vi "United-main.vi"() -> ()   [LabVIEW 2022 SP3]
doc: "Main VI for HFEPR measurements in Field domain.\nProgram uses a tab control that divides user interface in 5 pages. First (status) page is to monitor status of instruments. Second (adjustment) page is to setup individual parameters of each instrument. Third (EPR measurement) page serves for execution of measurement. Fourth (script) page serves for generation of script that can be later loaded in measurement tab. Fifth (measurement review) page is to display previous measurements. The last (about) page contains quick start info for user."
uses:
  Datatypes/Connected modules.ctl
  Datatypes/Magnet controls.ctl
  Datatypes/Application tabs.ctl
  Datatypes/Servo controls.ctl
  Datatypes/THz parameters.ctl
  Datatypes/Measurement info.ctl
  Datatypes/experiment state.ctl
  Datatypes/SampleHolders.ctl
  Datatypes/Module selection.ctl
  Datatypes/Acquisition controls.ctl
  Subsystem modules/Lock-in module/ctl/MFLI parameters.ctl
  Subsystem modules/Temperature control module/ctl/Set temperature.ctl
  Datatypes/script polymorh line.ctl
  Datatypes/Instr Info.ctl
  Subsystem modules/Magnet module/ctl/RampingOutput.ctl
  Datatypes/Single servo status.ctl
  Subsystem modules/Servo drive module/ctl/Axis names.ctl
  Datatypes/Measurement type.ctl
  Datatypes/Rotator controls.ctl
  Subsystem modules/Sample rotator/ctl/Motion Properties.ctl
  Subsystem modules/Source meter/ctls/SMU settings.ctl
  Datatypes/TopStates.ctl
  Datatypes/XY measurement graph data.ctl
  Datatypes/Measurement mode.ctl
  <vilib>/Utility/sysdir.llb/System Directory Type.ctl
  Subsystem modules/Magnet module/ctl/MSG to magnet.ctl
  Subsystem modules/Magnet module/ctl/Magnet Orders.ctl
  Subsystem modules/Magnet module/ctl/SetField data.ctl
  Subsystem modules/Magnet module/ctl/Magnet mode public.ctl
  Subsystem modules/Servo drive module/ctl/Servo MSG.ctl
  Subsystem modules/Servo drive module/ctl/Servo commands.ctl
  Subsystem modules/Sample rotator/ctl/MSG to Rotator.ctl
  Subsystem modules/Sample rotator/ctl/Rotator commands.ctl
  Subsystem modules/Sample rotator/ctl/Positoin to set.ctl
  Subsystem modules/THz module/ctl/THz Message for module.ctl
  Subsystem modules/THz module/ctl/THz commands enum.ctl
  Subsystem modules/THz module/ctl/THz sweep parameters.ctl
  Subsystem modules/Lock-in module/ctl/MFLI_message for module.ctl
  Subsystem modules/Lock-in module/ctl/MFLI_command enum.ctl
  Subsystem modules/Lock-in module/ctl/MFLI_parameter and value.ctl
  Subsystem modules/Lock-in module/ctl/MFLI_node.ctl
  Subsystem modules/Temperature control module/ctl/MSG for VTI.ctl
  Subsystem modules/Temperature control module/ctl/TC commands.ctl
  Subsystem modules/Temperature control module/ctl/Set point.ctl
  Subsystem modules/Source meter/ctls/MSG to SMU.ctl
  Subsystem modules/Source meter/ctls/SMU Commands.ctl
  Subsystem modules/THz module/ctl/THz MW generator constants.ctl
  Subsystem modules/Magnet module/ctl/TM Revision.ctl
  Subsystem modules/Magnet module/ctl/Overall status.ctl
  Subsystem modules/Magnet module/ctl/Actual magnet state.ctl
  Subsystem modules/Magnet module/ctl/Magnet mode.ctl
  Subsystem modules/Magnet module/ctl/Cryostat temperature sensors.ctl
  Subsystem modules/Power monitor/PwrM status.ctl
  Subsystem modules/Source meter/ctls/SMU status.ctl
  Subsystem modules/Lock-in module/ctl/ACQ info.ctl
  <instrlib>/Zurich Instruments LabOne/Public/Data/ziTypeDemodSampleSingle.ctl
  <instrlib>/Zurich Instruments LabOne/Public/ziTypeHandle.ctl
  Subsystem modules/Temperature control module/ctl/TC sensors.ctl
  Subsystem modules/Servo drive module/ctl/Servo state.ctl
  Subsystem modules/Servo drive module/ctl/Servo variables.ctl
  Subsystem modules/Servo drive module/ctl/Servo constants.ctl
  Subsystem modules/Servo drive module/ctl/Status variable change.ctl
  Subsystem modules/Sample rotator/ctl/Rotator all.ctl
  Subsystem modules/Sample rotator/ctl/Axis status.ctl
  <vilib>/Utility/error.llb/Trim Whitespace One-Sided.vi
  Subsystem modules/Messenger service/MessengerLib.lvlib
  Subsystem modules/Magnet module/Magnet module.lvlib
  Subsystem modules/Servo drive module/Servo drive module.lvlib
  Subsystem modules/THz module/THz source modeule.lvlib
  Subsystem modules/Lock-in module/Lock-in module.lvlib
  Subsystem modules/Sample rotator/SampleRotator.lvlib
  <instrlib>/Zurich Instruments LabOne/Zurich Instruments LabOne.lvlib
  Subsystem modules/Temperature control module/Temperature controller.lvlib
  <userlib>/_OpenG.lib/variantconfig/variantconfig.llb/openg_variant_configuration_file.lvlib
  <vilib>/Utility/config.llb/NI_LVConfig.lvlib
  Subsystem modules/Source meter/Source meter.lvlib
  Subsystem modules/Power monitor/Power monitor.lvlib
panel:
  out "Instr status":T1 caption="Connected\ninstuments"
  out "Controls referencies":T2
  out "Tmp [K]":T3
  out "Busy":bool
  in  "Stop":bool
  out "Results":T5(array[cluster])
  out "Magnetic\nfield state":bool
  out "data time":timestamp
  out "New data":bool
  out "Data":dbl[](array[numeric])
  out "Instr control refs":refnum<vi>[](array[refnum])
  out "meas results":refnum<file>
  out "Tmp reched time":dbl format="%<%H:%M:%S>T"
  out "VTI tmp reached":bool
  out "Running experiment":bool
  out "Temperature log ref":refnum<file>
  out "round execution\ntime [ms]":u32
  out "loggersRef":refnum<file>
  in  "Tab Control":T6
  out "Drift[K/s]":dbl[](array[numeric])
  in  "Log folder":path=path "C:/HFEPR logs"
  in  "Disconnect":bool
  in  "Select module":T7
  out "Logger":string[](array[string])
  in  "Re-connect instruments":bool
  in  "System config file path":path=path "C:/Programs/Debug/HFEPR spectrometer SW 2024/Multi-HFEPR app/SystemData/config.ini"
  out "Instr info":T8 {"PwrMonitor"."Last update" format="%<%H:%M:%S>T"; "VTI"."Last update" format="%<%H:%M:%S>T"; "PMD"."Last update" format="%<%H:%M:%S>T"; "SMU"."Last update" format="%<%H:%M:%S>T"; "Servo"."Last update" format="%<%H:%M:%S>T"; "Rotator"."Axes"."Actuator" items=["Linear", "Roatator", "Goniometer"]; "Rotator"."Name" items=["ANC350res", "ANC350num", "ANC350fps", "Unknown"]; "Rotator"."Last update" format="%<%H:%M:%S>T"; "THz"."Last update" format="%<%H:%M:%S>T"; "MFLI"."Last update" format="%<%H:%M:%S>T"; "Magnet"."Last update" format="%<%H:%M:%S>T"}
  in  "Use previous settings":bool=TRUE
  out "Temperature monitor":T12(graph)
  in  "Operation mode":bool=TRUE
  in  "SMU controls":T14={"Apply"=FALSE, "Measurement settings"={"Source Mode "=1, "Source Level"=0.1, "Source Limit"=0.21, "Measure Function"=0, "Remote sense"=TRUE, "Clear buffer?"=FALSE, "Beep"=TRUE, "High Capacity"=TRUE, "Terminals"=1, "PLCs"=4.0, "Fast measurement"=TRUE}, "Value"=0.1006, "Stop"=FALSE, "Record"=FALSE, "B[T]"=0.0, "Refresh"=FALSE} {"Value" format="%#_3e"; "Measurement settings"."Measure Function" items=["Volts", "Current", "Auto Resistance", "Manual Resistance", "Digitize Voltage", "Digitize Current"]; "Measurement settings"."Source Level" max=0.3; "Measurement settings"."Source Mode" items=["Voltage", "Current"]; "Measurement settings"."Terminals" items=["Front", "Rear"]}
  in  "Piezo controls":T15 {"Axes properties"."Amplitude [V]" min=0.0 max=60.0 step=1.0; "Axes properties"."DC voltage [V]" min=0.0 max=60.0 step=1.0; "Axes properties"."MaxErr [µm|m°]" min=1.0 max=1000.0 step=1.0; "Axes properties"."Frequency [Hz]" min=0.1 max=5000.0 step=10.0}
  in  "Password":string
  in  "VTI control":T17={"VTI space [K]"=1.0, "Sample [K]"=0.0, "Heater3 [K]"=1.8, "Heater4 [K]"=1.8, "Out 1 [%]"=0.0, "Out 2 [%]"=0.0, "Range out 1"=0} {"Range out 1" items=["Off", "Range 1 (On)", "Range 2", "Range 3", "Range 4", "Range 5"]; "Heater4 [K]" min=1.8 max=300.0; "Heater3 [K]" min=1.8 max=300.0; "Sample [K]" min=1.8 max=300.0; "VTI space [K]" min=1.8 max=300.0}
  in  "Acquisition controls":T18={"ACQ parameters"={"Filter order"=7.0, "Filter tau [ms]"=10.0, "F_Mod [kHz]"=1.0, "Amp_Mod [mV]"=10.0, "Enable output"=0, "Phase [°]"=0.0}, "ACQ shot btn"=FALSE, "Modulation [A]"=0.0, "In50"=FALSE, "Out50"=FALSE, "DemEn"=FALSE, "Actual [G]"=0.0, "Sample holder"=enum."Simple", "Desired [G]"=0.0, "Adj mod"=FALSE, "Auto-modulation"=TRUE, "Autorange"=FALSE, "AuxIn0 [V]"=0.0, "AuxIn1 [V]"=0.0} {"AuxIn1 [V]" format="%#_3g"; "AuxIn0 [V]" format="%#_3g"; "Desired [G]" format="%.1g"; "ACQ parameters"."Enable output" items=["Disable", "Enable"]; "ACQ parameters"."Amp_Mod [mV]" min=0.0 max=10000.0; "ACQ parameters"."F_Mod [kHz]" min=0.1 max=500.0; "ACQ parameters"."Filter order" min=1.0 max=9.0 step=1.0; "ACQ parameters"."Filter tau [ms]" min=0.0 max=1000.0}
  in  "THz control":T21={"AMC"=9, "Multip"=1, "Base frequency [GHz]"=82.0, "End frequency [GHz]"=0.0, "Im frequency [MHz]"=1885.0, "Sweep up [ms]"=0.0, "Reset trigger?"=FALSE} {"Multip" items=["1"=1, "2"=2, "3"=3, "4"=4, "6"=6, "8"=8, "9"=9]; "AMC" items=["9"=9, "12"=12]; "Base frequency [GHz]" format="%_5g"}
  in  "Servo controls":T22={"Y left"=FALSE, "Y right"=FALSE, "X backward"=FALSE, "X forward"=FALSE, "Zdown"=FALSE, "Zup"=FALSE, "Step\n[mm]"=5.0, "QO table"={"ZLdown"=FALSE, "ZLup"=FALSE, "ZRup"=FALSE, "ZRdown"=FALSE, "ZMdown"=FALSE, "ZMup"=FALSE}, "X"=0.0, "Y"=0.0, "ZL"=0.0, "ZR"=0.0, "ZM"=0.0, "Measure Position btn"=FALSE, "Eject position btn"=FALSE, "Stop servo btn"=FALSE, "Save position btn"=FALSE} {"Step\n[mm]" min=0.0 max=10.0 step=0.25}
  in  "Magnet controls":T23 {"Output\n[T]" scale=0.0..16.0; "Field\n[T]" scale=0.0..16.0; "Desired ramp\nrate [mT/s]" max=7.545; "Set Field [T]" min=0.0 max=16.0}
  out "lookup":cluster{"X (Vrms)":dbl, "Y (Vrms)":dbl}(graph) caption="Waveform Chart - Dark"
  in  "Create folder with date":bool
  in  "Operator":string
  in  "Save also backup":bool
  in  "Main data folder":path
  in  "Global comment":string
  in  "Sample name":string="Unknown"
  in  "Run script btn":bool
  in  "Direct stop meas. btn":bool
  out "Infobar":T24 {"Started" format="%<%H:%M:%S>T"; "Remains" format="%<%H:%M:%S>t"}
  out "Spectrum":cluster{dbl[], dbl[]}[](graph) caption="Live spectrum"
  in  "Paste from Editor":bool
  out "Actual measurement":T26={"Start"=nan, "Start Caption"="Start [T]", "End"=0.0, "End Caption"="End [T]", "Sweep"=0.0, "Sweep caption"="Rate [mT/s]", "Constant"=0.0, "Constant caption"="Freq [GHz]", "Mod_F [kHz]"=0.0, "Mod_A [G]"=0.0, "Tau [ms]"=0.0, "Positioners [mm|°]"=[], "Tmp [K]"=50.0, "Wait [min]"=0.0, "Carousel"=-1, "Comment"="", "Auto-mod"=TRUE, "Execute"=FALSE} {"Carousel" items=["0", "1", "2", "3", "4", "5", "6"]; "Positioners [mm|°]" min=-1.0 max=330.0; "Tau [ms]" min=0.002 max=10000.0; "Wait [min]" min=0.0 max=3000.0; "Tmp [K]" min=0.0 max=350.0; "Mod_A [G]" min=0.0 max=100.0; "Mod_F [kHz]" min=0.1 max=150.0}
  in  "Script Array":T26[](array[typedef]) {"Carousel" items=["0", "1", "2", "3", "4", "5", "6"]; "Positioners [mm|°]" min=-1.0 max=330.0; "Tau [ms]" min=0.002 max=10000.0; "Wait [min]" min=0.0 max=3000.0; "Tmp [K]" min=0.0 max=350.0; "Mod_A [G]" min=0.0 max=100.0; "Mod_F [kHz]" min=0.1 max=150.0}
  in  "Generator options":T27={"Tmp step [K]"=0.0, "Position [mm|°]"=[], "Freq step [GHz]"=0.0, "Append"=TRUE, "Iterate"=0}
  in  "Clear script btn":bool caption="Clear all script"
  in  "Set as adj tab btn":bool caption="Apply settings from\nadjustment tab"
  in  "Prototype line":T26={"Start"=0.0, "Start Caption"="Start [T]", "End"=0.0, "End Caption"="End [T]", "Sweep"=3.0, "Sweep caption"="Rate [mT/s]", "Constant"=100.0, "Constant caption"="Freq [GHz]", "Mod_F [kHz]"=3.01, "Mod_A [G]"=3.0, "Tau [ms]"=100.0, "Positioners [mm|°]"=[], "Tmp [K]"=5.0, "Wait [min]"=0.1, "Carousel"=0, "Comment"="", "Auto-mod"=TRUE, "Execute"=TRUE} {"Carousel" items=["0", "1", "2", "3", "4", "5", "6"]; "Positioners [mm|°]" min=-1.0 max=330.0; "Tau [ms]" min=0.002 max=10000.0; "Wait [min]" min=0.0 max=3000.0; "Tmp [K]" min=0.0 max=350.0; "Mod_A [G]" min=0.0 max=100.0; "Mod_F [kHz]" min=0.1 max=150.0}
  in  "Paste from meeasurrement":bool
  in  "Save script file btn":bool
  in  "Generate Script btn":bool caption="Generate Script"
  in  "Edited script":T26[](array[typedef]) caption="Script file name:" {"Carousel" items=["0", "1", "2", "3", "4", "5", "6"]; "Positioners [mm|°]" min=-1.0 max=330.0; "Tau [ms]" min=0.002 max=10000.0; "Wait [min]" min=0.0 max=3000.0; "Tmp [K]" min=0.0 max=350.0; "Mod_A [G]" min=0.0 max=100.0; "Mod_F [kHz]" min=0.1 max=150.0}
  in  "Remove from script btn":bool
  in  "Load script btn":bool
  in  "Select line":i32 min=0 max=10000
  in  "Save data btn":bool
  in  "Shift data btn":bool
  in  "Edit Channel":bool
  in  "Amlitude shift [-]":dbl
  in  "From point [T]":dbl
  out "Header":string[](array[string])
  out "Review Graph":cluster{"Array":dbl[], "Array":dbl[]}[](graph) caption="Header"
  in  "Open measurement":bool
  in  "Data file to show":u16(ring) items=["Empty", "Empty", "Empty", "Empty", "Empty", "Empty", "Empty", "Empty", "Empty", "Empty"]
  in  "Quick guide":T28(tab)
  # "Status part"
  # "Option 1:\nchoice primary and secondary sweep\n\nOption 2:\nChoice measurement mode, and appropriate cluster will apear. Other clusters wil be hidden.\n\n\nOption 3:\nChoice measurement mode.\nInternal parts of single cluster will (dis)apear if needed.\n\nNote:\nPosibility to do an orientation/temperature deppendency."
  # "Tmp [K]"
  # "Position [mm]"
  # "Z"
  # "X/Y"
  # "1.\tSelect module for subsystem, which is ready to operate. For CW measurements it is necessary to use subsystems: Magnet, VTI,\n THz sources and data acquisition (MFLI).\n2.\tClick on (Re)Connect button. Repeat for all subsystems that are ready and needed.\n3.\tWhen VTI and Magnet subsystems are connected, readings from temperature monitor and controller are displayed in graph.\n4.\tSuccessful connection to subsystem is indicated here.\n5.\tEvents on instruments are reported in this indicator.\n6.\tIf everything is OK, user may continue to another tab."
  # "1.\tFor CW experiments, magnet has to be in  ramping mode. (Magnet can be then pre-set to a start field.)\n2.\tCorrect multiplication factor need to be set manually by user.\n3.\tIntermediate frequency need to be set in in a middle of the range of band pass filters. \n4.\tTemperature of VTI can be also pre-set, while other settings are done (2 - 325 K).\n5.\tPosition of table in X axis should be about 900 mm. If table is not in measurement position, and there is no object in way, user can click on button Measure.\n6.\tIn control cluster for MFLI it is needed to enable output and set reasonable frequency and amplitude of modulation. After that click on Auto range button.\n7.\tIn case when sample rotator is used, user can check if rotator works correctly by setting desired position and press Go button.\n8.\tIn case when field sensor is used, it is required to setup current source, 100 mA, measure voltage, remote sense, rear terminals and press Apply button.\n9.\tIf series of measurement is going to be done, it is recommended to first setup measurement script in a script editor."
  # "1.\tLoad script from the Script editor tab. (overwrites current script in this tab)\n2.\tModify script if needed.\n3.\tSelect main folder, where data will be stored.\n4.\tFill name of a sample and operator that will be included in a file name.\n5.\tIf checked, save data in subfolder.\n6.\tTextbox for user to add any comment in header of data file.\n7.\tStart sequence of measurements in the script.\n8.\tContain brief information about measurement process.\n9.\tDisplays a raw spectrum.\n10.\tStop whole sequence.\n11.\tA standard graph tools."
  # "1.\tLoad actual settings of instruments and apply them to a prototype line.\n2.\tModify prototype line if needed.\n3.\tSet step for one (or more) parameter, and number of iterations.\n4.\tIf checked, append to a current scrip; else, overwrites.\n5.\tSave current script into text file (structured as configuration file) to load it later.\n6.\tModify generated script or manually fill a next line."
  # "1.\tLoad data from a file.\n2.\tRing for switching to previously loaded data.\n3.\tStandard graph tools (zoom, cursor).\n4.\tFeature to apply a simple data correction."
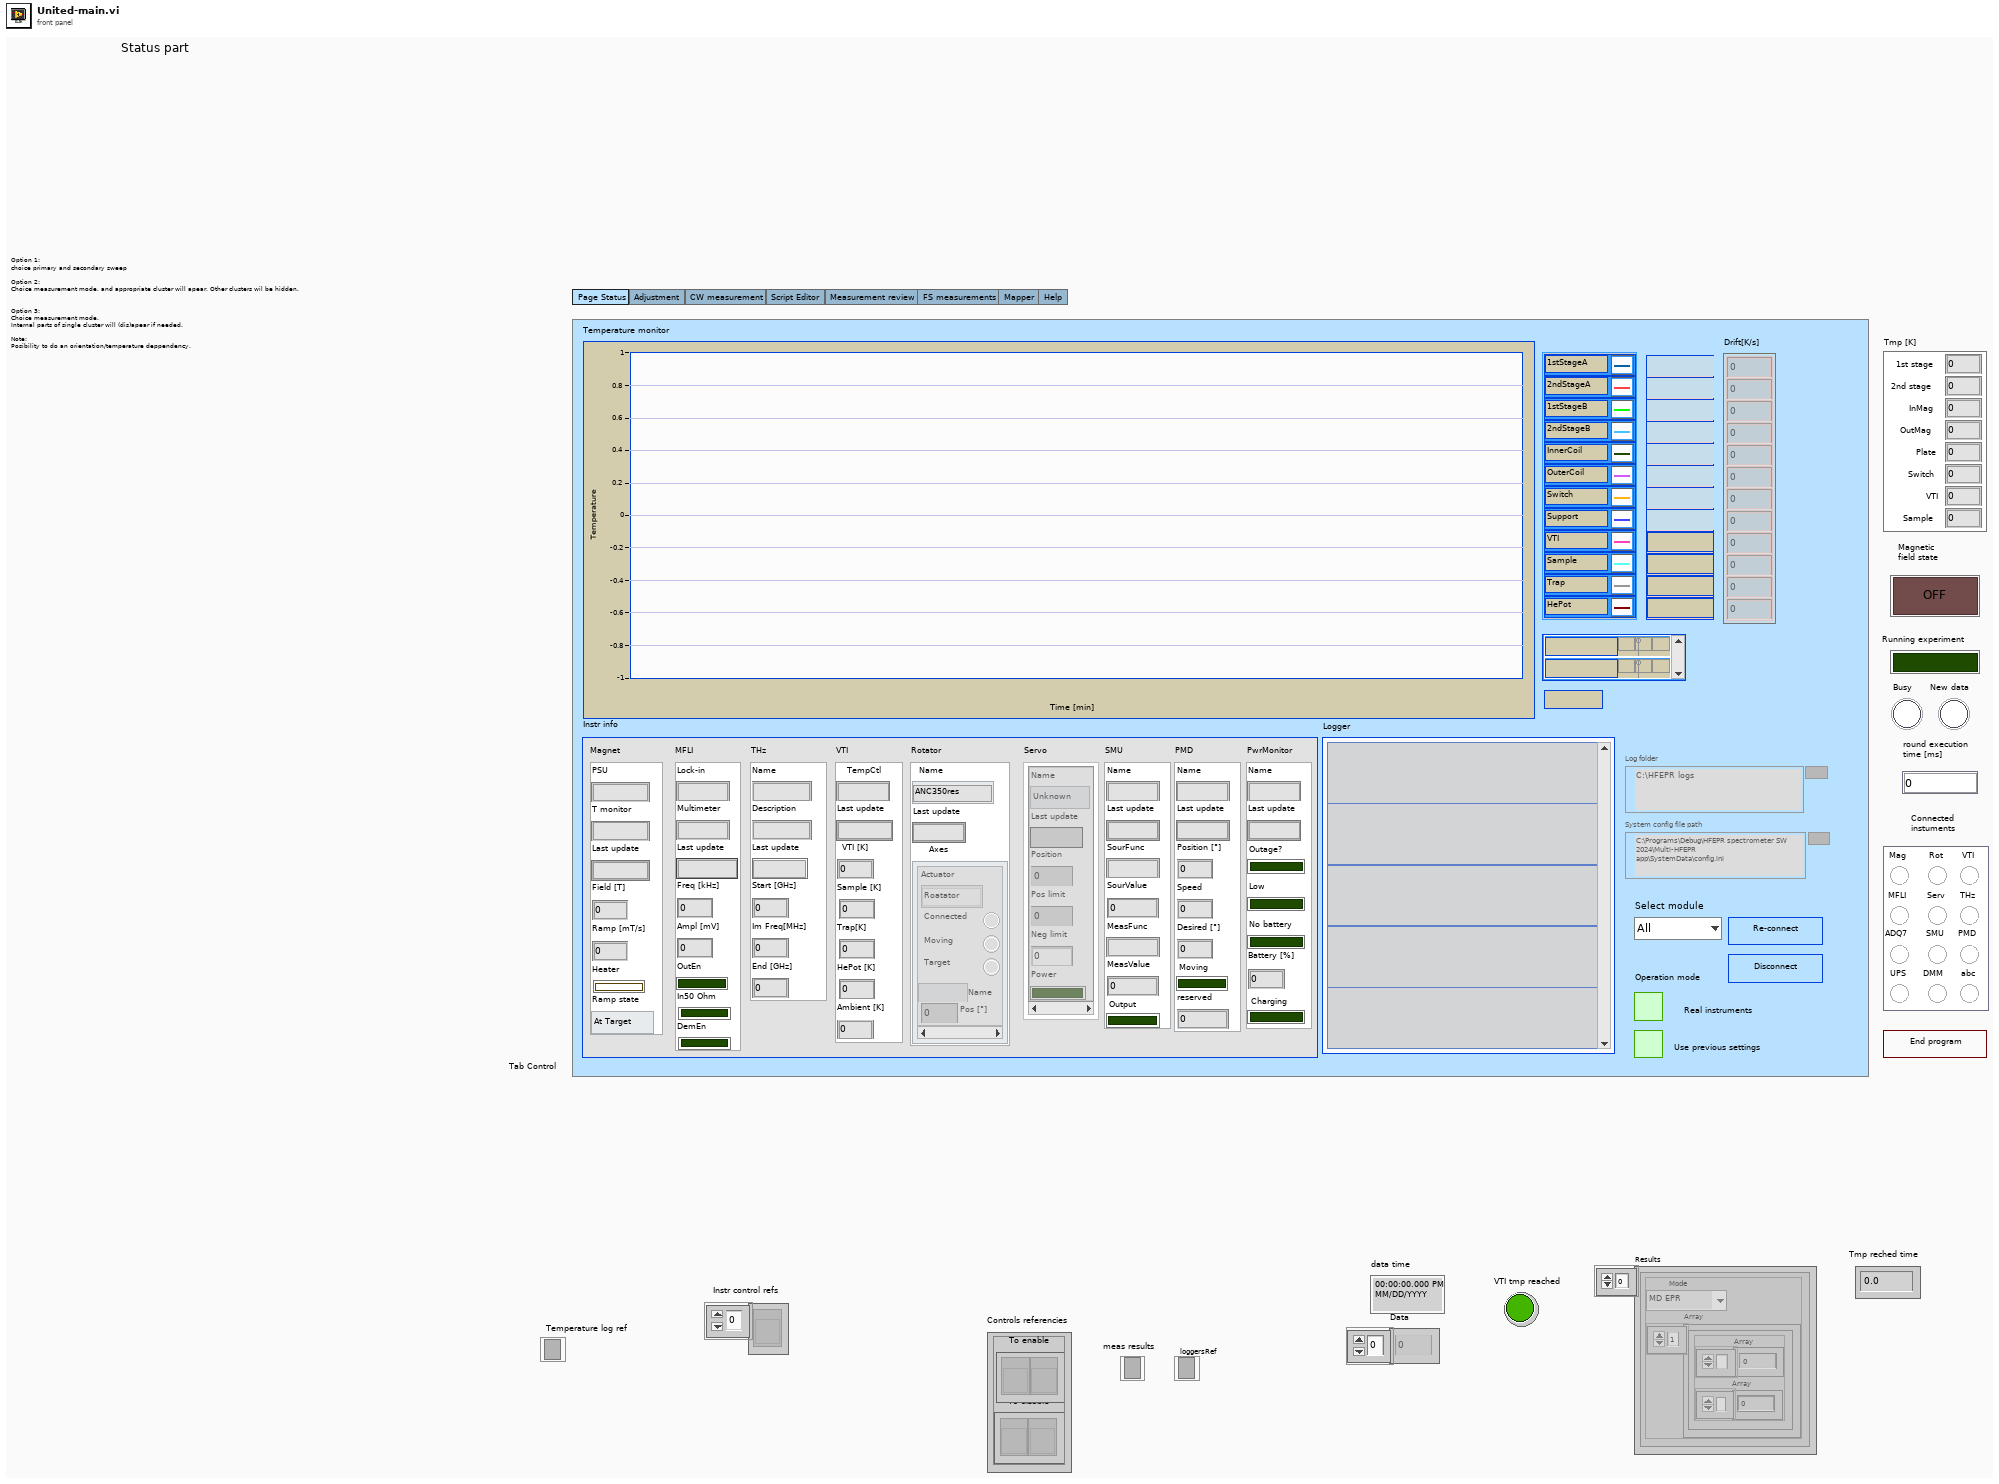
[diagram p1: front panel]
types:
  T1 = typedef "Connected modules.ctl" = cluster{"Mag":bool, "Rot":bool, "VTI":bool, "MFLI":bool, "Serv":bool, "THz":bool, "ADQ7":bool, "SMU":bool, "PMD":bool, "UPS":bool, "DMM":bool, "abc":bool}
  T2 = cluster{"To disable":refnum<vi>[], "To enable":refnum<vi>[]}
  T3 = cluster{"1st stage":dbl, "2nd stage":dbl, "InMag":dbl, "OutMag":dbl, "Plate":dbl, "Switch":dbl, "VTI":dbl, "Sample":dbl}
  T4 = typedef "Measurement type.ctl" = enum16{"MD EPR", "FD EPR"}
  T5 = cluster{"Mode":T4, "Array":cluster{"Array":dbl[], "Array":dbl[]}[]}[]
  T6 = typedef "Application tabs.ctl" = enum32{"Page Status", "Adjustment", "CW measurement", "Script Editor", "Measurement review", "FS measurements", "Mapper", "Help"}
  T7 = typedef "Module selection.ctl" = enum16{"All", "None", "ACQ", "THz", "MAG", "SERV", "ROT", "VTI", "SMU", "ADQ7", "PMD"}
  T8 = typedef "Instr Info.ctl" = cluster{"Magnet":cluster{"PSU":string, "T monitor":string, "Last update":timestamp, "Field [T]":dbl, "Ramp [mT/s]":dbl, "Heater":bool, "Ramp state":T9}, "MFLI":cluster{"Lock-in":string, "Multimeter":string, "Last update":timestamp, "Freq [kHz]":dbl, "Ampl [mV]":dbl, "OutEn":bool, "In50 Ohm":bool, "DemEn":bool}, "THz":cluster{"Name":string, "Description":string, "Last update":timestamp, "Start [GHz]":dbl, "Im Freq[MHz]":dbl, "End [GHz]":dbl}, "VTI":cluster{"TempCtl":string, "Last update":timestamp, "VTI [K]":dbl, "Sample [K]":dbl, "Trap[K]":dbl, "HePot [K]":dbl, "Ambient [K]":dbl}, "Rotator":cluster{"Name":i32, "Last update":timestamp, "Axes":cluster{"Pos [°]":dbl, "Moving":bool, "Name":string, "Actuator":u16, "Target":bool, "Connected":bool}[]}, "Servo":T10[], "SMU":cluster{"Name":string, "Last update":timestamp, "SourFunc":string, "SourValue":dbl, "MeasFunc":string, "MeasValue":dbl, "Output":bool}, "PMD":cluster{"Name":string, "Last update":timestamp, "Position [°]":dbl, "Speed":dbl, "Desired [°]":dbl, "Moving":bool, "reserved":dbl}, "PwrMonitor":cluster{"Name":string, "Last update":timestamp, "Outage?":bool, "Low":bool, "No battery":bool, "Battery [%]":u8, "Charging":bool}}
  T9 = typedef "Magnet module.lvlib/RampingOutput.ctl" = enum16{"At Target", "Go up", "Go down"}
  T10 = typedef "Single servo status.ctl" = cluster{"Name":T11, "Last update":timestamp, "Position":dbl, "Pos limit":dbl, "Neg limit":dbl, "Power":bool}
  T11 = typedef "Servo drive module.lvlib/Axis names.ctl" = enum16{"Unknown", "AxisX", "AxisY", "AxisZ_left", "AxisZ_middle", "AxisZ_right"}
  T12 = cluster{"[0]":dbl, "[1]":dbl, "[2]":dbl, "[3]":dbl, "[4]":dbl, "[5]":dbl, "[6]":dbl, "[7]":dbl, "[8]":dbl, "[9]":dbl, "[10]":dbl, "[11]":dbl}
  T13 = typedef "SMU settings.ctl" = cluster{"Source Mode ":u16, "Source Level":dbl, "Source Limit":dbl, "Measure Function":u16, "Remote sense":bool, "Clear buffer?":bool, "Beep":bool, "High Capacity":bool, "Terminals":u16, "PLCs":dbl, "Fast measurement":bool}
  T14 = cluster{"Apply":bool, "Measurement settings":T13, "Value":dbl, "Stop":bool, "Record":bool, "B[T]":dbl, "Refresh":bool}
  T15 = typedef "Rotator controls.ctl" = cluster{"Axes properties":T16[], "Rot set properties btn":bool, "Rot set position btn":bool, "Stop btn":bool, "Safe to \nmove?":bool}
  T16 = typedef "Motion Properties.ctl" = cluster{"Frequency [Hz]":dbl, "MaxErr [µm|m°]":dbl, "DC voltage [V]":dbl, "Amplitude [V]":dbl, "Position [mm|°]":dbl, "EoF":bool, "EoB":bool, "Error":bool, "Target [mm|°]":dbl}
  T17 = typedef "Temperature controller.lvlib/Set temperature.ctl" = cluster{"VTI space [K]":dbl, "Sample [K]":dbl, "Heater3 [K]":dbl, "Heater4 [K]":dbl, "Out 1 [%]":dbl, "Out 2 [%]":dbl, "Range out 1":u16}
  T18 = typedef "Acquisition controls.ctl" = cluster{"ACQ parameters":T19, "ACQ shot btn":bool, "Modulation [A]":dbl, "In50":bool, "Out50":bool, "DemEn":bool, "Actual [G]":dbl, "Sample holder":T20, "Desired [G]":dbl, "Adj mod":bool, "Auto-modulation":bool, "Autorange":bool, "AuxIn0 [V]":dbl, "AuxIn1 [V]":dbl}
  T19 = typedef "Lock-in module.lvlib/MFLI parameters.ctl" = cluster{"Filter order":dbl, "Filter tau [ms]":dbl, "F_Mod [kHz]":dbl, "Amp_Mod [mV]":dbl, "Enable output":u16, "Phase [°]":dbl}
  T20 = typedef "SampleHolders.ctl" = enum16{"Simple", "Carousel", "Chip", "Rotator", "Liquid"}
  T21 = typedef "THz parameters.ctl" = cluster{"AMC":u16, "Multip":u16, "Base frequency [GHz]":dbl, "End frequency [GHz]":dbl, "Im frequency [MHz]":dbl, "Sweep up [ms]":dbl, "Reset trigger?":bool}
  T22 = typedef "Servo controls.ctl" = cluster{"Y left":bool, "Y right":bool, "X backward":bool, "X forward":bool, "Zdown":bool, "Zup":bool, "Step\n[mm]":dbl, "QO table":cluster{"ZLdown":bool, "ZLup":bool, "ZRup":bool, "ZRdown":bool, "ZMdown":bool, "ZMup":bool}, "X":dbl, "Y":dbl, "ZL":dbl, "ZR":dbl, "ZM":dbl, "Measure Position btn":bool, "Eject position btn":bool, "Stop servo btn":bool, "Save position btn":bool}
  T23 = typedef "Magnet controls.ctl" = cluster{"Set Field [T]":dbl, "Desired ramp\nrate [mT/s]":dbl, "Custom\nramp":bool, "Mode switch":bool, "Pause ramp":bool, "Field\n[T]":dbl, "Output\n[T]":dbl, "Equalize":bool, "Discharge":bool, "Switch \ntmp [K]":dbl, "Direction":bool}
  T24 = typedef "Measurement info.ctl" = cluster{"Remains":dbl, "T_sample [K]":dbl, "Last log":string, "Experiment state":T25, "Field [T]":dbl, "Sample holder":T20, "Started":timestamp}
  T25 = typedef "experiment state.ctl" = enum16{"Setup", "Preparation", "Stabilization", "Begin", "Acquisition", "Save"}
  T26 = typedef "script polymorh line.ctl" = cluster{"Start":dbl, "Start Caption":string, "End":dbl, "End Caption":string, "Sweep":dbl, "Sweep caption":string, "Constant":dbl, "Constant caption":string, "Mod_F [kHz]":dbl, "Mod_A [G]":dbl, "Tau [ms]":dbl, "Positioners [mm|°]":dbl[], "Tmp [K]":dbl, "Wait [min]":dbl, "Carousel":i8, "Comment":string, "Auto-mod":bool, "Execute":bool}
  T27 = cluster{"Tmp step [K]":dbl, "Position [mm|°]":dbl[], "Freq step [GHz]":dbl, "Append":bool, "Iterate":u16}
  T28 = enum32{"Status", "Adjustment", "Measurement", "Script", "Viewer"}
  T29 = typedef "TopStates.ctl" = enum16{"Initialize GUI", "Wait for Event", "Check message", "Check measurement", "Stop", "Restart"}
  T30 = typedef "MessengerLib.lvlib/Messenger referencies.ctl" = cluster{"TOP":refnum<queue>, "Instr_M":refnum<queue>, "Field_C":refnum<queue>, "Tmp_M":refnum<queue>, "Tmp_C":refnum<queue>, "Table_C":refnum<queue>, "MW_C":refnum<queue>, "Data_Aq":refnum<queue>, "Mod_M":refnum<queue>, "Field_M":refnum<queue>, "Pwr_M":refnum<queue>, "Angle_C":refnum<queue>, "Sample_C":refnum<queue>, "Reserved":refnum<queue>}
  T31 = typedef "XY measurement graph data.ctl" = cluster{"Mode":T32, "Array":cluster{"Array":dbl[], "Array":dbl[]}[]}
  T32 = typedef "Measurement mode.ctl" = enum16{"MD EPR", "FD EPR", "EDMR", "EPR MAP"}
  T33 = enum8{"Enabled", "Disabled", "Disabled and Grayed Out"}
  T34 = typedef "Magnet module.lvlib/Magnet mode public.ctl" = enum16{"Persistant", "Ramping"}
  T35 = typedef "Magnet module.lvlib/SetField data.ctl" = cluster{"Field [T]":dbl, "Ramp [T/s]":dbl, "Custom Ramp?":bool, "Mode":T34}
  T36 = typedef "Magnet module.lvlib/Magnet Orders.ctl" = enum16{"Ignore", "Connect", "Update", "Switch mode", "Set field", "Stop ramping", "Equalize output", "Zero output", "Flip polarity", "Blackout", "Set timer", "Eval temperatures", "Disconnect"}
  T37 = typedef "Magnet module.lvlib/MSG to magnet.ctl" = cluster{"Command":T36, "Data":variant}
  T38 = typedef "Servo drive module.lvlib/Servo commands.ctl" = enum16{"Initialize", "Update", "Move by", "Move to", "Stop", "Ignore", "Disconnect", "End"}
  T39 = typedef "Servo drive module.lvlib/Servo MSG.ctl" = cluster{"Command":T38, "Data":variant}
  T40 = typedef "SampleRotator.lvlib/MSG to Rotator.ctl" = cluster{"Command":T41, "Data":variant}
  T41 = typedef "SampleRotator.lvlib/Rotator commands.ctl" = enum16{"Ignore", "Initialize", "Initialize axes", "Update", "Set parameters", "Stop movement", "Set position", "Disconnect", "End"}
  T42 = typedef "Positoin to set.ctl" = cluster{"Relative?":bool, "Position [°]":dbl, "Safe to move?":bool}
  T43 = typedef "THz source modeule.lvlib/THz commands enum.ctl" = enum16{"Ignore", "Connect", "Update", "Set parameters", "Disconnect", "End"}
  T44 = typedef "THz source modeule.lvlib/THz sweep parameters.ctl" = cluster{"Start [GHz]":dbl, "End [GHz] ":dbl, "Sweep up\ntime [ms]":dbl, "Sweep down\ntime [ms]":dbl, "Intermidiate [MHz]":dbl, "Reset trigger":bool}
  T45 = typedef "THz source modeule.lvlib/THz Message for module.ctl" = cluster{"Command":T43, "Data":variant}
  T46 = typedef "Lock-in module.lvlib/MFLI_parameter and value.ctl" = cluster{"parameter":T47, "value":dbl}
  T47 = typedef "Lock-in module.lvlib/MFLI_node.ctl" = enum16{"None", "filter_order [-]", "filter_constant [ms]", "in_diff", "in_autorange", "in_imp50", "in_AC", "osc_freq [kHz]", "out_ampl [V]", "out_autorange", "out_imp50", "enable output", "enamble ampl", "scope_enable", "scope_rate", "scope_len", "scope_trigEn", "AuxOut_amplify", "Phase_deg", "AuxOut_select"}
  T48 = typedef "Lock-in module.lvlib/MFLI_command enum.ctl" = enum16{"Initialize", "Update", "Set parameters", "Set module", "Set individual parameters", "Get point", "Get array", "Disconnect", "End", "Ignore"}
  T49 = typedef "Lock-in module.lvlib/MFLI_message for module.ctl" = cluster{"Command":T48, "Data":variant}
  T50 = typedef "Temperature controller.lvlib/Set point.ctl" = cluster{"Heater":string, "Tmp [K]":dbl}
  T51 = typedef "Temperature controller.lvlib/TC commands.ctl" = enum16{"Initialize", "Update", "Stop tmp change", "Set temperature", "Set point", "Disconnect", "End", "Ignore"}
  T52 = typedef "Temperature controller.lvlib/MSG for VTI.ctl" = cluster{"Command":T51, "Data":variant}
  T53 = typedef "Source meter.lvlib/MSG to SMU.ctl" = cluster{"Command":T54, "Data":variant}
  T54 = typedef "Source meter.lvlib/SMU Commands.ctl" = enum16{"Ignore", "Connect", "Update", "Set measurement", "Start measurement", "Get actual results", "Stop measurement", "Disconnect", "End"}
  T55 = cluster{"min synth f":dbl, "max synth f":dbl, "Ramp limits [mT/s]":dbl[], "Field ranges [T]":dbl[]}
  T56 = cluster{"Mode":T4, "Array":cluster{"Array":dbl[], "Array":dbl[]}[]}
  T57 = typedef "THz source modeule.lvlib/THz MW generator constants.ctl" = cluster{"Lower limit [GHz]":dbl, "Upper limit [GHz]":dbl, "Device name":string, "Connection":string, "Description":string, "Connected":bool, "Last settings":string, "Operation mode":enum16{"Disabled", "CW", "Arbitrary", "Sweep"}, "Enable ch 1":bool, "Enable ch 2":bool}
  T58 = typedef "Magnet module.lvlib/TM Revision.ctl" = cluster{"Instr Serial Number":string, "Instr Driver Revision":string, "Instr Firmware Revision":string, "Instr Model Number":string}
  T59 = typedef "Magnet module.lvlib/Overall status.ctl" = cluster{"Desired":T35, "Actual":T60}
  T60 = typedef "Magnet module.lvlib/Actual magnet state.ctl" = cluster{"Mode":T61, "Ramping output":T9, "Ready for change":bool, "Switch heater":bool, "Cooler Overheat":bool, "Coil overheat":bool, "Energized":bool, "Output [T]":dbl, "Field [T]":dbl, "Ramp[T/s]":dbl, "Switch\ntemperature [K]":dbl, "Voltage [V]":dbl, "Current direction":bool}
  T61 = typedef "Magnet module.lvlib/Magnet mode.ctl" = enum16{"Persistant", "Switching", "Ramping", "Quenched"}
  T62 = typedef "Magnet module.lvlib/Cryostat temperature sensors.ctl" = cluster{"First stage A [K]":dbl, "Second stage A [K]":dbl, "Firs stage B [K]":dbl, "Second stage B [K]":dbl, "Inner magnet [K]":dbl, "Outer Magnet [K]":dbl, "Switch [K]":dbl, "Support plate [K]":dbl, "Time stamp":dbl}
  T63 = typedef "Power monitor.lvlib/PwrM status.ctl" = cluster{"Name":string, "Last update":timestamp, "Outage?":bool, "Low":bool, "No battery":bool, "Battery [%]":u8, "Charging":bool}
  T64 = typedef "Source meter.lvlib/SMU status.ctl" = cluster{"VISA name":refnum<visa-resource-name>, "Connected":bool, "Name":string, "Message":string, "Error message":string, "Min voltage":dbl, "Max voltage":dbl, "Min Current":dbl, "Max Current":dbl, "Measurement value":dbl, "Source Voltage":dbl, "Measurement":bool, "Source Current":dbl, "Source Mode":u16, "Measure Function":u16}
  T65 = typedef "Lock-in module.lvlib/ACQ info.ctl" = cluster{"In50":bool, "InAC":bool, "InDiff":bool, "Out50":bool, "OutEN":bool, "OutF[Hz]":dbl, "OutA[V]":dbl, "DemEN":bool, "Const[ms]":dbl, "Order[-]":i32, "Phase [°]":dbl}
  T66 = enum32{"Page Status", "Adjustment", "EPR measurement", "About"}
  T67 = typedef "Zurich Instruments LabOne.lvlib/ziTypeDemodSampleSingle.ctl" = cluster{"Timestamps (ticks)":u64, "X (Vrms)":dbl, "Y (Vrms)":dbl, "Osc Phase (deg)":dbl, "Freq (Hz)":dbl, "DIO":u32, "AuxIn0 (V)":dbl, "AuxIn1 (V)":dbl, "Trigger":u32}
  T68 = typedef "Zurich Instruments LabOne.lvlib/ziTypeHandle.ctl" = cluster{"handleValid":bool, "Conn":u64, "Path Prefix":string, "Handle":u64, "Connected":bool, "Clockbase(s)":dbl}
  T69 = typedef "Temperature controller.lvlib/TC sensors.ctl" = cluster{"VTI space":dbl, "Sample":dbl, "He pot":dbl, "Trap":dbl, "Ambient":dbl, "SetP_VTI":dbl, "SetP_Smp":dbl, "SetP_Pot":dbl, "SetP_Trap":dbl, "Range out 1":u16, "Out 1 [%]":dbl, "Out 2 [%]":dbl}
  T70 = typedef "Servo drive module.lvlib/Servo state.ctl" = cluster{"Servo variables":T71, "Servo constants":T72, "Connection":variant}
  T71 = typedef "Servo drive module.lvlib/Servo variables.ctl" = cluster{"Terget reached":bool, "Connected":bool, "Power ON":bool, "Operation mode":bool, "Actual position":dbl, "Target position":dbl}
  T72 = typedef "Servo drive module.lvlib/Servo constants.ctl" = cluster{"Name":T11, "Pos position limit [mm]":dbl, "Neg position limit [mm]":dbl, "Pos velocity limit":dbl, "Neg velocity limit":dbl, "Acceleration limit":dbl}
  T73 = typedef "Servo drive module.lvlib/Status variable change.ctl" = cluster{"Property":string, "Value":variant, "Name":T11}
  T74 = typedef "SampleRotator.lvlib/Rotator all.ctl" = cluster{"Controller info":cluster{"deviceNumber":i32, "DeviceType":i32, "ID":u32, "Serial":string, "Address":string, "connected":bool}, "Handle":u64, "FW-Version":i32, "Features":u32, "Axes":T75[], "Path to DLL":path}
  T75 = typedef "SampleRotator.lvlib/Axis status.ctl" = cluster{"Axis status":cluster{"Connected":bool, "Enabled":bool, "Moving":bool, "Target":bool, "EndForward":bool, "EndBackarwd":bool, "Error":bool}, "Position [°]":dbl, "Frequency [Hz]":dbl, "Voltage [V]":dbl, "Capacitance[uF]":dbl, "Name":string, "ActuatorType":u16, "DC offset [V]":dbl, "Tolerance [m°]":dbl, "Index":u8}
  T76 = typedef "NI_LVConfig.lvlib/Config Data RefNum.ctl" = refnum<k1>
  T77 = typedef "System Directory Type.ctl" = i32
  T78 = typedef "lveventtype.ctl" = enum32{"Null", "Timeout", "Annotation Menu Selection", "Annotation Menu Selection?", "App Instance Close", "App Instance Close?", "Autoscale Range Change", "Bookmark Info Change", "Cell Edit", "Cell Edit?", "Cursor Grab", "Cursor Grab?", "Cursor Menu Selection", "Cursor Menu Selection?", "Cursor Move", "Cursor Release", "Data Change", "Direction Change", "Display State Change", "Drag Ended", "Drag Enter", "Drag Leave", "Drag Over", "Drag Source Update", "Drag Starting", "Drag Starting?", "Drop", "Exec State Change", "Key Down", "Key Down?", "Key Repeat", "Key Repeat?", "Key Up", "Listbox Double Click", "Menu Activation?", "Menu Selection (App)", "Menu Selection? (App)", "Menu Selection (User)", "Mouse Down", "Mouse Down?", "Mouse Enter", "Mouse Leave", "Mouse Move", "Mouse Up", "Mouse Wheel", "NI Security User Change (App)", "Pane Size", "Panel Close", "Panel Close?", "Panel Resize", "Plot Attribute Change", "Scale Range Change", "Shortcut Menu Activation?", "Shortcut Menu Selection (App)", "Shortcut Menu Selection? (App)", "Shortcut Menu Selection (User)", "Tree Double Click", "Tree Drag", "Tree Drag?", "Tree Drop", "Tree Drop?", "Tree Item Close", "Tree Item Close?", "Tree Item Open", "Tree Item Open?", "User Event", "Value Change"}
  T79 = typedef "Mudules status.ctl" = cluster{"Mag":bool, "Rot":bool, "VTI":bool, "MFLI":bool, "Serv":bool, "THz":bool, "ADQ7":bool, "SMU":bool, "PMD":bool, "UPS":bool, "DMM":bool, "abc":bool}
  T80 = typedef "Magnet module.lvlib/Magnet config constants.ctl" = cluster{"Switch resistant [K]":dbl, "Switch superconducting [K]":dbl, "First stage critical temperature [K]":dbl, "Second stage critical temperature [K]":dbl, "Inner magnet critical temperature [K]":dbl, "Outer magnet critical temperature [K]":dbl, "Field Constant [T/A]":dbl, "Maximum Current [A]":dbl, "Maximum field [T]":dbl, "Maximum source ramp [A/s]":dbl, "Source precision [T]":dbl, "Ramp limits [A/s]":dbl[], "Field limits [T]":dbl[], "SMS":refnum<visa-resource-name>, "LSC218":refnum<visa-resource-name>}
  T81 = typedef "MessengerLib.lvlib/MSG to TOP.ctl" = cluster{"Module":T82, "Response":string, "Data":variant, "Time":timestamp}
  T82 = typedef "Module name.ctl" = enum16{"Emty", "Magnet", "VTI", "Excitation", "Servo", "Acquisition", "Rotator", "Digitizer", "SMU2450", "Carousel", "Multimeter", "Tmp monitor", "Power monitor"}
  T83 = cluster{"PSU":string, "T monitor":string, "Last update":timestamp, "Field [T]":dbl, "Ramp [mT/s]":dbl, "Heater":bool, "Ramp state":T9}
  T84 = cluster{"TempCtl":string, "Last update":timestamp, "VTI [K]":dbl, "Sample [K]":dbl, "Trap[K]":dbl, "HePot [K]":dbl, "Ambient [K]":dbl}
  T85 = cluster{"Name":string, "Description":string, "Last update":timestamp, "Start [GHz]":dbl, "Im Freq[MHz]":dbl, "End [GHz]":dbl}
  T86 = cluster{"Name":string, "Last update":timestamp, "Outage?":bool, "Low":bool, "No battery":bool, "Battery [%]":u8, "Charging":bool}
  T87 = cluster{"Name":string, "Last update":timestamp, "SourFunc":string, "SourValue":dbl, "MeasFunc":string, "MeasValue":dbl, "Output":bool}
  T88 = cluster{"Lock-in":string, "Multimeter":string, "Last update":timestamp, "Freq [kHz]":dbl, "Ampl [mV]":dbl, "OutEn":bool, "In50 Ohm":bool, "DemEn":bool}
  T89 = cluster{"Name":i32, "Last update":timestamp, "Axes":cluster{"Pos [°]":dbl, "Moving":bool, "Name":string, "Actuator":u16, "Target":bool, "Connected":bool}[]}
  T90 = cluster{"Pos [°]":dbl, "Moving":bool, "Name":string, "Actuator":u16, "Target":bool, "Connected":bool}[]
  T91 = cluster{"Pos [°]":dbl, "Moving":bool, "Name":string, "Actuator":u16, "Target":bool, "Connected":bool}
  T92 = cluster{"deviceNumber":i32, "DeviceType":i32, "ID":u32, "Serial":string, "Address":string, "connected":bool}
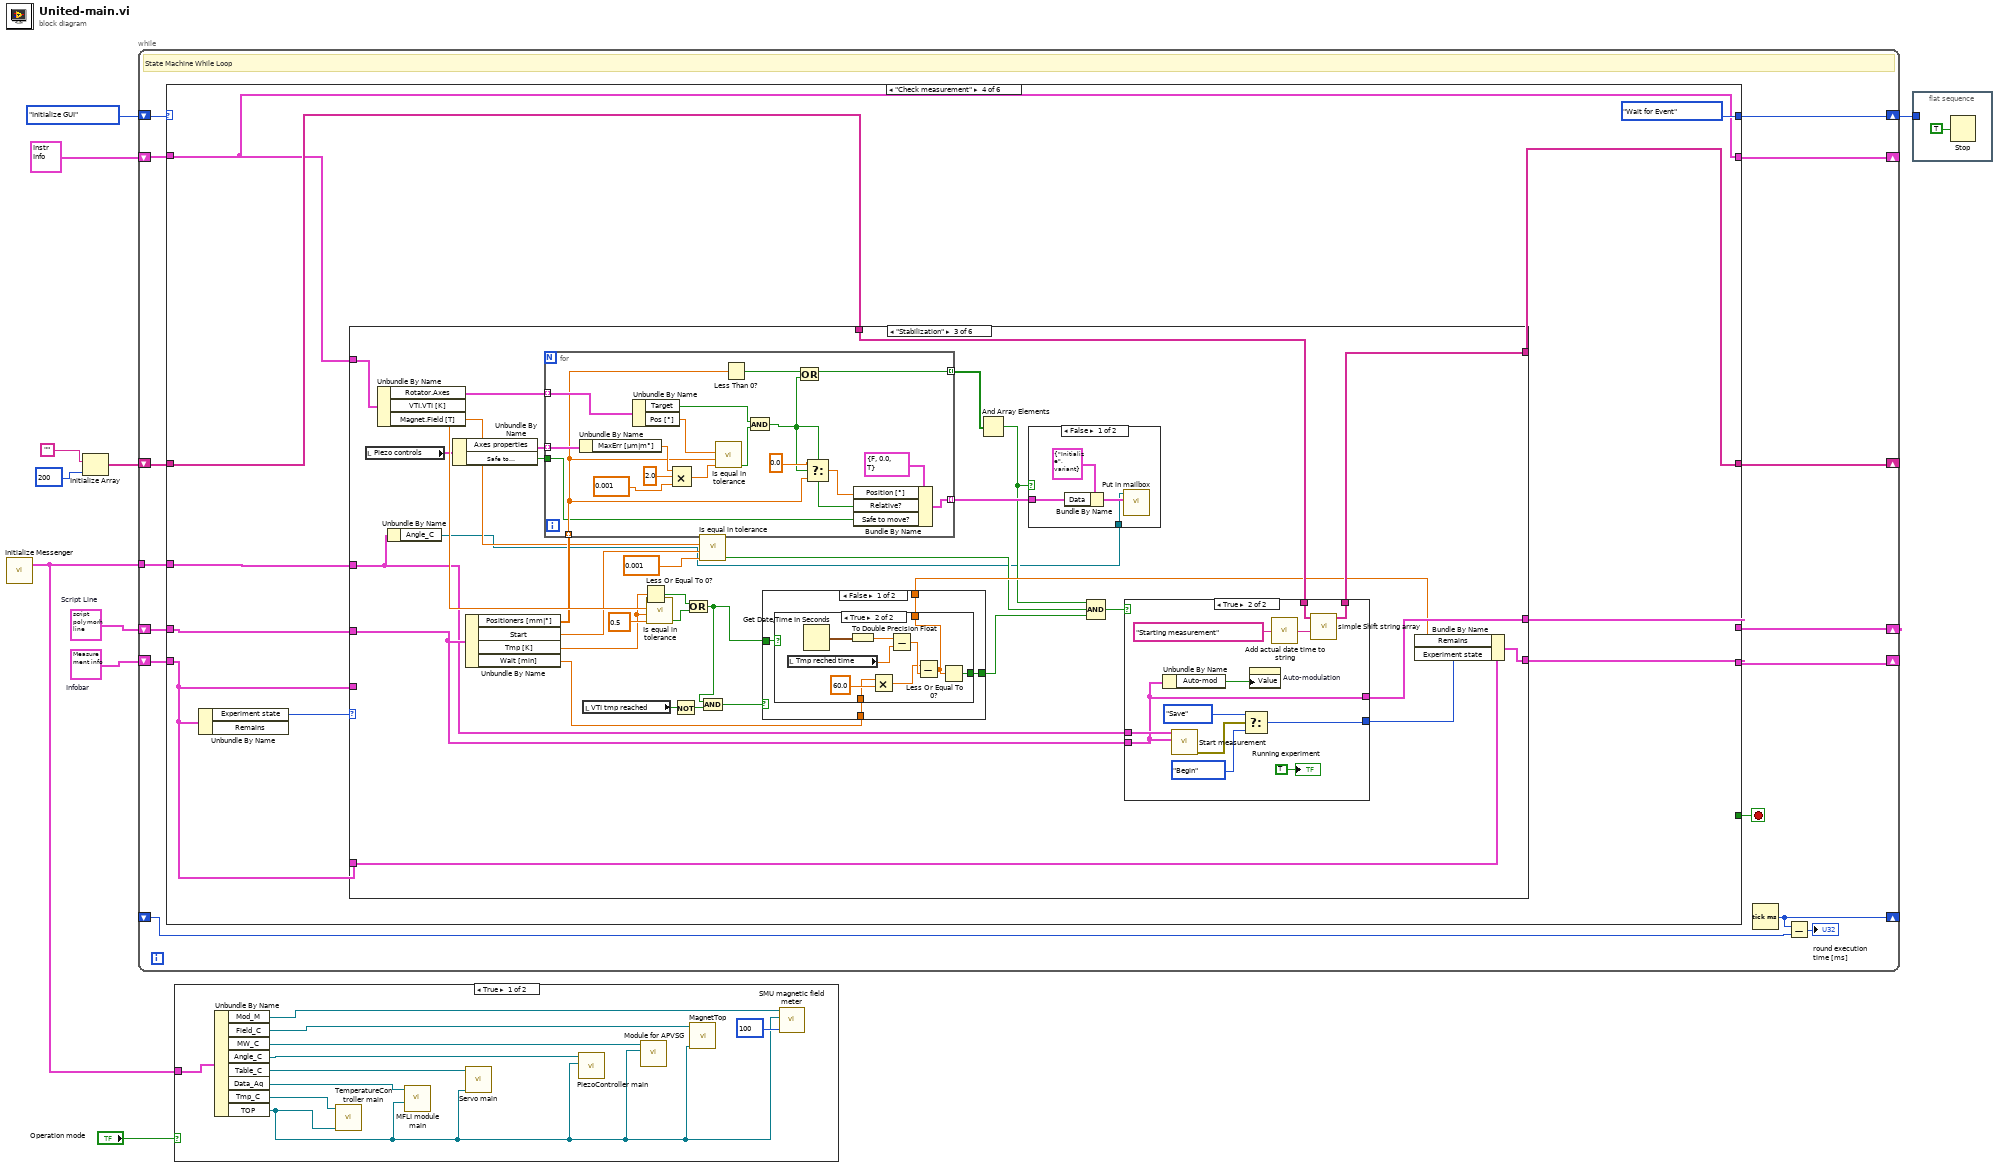
[diagram p0: block diagram]
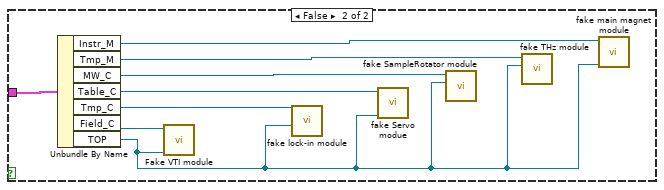
[diagram p2: hidden frame]
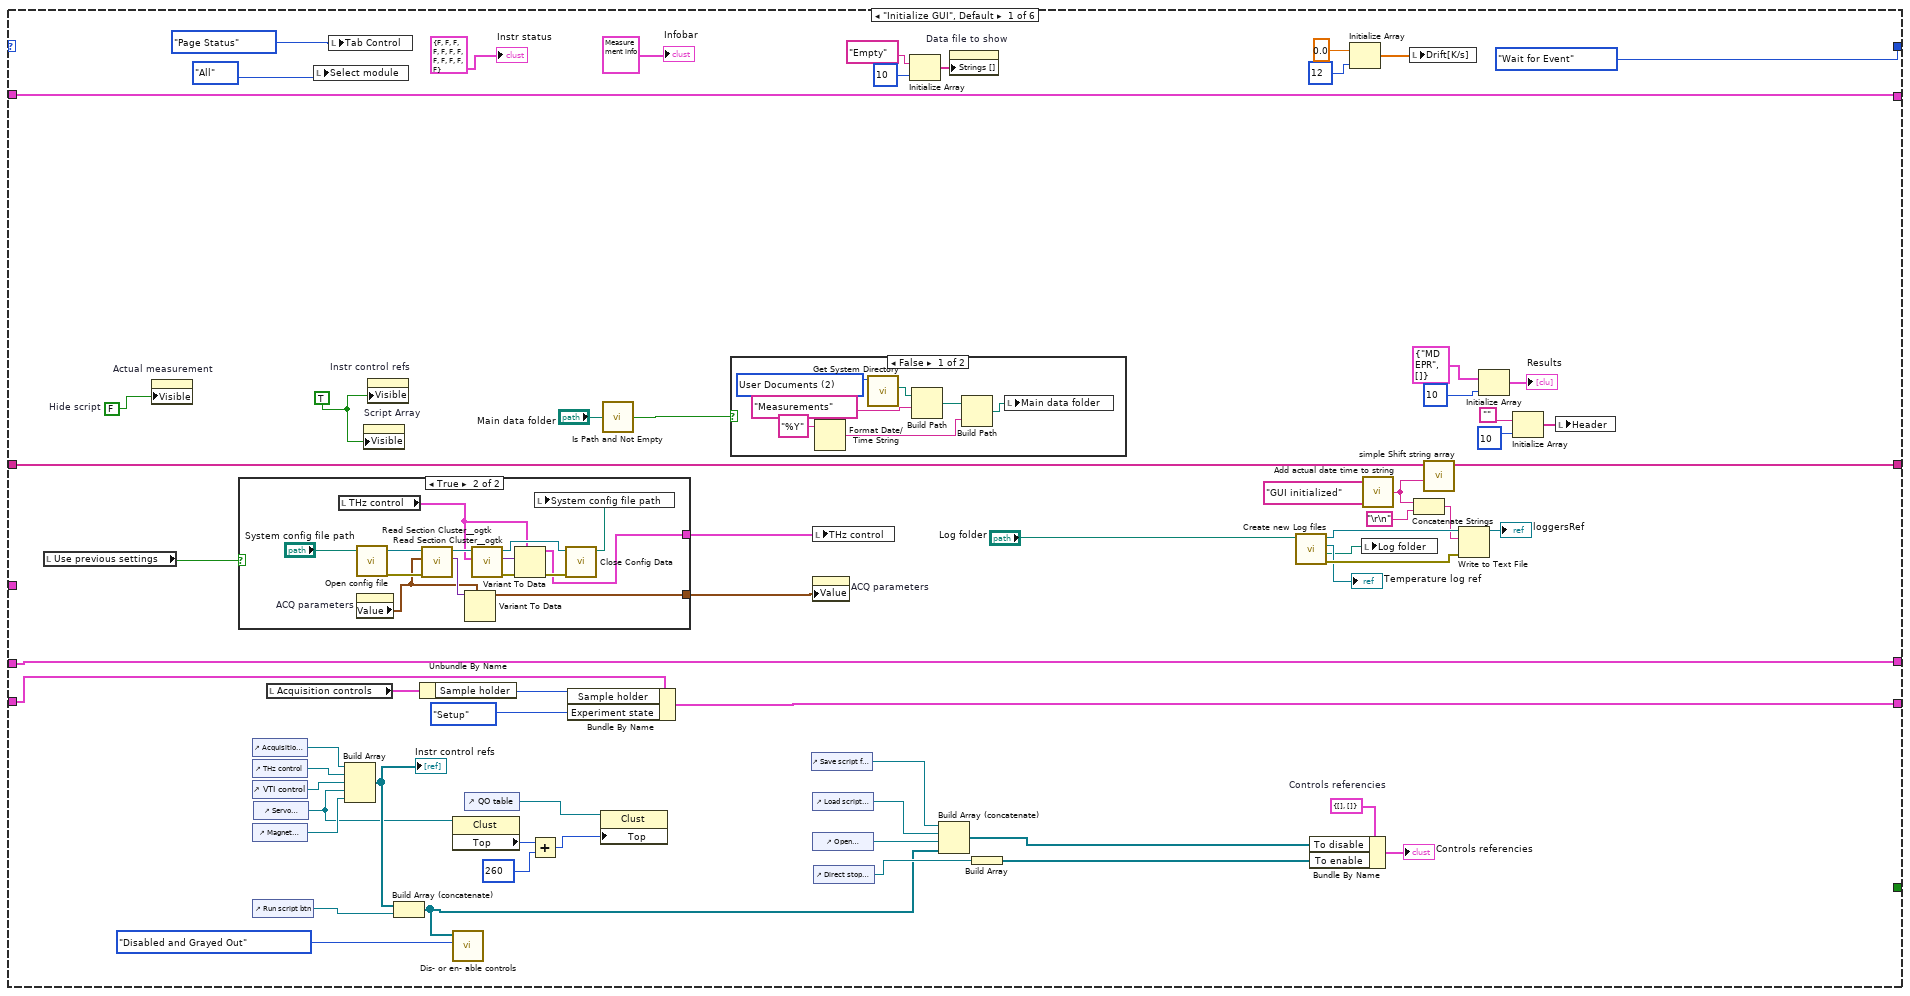
[diagram p3: hidden frame]
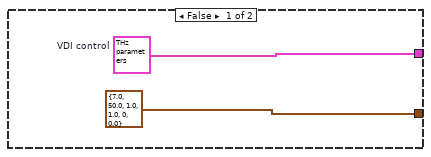
[diagram p5: hidden frame]
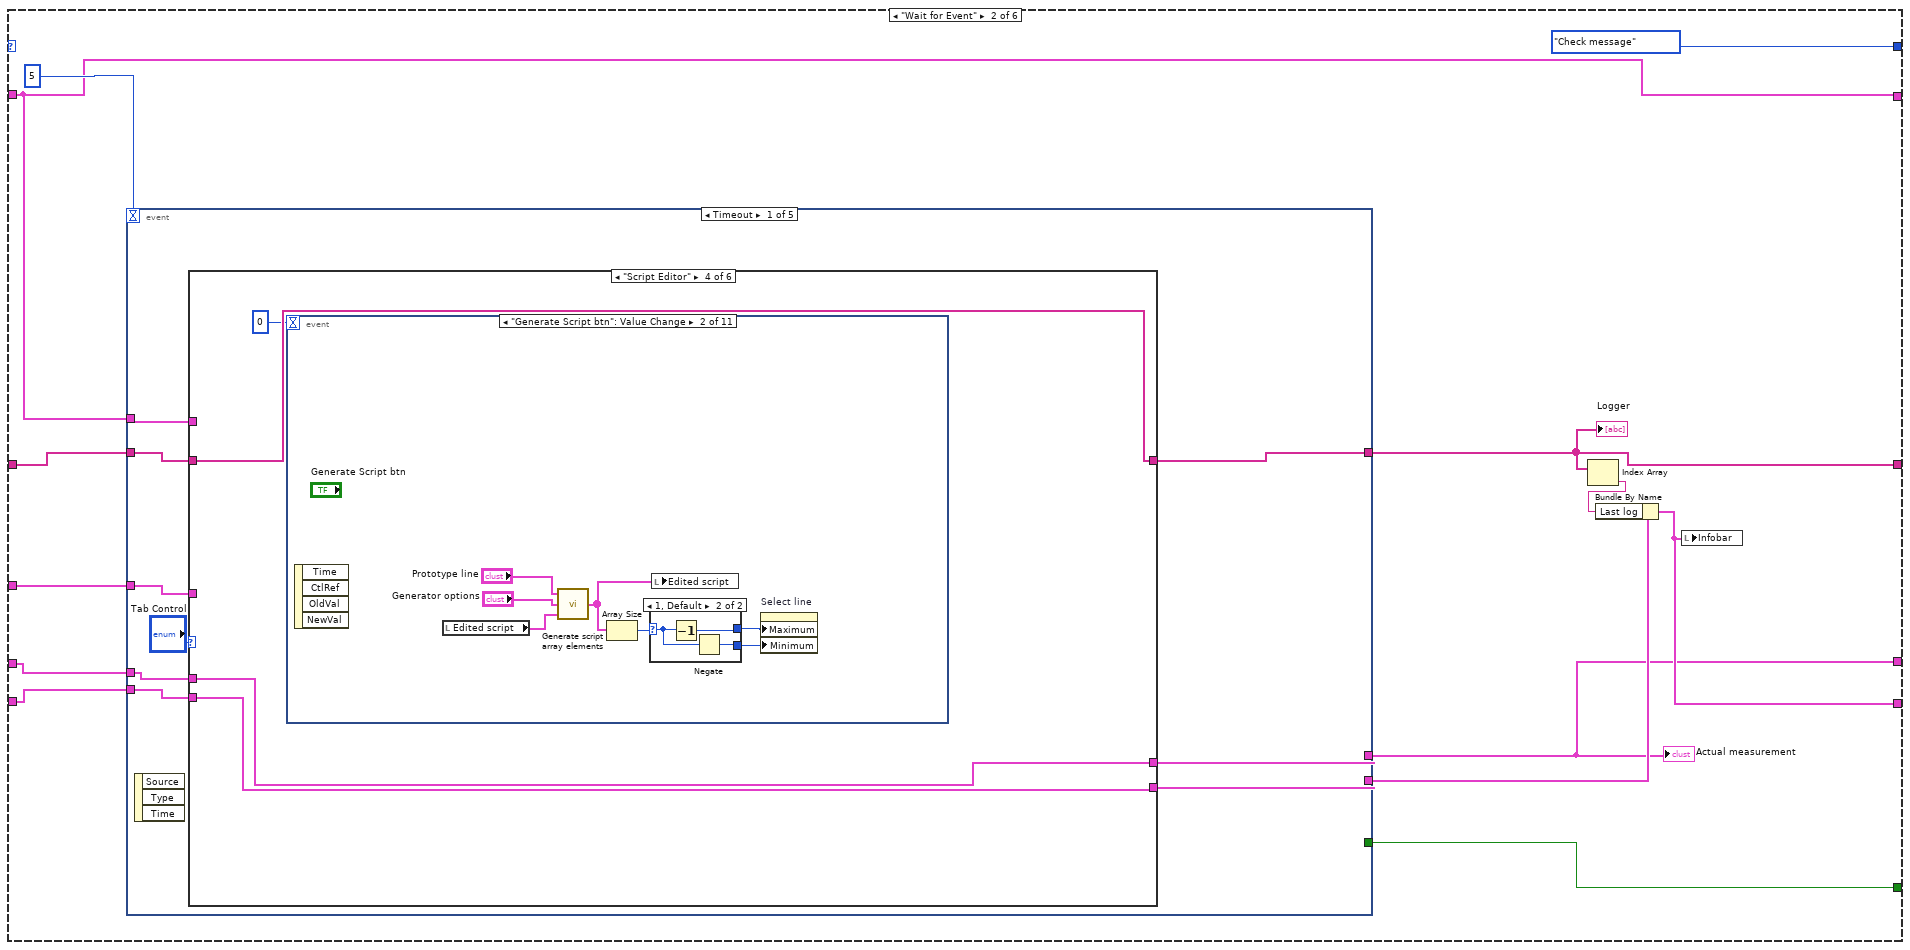
[diagram p6: hidden frame]
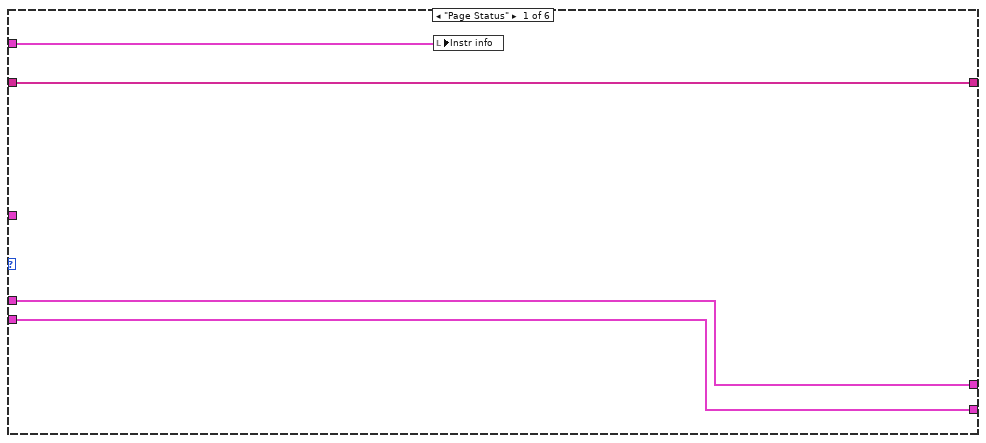
[diagram p7: hidden frame]
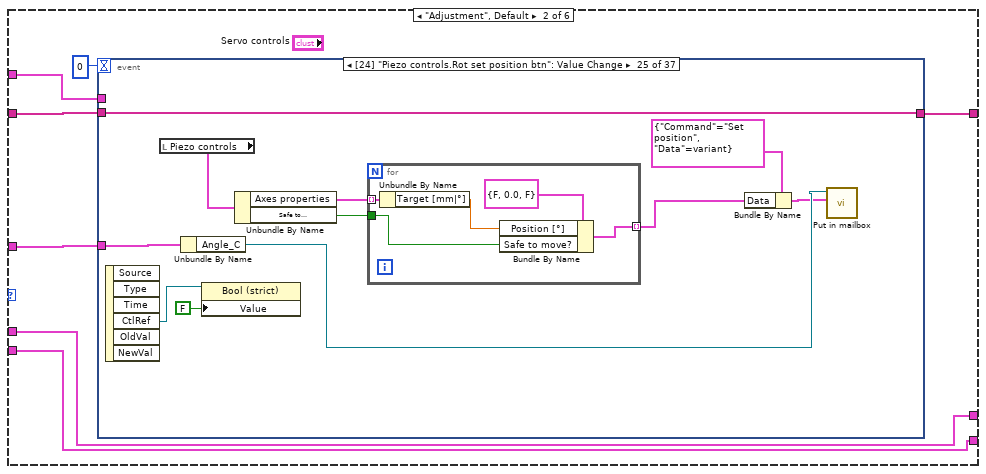
[diagram p8: hidden frame]
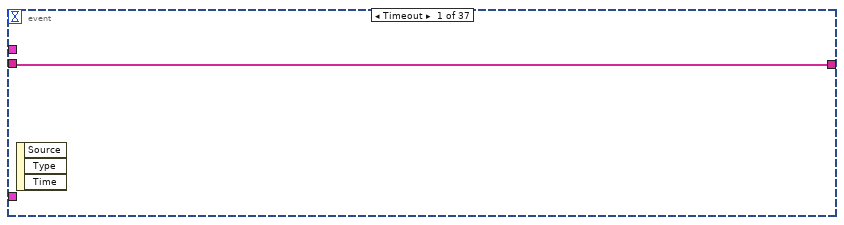
[diagram p9: hidden frame]
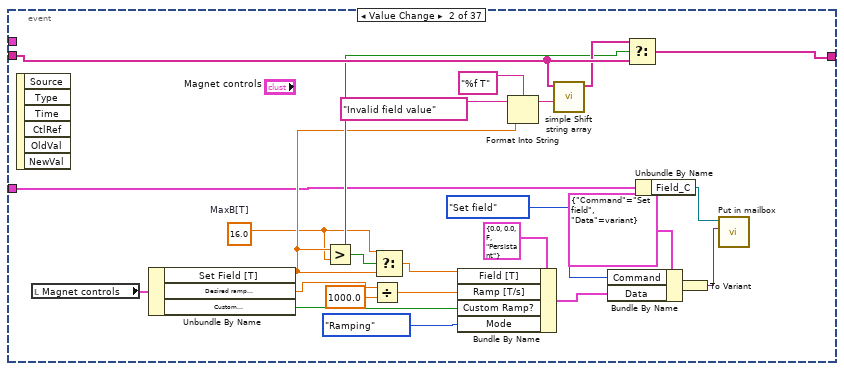
[diagram p10: hidden frame]
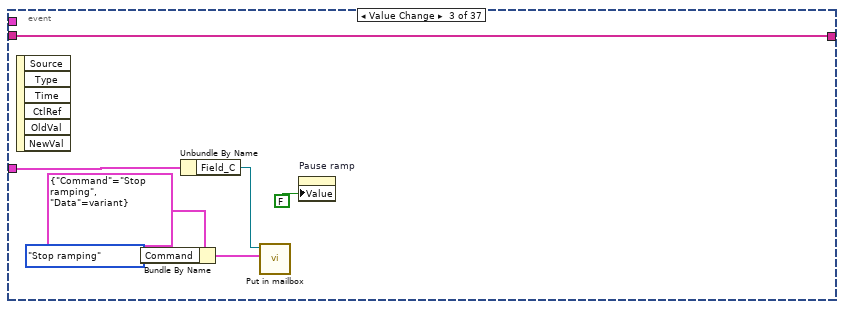
[diagram p11: hidden frame]
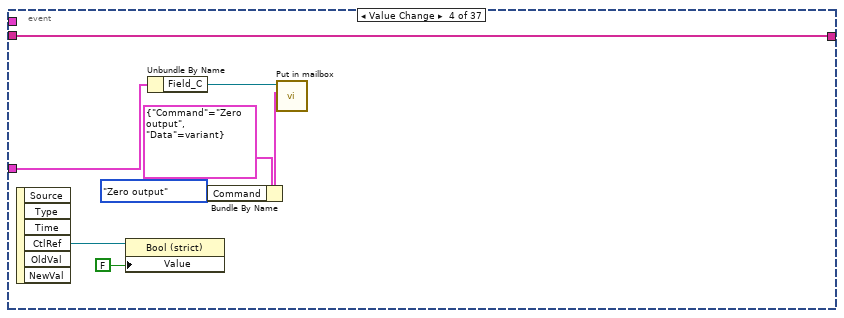
[diagram p12: hidden frame]
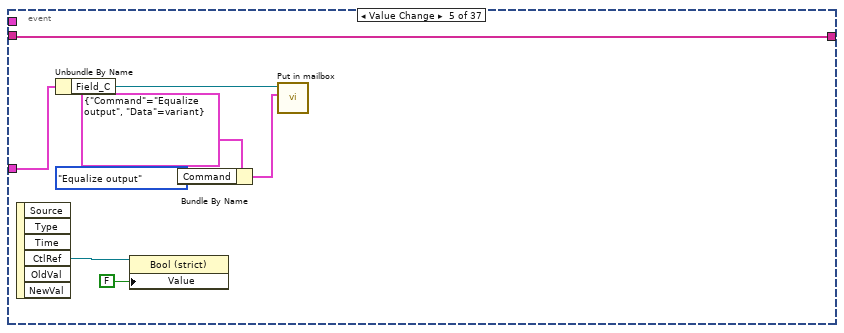
[diagram p13: hidden frame]
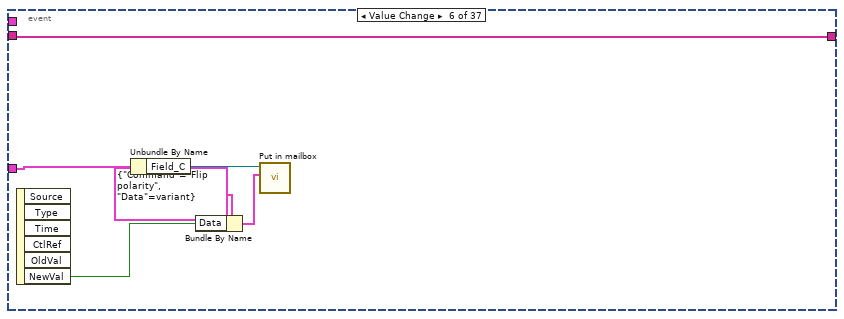
[diagram p14: hidden frame]
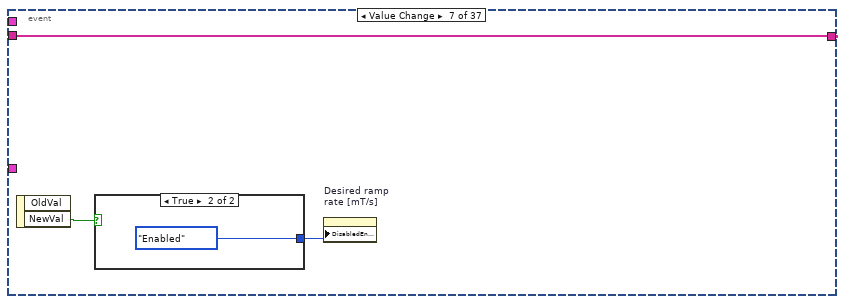
[diagram p15: hidden frame]
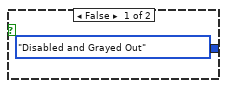
[diagram p16: hidden frame]
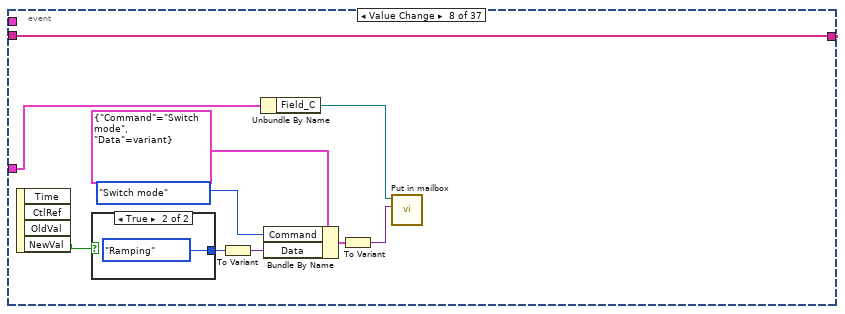
[diagram p17: hidden frame]
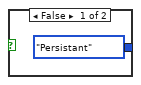
[diagram p18: hidden frame]
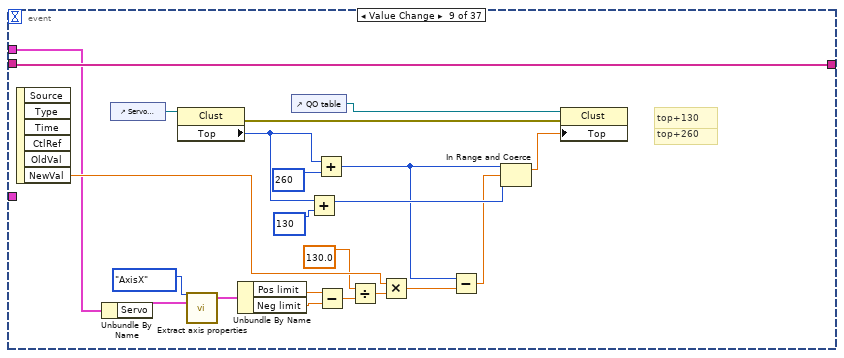
[diagram p19: hidden frame]
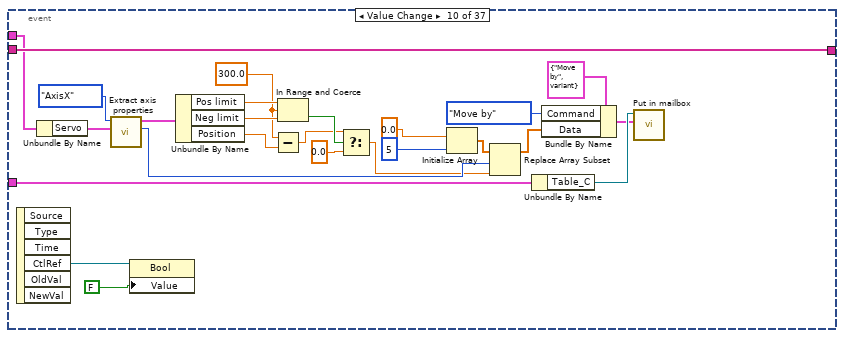
[diagram p20: hidden frame]
diagram:
  w1 = T26 {"Start"=nan, "Start Caption"="Start [T]", "End"=0.0, "End Caption"="End [T]", "Sweep"=0.0, "Sweep caption"="Rate [mT/s]", "Constant"=0.0, "Constant caption"="Freq [GHz]", "Mod_F [kHz]"=0.0, "Mod_A [G]"=0.0, "Tau [ms]"=0.0, "Positioners [mm|°]"=[], "Tmp [K]"=50.0, "Wait [min]"=0.0, "Carousel"=-1, "Comment"="", "Auto-mod"=TRUE, "Execute"=FALSE}  # Script Line
  w4 = T24 {"Remains"=0.0, "T_sample [K]"=1.6, "Last log"="", "Experiment state"=enum."Setup", "Field [T]"=0.0, "Sample holder"=enum."Simple", "Started"=timestamp(0 s since 1904-01-01)}  # Infobar
  n1 = call "Initialize Messenger.vi"() -> ("Referencies out"=w10:T30)  [unwired: 2 in, 1 out]
  n2 = Initialize Array("", 200 ("dimension size")) -> (w7:string[])
  n3 = while {
    tunnel: w10 -> [w25]
    shift-right: [w14] -> _
    shift-left: w7 -> [w24]
    shift-right: [w22] -> w5
    shift-left: TopStates."Initialize GUI" ("State") -> [w23]
    shift-right: [w20] -> _
    shift-left: _ -> [w19]
    shift-right: [w11] -> _
    shift-left: w1 -> [w17]
    shift-right: [w15] -> _
    shift-left: w4 -> [w16]
    shift-right: [w12] -> _
    shift-left: T8 {"Magnet"={"PSU"="None", "T monitor"="None", "Last update"=timestamp(0 s since 1904-01-01), "Field [T]"=0.0, "Ramp [mT/s]"=0.0, "Heater"=FALSE, "Ramp state"=enum."At Target"}, "MFLI"={"Lock-in"="None", "Multimeter"="None", "Last update"=timestamp(0 s since 1904-01-01), "Freq [kHz]"=0.0, "Ampl [mV]"=0.0, "OutEn"=FALSE, "In50 Ohm"=FALSE, "DemEn"=FALSE}, "THz"={"Name"="None", "Description"="None", "Last update"=timestamp(0 s since 1904-01-01), "Start [GHz]"=0.0, "Im Freq[MHz]"=0.0, "End [GHz]"=0.0}, "VTI"={"TempCtl"="", "Last update"=timestamp(0 s since 1904-01-01), "VTI [K]"=0.0, "Sample [K]"=0.0, "Trap[K]"=0.0, "HePot [K]"=0.0, "Ambient [K]"=0.0}, "Rotator"={"Name"=0, "Last update"=timestamp(0 s since 1904-01-01), "Axes"=[]}, "Servo"=[{"Name"=enum."Unknown", "Last update"=timestamp(0 s since 1904-01-01), "Position"=0.0, "Pos limit"=0.0, "Neg limit"=0.0, "Power"=FALSE}], "SMU"={"Name"="", "Last update"=timestamp(0 s since 1904-01-01), "SourFunc"="None", "SourValue"=0.0, "MeasFunc"="", "MeasValue"=0.0, "Output"=FALSE}, "PMD"={"Name"="", "Last update"=timestamp(0 s since 1904-01-01), "Position [°]"=0.0, "Speed"=0.0, "Desired [°]"=0.0, "Moving"=FALSE, "reserved"=0.0}, "PwrMonitor"={"Name"="", "Last update"=timestamp(0 s since 1904-01-01), "Outage?"=FALSE, "Low"=FALSE, "No battery"=FALSE, "Battery [%]"=0, "Charging"=FALSE}} ("Instr info") -> [w13]
    stop <- w21 stop-if-true
    # "State Machine While Loop"
    n4 = case shown="\"Check measurement\"" w23 {
      tunnel: w25 -> [_ w125 w1415 w2930 _ _]
      tunnel: w24 -> [w88 w124 w1429 w2929 w3218 _]
      tunnel: [w87 w113 w1428 w2928 w3217 w3223] -> w14
      tunnel: [TopStates."Wait for Event" ("State") TopStates."Check message" ("State") w1418 TopStates."Wait for Event" ("State") TopStates."Stop" ("State") TopStates."Initialize GUI" ("State")] -> w22
      tunnel: [_ w122 _ _ _ _] -> w21
      tunnel: [w74 w114 w1416 w2925 w3215 w3222] -> w11
      tunnel: w17 -> [w74 w120 w1416 w2926 w3215 w3222]
      tunnel: [w72 w115 w1417 w2927 w3214 w3221] -> w15
      tunnel: w16 -> [w73 w119 w1412 w2922 w3214 w3221]
      tunnel: w13 -> [w64 w116 w1414 w2923 w3213 w3220]
      tunnel: [w64 w116 w1413 w2923 w3213 w3220] -> w12
      frame "Initialize GUI", Default {
        w34 = FALSE  # Hide script
        w42 = T2 {"To disable"=[], "To enable"=[]}  # Controls referencies
        w63 = TRUE ("Visible")
        n5 = local read "Use previous settings"() -> (w57:bool)
        n6 = property on="Actual measurement" class="Clust (strict)"("Visible"=w34) -> ()  [unwired: 2 in, 2 out]
        n7 = case shown="True" w57 {
          tunnel: [w98 w100] -> w60
          tunnel: [T19 {"Filter order"=7.0, "Filter tau [ms]"=50.0, "F_Mod [kHz]"=1.0, "Amp_Mod [mV]"=1.0, "Enable output"=0, "Phase [°]"=0.0} ("ACQ parameters") w103] -> w54
          frame False {
            w98 = T21 {"AMC"=9, "Multip"=1, "Base frequency [GHz]"=90.0, "End frequency [GHz]"=90.0, "Im frequency [MHz]"=10.0, "Sweep up [ms]"=0.0, "Reset trigger?"=FALSE}  # VDI control
          }
          frame True {
            n8 = local read "THz control"() -> (w102:T21)
            n9 = call "Open config file.vi"("MAG config file path"="System config file path") -> ("error out"=w111:errorcluster, "Refnum out"=w112:T76)  [unwired: 7 in, 2 out]
            n10 = property on="ACQ parameters" class="Clust (strict)"() -> ("Value"=w101:T19)  [unwired: 2 in, 2 out]
            n11 = call <userlib>:"Read Section Cluster__ogtk.vi"("error in (no error)"=w111, "Section Formatted Cluster Type"=w101, "refnum"=w112) -> ("Section Formatted Cluster"=w110:variant, "dup refnum"=w107:T76)  [unwired: 4 in, 3 out]
            n12 = Variant To Data(type=w101, Variant=w110) -> (data=w103:T19)  [unwired: 1 in, 1 out]
            n13 = call <userlib>:"Read Section Cluster__ogtk.vi"("Section Formatted Cluster Type"=w102, "refnum"=w107) -> ("error out"=w109:errorcluster, "Section Formatted Cluster"=w108:variant, "dup refnum"=w106:T76)  [unwired: 5 in, 2 out]
            n14 = Variant To Data(error in=w109, type=w102, Variant=w108) -> (data=w100:T21, error out=w104:errorcluster)
            n15 = call <vilib>:"Close Config Data.vi"("error in (no error)"=w104, "refnum"=w106) -> ("file path"=w99:path)  [unwired: 8 in, 1 out]
            n16 = local write "System config file path"(w99) -> ()
          }
        }
        n17 = control-ref of="Acquisition controls"() -> (w76:refnum<vi>)
        n18 = control-ref of="THz control"() -> (w58:refnum<vi>)
        n19 = control-ref of="VTI control"() -> (w59:refnum<vi>)
        n20 = control-ref of="Magnet controls"() -> (w75:refnum<vi>)
        n21 = control-ref of="Run script btn"() -> (w52:refnum<vi>)
        n22 = control-ref of="Servo controls"() -> (w65:refnum<vi>)
        n23 = local read "Acquisition controls"() -> (w56:T18)
        n24 = local write "Select module"(Module_selection."All" ("Module")) -> ()
        n25 = local write "Tab Control"(Application_tabs."Page Status" ("Tab Control")) -> ()
        n26 = Build Array(w76, w58, w59, w65, w75) -> (w66:refnum<vi>[])
        "Instr control refs" <- w66
        n27 = property on="Script Array" class="Arr (strict)"("Visible"=w63) -> ()  [unwired: 2 in, 2 out]
        n28 = property on="Instr control refs" class="Arr (strict)"("Visible"=w63) -> ()  [unwired: 2 in, 2 out]
        n29 = Build Array (concatenate)(w66, w52) -> (w33:refnum<vi>[])
        n30 = Unbundle By Name(w56) -> ("Sample holder"=w30:T20)
        n31 = property class="Clust"(reference=w65) -> ("Top"=w69:i32)  [unwired: 1 in, 2 out]
        n32 = call "Dis- or en- able controls.vi"("Disabled"=T33."Disabled and Grayed Out", "Control referencies"=w33) -> ()  [unwired: 9 in, 1 out]
        n33 = control-ref of="QO table"() -> (w68:refnum<vi>)
        n34 = Add(x=w69, y=260 ("Position:Top")) -> (x+y=w70:i32)
        n35 = Bundle By Name(cluster=w73, "Sample holder"=w30, "Experiment state"=experiment_state."Setup" ("Value")) -> (w72:T24)
        n36 = property class="Clust"(reference=w68, "Top"=w70) -> ()  [unwired: 1 in, 2 out]
        n37 = call <vilib>:"Is Path and Not Empty.vi"("path"="Main data folder") -> ("Is Path and Not Empty?"=w32:bool)  [unwired: 4 in]
        n38 = case shown="False" w32 {
          frame False {
            w94 = T77 2 items=["User Home"=0, "User Desktop"=1, "User Documents"=2, "User Application Data"=3, "User Preferences"=4, "User Temporary"=5, "Public Documents"=6, "Public Application Data"=7, "Public Preferences"=8, "Public Cache"=13, "System Core Libraries"=9, "System Installed Libraries"=10, "Application Files"=11, "Boot Volume Root"=12] ("system directory type")
            n39 = Format Date/Time String(time format string (%c)="%Y") -> (date/time string=w90:string)  [unwired: 2 in]
            n40 = call <vilib>:"Get System Directory.vi"("system directory type"=w94) -> ("system directory"=w96:path)  [unwired: 10 in]
            n41 = Build Path(base path=w96, name or relative path="Measurements") -> (appended path=w95:path)
            n42 = Build Path(base path=w95, name or relative path=w90) -> (appended path=w92:path)
            n43 = local write "Main data folder"(w92) -> ()
          }
          frame True {
          }
        }
        n44 = control-ref of="Save script file btn"() -> (w35:refnum<vi>)
        n45 = local write "THz control"(w60) -> ()
        n46 = property on="ACQ parameters" class="Clust (strict)"("Value"=w54) -> ()  [unwired: 2 in, 2 out]
        n47 = control-ref of="Load script btn"() -> (w36:refnum<vi>)
        n48 = control-ref of="Open measurement"() -> (w37:refnum<vi>)
        n49 = control-ref of="Direct stop meas. btn"() -> (w40:refnum<vi>)
        n50 = Initialize Array("Empty", 10 ("dimension size")) -> (w44:string[])
        n51 = Build Array (concatenate)(w35, w36, w37, w33) -> (w38:refnum<vi>[])
        n52 = property on="Data file to show" class="Ring (strict)"("Strings []"=w44) -> ()  [unwired: 2 in, 2 out]
        n53 = Build Array(w40) -> (w39:refnum<vi>[])
        n54 = call "Create new Log files.vi"("Log folder"="Log folder") -> ("error out"=w82:errorcluster, "dup path"=w53:path, "tmp logfile out"=→"Temperature log ref":refnum<file>, "event logfile out"=w83:refnum<file>)  [unwired: 7 in]
        n55 = Bundle By Name(cluster=w42, "To disable"=w38, "To enable"=w39) -> (→"Controls referencies":T2)
        n56 = Initialize Array(0.0 ("element"), 12 ("dimension size")) -> (w29:dbl[])
        n57 = local write "Log folder"(w53) -> ()
        n58 = call "Add actual date time to string.vi"("String in"="GUI initialized") -> ("String out"=w81:string)  [unwired: 4 in]
        n59 = local write "Drift[K/s]"(w29) -> ()
        n60 = Concatenate Strings(w81, "\r\n") -> (w80:string)
        n61 = call "simple Shift string array.vi"("Element in"=w81, "Array in"=w88) -> ("Array out"=w87:string[])  [unwired: 8 in, 1 out]
        n62 = Write to Text File(file (use dialog)=w83, text=w80, error in=w82) -> (refnum out=→"loggersRef":refnum<file>)  [unwired: 1 in, 2 out]
        n63 = Initialize Array(T31 {"Mode"=enum."MD EPR", "Array"=[]} ("Results"), 10 ("dimension size")) -> (→"Results":T31[])
        n64 = Initialize Array("", 10 ("dimension size")) -> (w50:string[])
        n65 = local write "Header"(w50) -> ()
        "Instr status" <- T1 {"Mag"=FALSE, "Rot"=FALSE, "VTI"=FALSE, "MFLI"=FALSE, "Serv"=FALSE, "THz"=FALSE, "ADQ7"=FALSE, "SMU"=FALSE, "PMD"=FALSE, "UPS"=FALSE, "DMM"=FALSE, "abc"=FALSE} ("Instruments status 2")
        "Infobar" <- T24 {"Remains"=0.0, "T_sample [K]"=0.0, "Last log"="", "Experiment state"=enum."Setup", "Field [T]"=0.0, "Sample holder"=enum."Simple", "Started"=timestamp(0 s since 1904-01-01)} ("Infobar")
      }
      frame "Wait for Event" {
        n66 = event shown="[0] Timeout" {
          selector: _ -> [_ _ _ _ _]
          dyn-events: _ -> [_ _ _ _ _]
          timeout: 5 -> [_ _ _ _ _]
          tunnel: w124 -> [w132 w1143 w1153 w1225 w1309]
          tunnel: [w134 w1143 w1153 w1225 w1308] -> w113
          tunnel: w125 -> [w127 _ w1147 w1227 w1310]
          tunnel: [_ _ _ w1226 _] -> w122
          tunnel: [w131 w1146 w1152 w1224 w1307] -> w114
          tunnel: w120 -> [w130 w1146 w1152 w1224 w1307]
          tunnel: [w129 w1145 w1151 w1223 w1306] -> w117
          tunnel: w119 -> [w128 w1145 w1151 w1223 w1306]
          tunnel: w116 -> [w126 _ _ _ _]
          event Timeout {
            n67 = event-data() -> ()  [unwired: 1 in, 3 out]
            n68 = case shown="\"Script Editor\"" "Tab Control" {
              tunnel: [w138 w145 w845 w979 w1083 w1142] -> w134
              tunnel: w132 -> [w138 w143 w846 w979 w1083 w1142]
              tunnel: w127 -> [_ w142 w843 _ _ _]
              tunnel: [w137 w141 w842 w978 w1082 w1141] -> w131
              tunnel: w130 -> [w137 w141 w841 w978 w1082 w1141]
              tunnel: [w136 w140 w839 w977 w1081 w1140] -> w129
              tunnel: w128 -> [w136 w140 w840 w977 w1081 w1140]
              tunnel: w126 -> [w135 w139 _ _ _ _]
              frame "Page Status" {
                n69 = local write "Instr info"(w135) -> ()
              }
              frame "Adjustment", Default {
                n70 = event shown="[24] \"Piezo controls.Rot set position btn\": Value Change" {
                  selector: _ -> [_ _ _ _ _ _ _ _ _ _ _ _ _ _ _ _ _ _ _ _ _ _ _ _ _ _ _ _ _ _ _ _ _ _ _ _ _]
                  dyn-events: _ -> [_ _ _ _ _ _ _ _ _ _ _ _ _ _ _ _ _ _ _ _ _ _ _ _ _ _ _ _ _ _ _ _ _ _ _ _ _]
                  timeout: 0 -> [_ _ _ _ _ _ _ _ _ _ _ _ _ _ _ _ _ _ _ _ _ _ _ _ _ _ _ _ _ _ _ _ _ _ _ _ _]
                  tunnel: w143 -> [w146 w162 w177 w185 w193 w199 w200 w209 w219 w263 w273 w302 w316 w341 w367 w397 w432 w477 w506 w531 w557 w582 w608 w633 w656 w671 w690 w712 w721 w736 w787 w796 w807 w816 w823 w830 w836]
                  tunnel: [w146 w166 w177 w185 w193 w199 w200 w209 w219 w263 w273 w302 w316 w341 w367 w397 w432 w477 w506 w531 w557 w582 w608 w633 w656 w671 w690 w712 w721 w736 w787 w796 w807 w816 w823 w830 w836] -> w145
                  tunnel: w142 -> [_ w152 w171 w180 w188 w195 _ w205 _ w253 w270 w299 w307 w332 w358 w383 w408 w452 w497 w522 w548 w573 w599 w624 w654 w667 w688 w703 _ w735 w786 w793 w806 w811 w817 w826 _]
                  tunnel: w139 -> [_ _ _ _ _ _ _ _ w218 w240 w265 _ w304 w328 w354 w379 w405 w448 w494 w518 w544 w569 w595 w620 _ _ _ _ _ _ _ _ _ _ _ _ _]
                  event Timeout {
                    (unwired) TopStates."Check message" ("State")
                    n71 = event-data() -> ()  [unwired: 1 in, 3 out]
                  }
                  event Value Change {
                    w147 = 16.0  # MaxB[T]
                    n72 = event-data() -> ()  [unwired: 1 in, 6 out]
                    n73 = local read "Magnet controls"() -> (w168:T23)
                    n74 = Unbundle By Name(w168) -> ("Set Field [T]"=w159:dbl, "Desired ramp\nrate [mT/s]"=w149:dbl, "Custom\nramp"=w155:bool)
                    n75 = Greater?(x=w159, y=w147) -> (0:w160:bool)
                    n76 = Divide(x=w149, y=1000.0) -> (x/y=w150:dbl)
                    n77 = Select(t=w147, s=w160, f=w159) -> (s? t:f=w157:dbl)
                    n78 = Bundle By Name(cluster=T35 {"Field [T]"=0.0, "Ramp [T/s]"=0.0, "Custom Ramp?"=FALSE, "Mode"=enum."Persistant"} ("Set Field"), "Field [T]"=w157, "Ramp [T/s]"=w150, "Custom Ramp?"=w155, "Mode"=Magnet_mode_public."Ramping") -> (w156:T35)
                    n79 = Format Into String(format string="%f T", initial string="Invalid field value" ("Element in"), w159) -> (resulting string=w163:string)  [unwired: 1 in, 1 out]
                    n80 = call "simple Shift string array.vi"("Element in"=w163, "Array in"=w162) -> ("Array out"=w161:string[])  [unwired: 8 in, 1 out]
                    n81 = Bundle By Name(cluster=T37 {"Command"=enum."Set field", "Data"=variant(enum16{"Ramping", "Perzistant"} enum."Ramping")} ("MSG to magnet"), "Command"=Magnet_Orders."Set field" ("Order"), "Data"=w156) -> (w170:T37)
                    n82 = Select(t=w161, s=w160, f=w162) -> (s? t:f=w166:string[])
                    n83 = Unbundle By Name(w152) -> ("Field_C"=w154:refnum<queue>)
                    n84 = To Variant(anything=w170) -> (Variant=w153:variant)
                    n85 = call "Put in mailbox.vi"("Message"=w153, "Queue in"=w154) -> ()  [unwired: 7 in, 3 out]
                  }
                  event Value Change {
                    n86 = event-data() -> ()  [unwired: 1 in, 6 out]
                    n87 = Bundle By Name(cluster=T37 {"Command"=enum."Stop ramping", "Data"=variant(enum16{"Ramping", "Perzistant"} enum."Ramping")} ("MSG to magnet"), "Command"=Magnet_Orders."Stop ramping" ("Order")) -> (w174:T37)
                    n88 = Unbundle By Name(w171) -> ("Field_C"=w175:refnum<queue>)
                    n89 = call "Put in mailbox.vi"("Message"=w174, "Queue in"=w175) -> ()  [unwired: 7 in, 3 out]
                    n90 = property on="Pause ramp" class="Bool (strict)"("Value"=FALSE) -> ()  [unwired: 2 in, 2 out]
                  }
                  event Value Change {
                    n91 = event-data() -> ("CtlRef"=w179:refnum<vi>)  [unwired: 1 in, 5 out]
                    n92 = property class="Bool (strict)"(reference=w179, "Value"=FALSE) -> ()  [unwired: 1 in, 2 out]
                    n93 = Unbundle By Name(w180) -> ("Field_C"=w182:refnum<queue>)
                    n94 = Bundle By Name(cluster=T37 {"Command"=enum."Zero output", "Data"=variant(enum16{"Ramping", "Perzistant"} enum."Ramping")} ("MSG to magnet"), "Command"=Magnet_Orders."Zero output" ("Order")) -> (w181:T37)
                    n95 = call "Put in mailbox.vi"("Message"=w181, "Queue in"=w182) -> ()  [unwired: 7 in, 3 out]
                  }
                  event Value Change {
                    n96 = event-data() -> ("CtlRef"=w186:refnum<vi>)  [unwired: 1 in, 5 out]
                    n97 = Unbundle By Name(w188) -> ("Field_C"=w190:refnum<queue>)
                    n98 = property class="Bool (strict)"(reference=w186, "Value"=FALSE) -> ()  [unwired: 1 in, 2 out]
                    n99 = Bundle By Name(cluster=T37 {"Command"=enum."Equalize output", "Data"=variant(enum16{"Ramping", "Perzistant"} enum."Ramping")} ("MSG to magnet"), "Command"=Magnet_Orders."Equalize output" ("Order")) -> (w189:T37)
                    n100 = call "Put in mailbox.vi"("Message"=w189, "Queue in"=w190) -> ()  [unwired: 7 in, 3 out]
                  }
                  event Value Change {
                    n101 = event-data() -> ("NewVal"=w194:bool)  [unwired: 1 in, 5 out]
                    n102 = Unbundle By Name(w195) -> ("Field_C"=w197:refnum<queue>)
                    n103 = Bundle By Name(cluster=T37 {"Command"=enum."Flip polarity", "Data"=variant(enum16{"Ramping", "Perzistant"} enum."Ramping")} ("MSG to magnet"), "Data"=w194) -> (w196:T37)
                    n104 = call "Put in mailbox.vi"("Message"=w196, "Queue in"=w197) -> ()  [unwired: 7 in, 3 out]
                  }
                  event Value Change {
                    n105 = event-data() -> ("NewVal"=w202:bool)  [unwired: 1 in, 1 out]
                    n106 = case shown="True" w202 {
                      tunnel: [T33."Disabled and Grayed Out" ("Disabled") T33."Enabled" ("Disabled")] -> w201
                      frame False {
                      }
                      frame True {
                      }
                    }
                    n107 = property on="Desired ramp\nrate [mT/s]" class="DigNum (strict)"("DisabledEnum"=w201) -> ()  [unwired: 2 in, 2 out]
                  }
                  event Value Change {
                    n108 = event-data() -> ("NewVal"=w210:bool)  [unwired: 1 in, 3 out]
                    n109 = case shown="True" w210 {
                      tunnel: [Magnet_mode_public."Persistant" ("Operation mode") Magnet_mode_public."Ramping" ("Operation mode")] -> w211
                      frame False {
                      }
                      frame True {
                      }
                    }
                    n110 = To Variant(anything=w211) -> (Variant=w208:variant)
                    n111 = Unbundle By Name(w205) -> ("Field_C"=w207:refnum<queue>)
                    n112 = Bundle By Name(cluster=T37 {"Command"=enum."Switch mode", "Data"=variant(enum16{"Ramping", "Perzistant"} enum."Ramping")} ("MSG to magnet"), "Command"=Magnet_Orders."Switch mode" ("Order"), "Data"=w208) -> (w214:T37)
                    n113 = To Variant(anything=w214) -> (Variant=w206:variant)
                    n114 = call "Put in mailbox.vi"("Message"=w206, "Queue in"=w207) -> ()  [unwired: 7 in, 3 out]
                  }
                  event Value Change {
                    # "top+260"
                    # "top+130"
                    n115 = event-data() -> ("NewVal"=w230:dbl)  [unwired: 1 in, 5 out]
                    n116 = Unbundle By Name(w218) -> ("Servo"=w217:T10[])
                    n117 = control-ref of="Servo controls"() -> (w238:refnum<vi>)
                    n118 = property class="Clust"(reference=w238) -> (error out=w229:errorcluster, "Top"=w224:i32)  [unwired: 1 in, 1 out]
                    n119 = call "Extract axis properties.vi"("Name"=Axis_names."AxisX", "All servo status"=w217) -> ("Servo"=w235:T10)  [unwired: 6 in, 2 out]
                    n120 = Unbundle By Name(w235) -> ("Pos limit"=w233:dbl, "Neg limit"=w232:dbl)
                    n121 = control-ref of="QO table"() -> (w234:refnum<vi>)
                    n122 = Add(x=w224, y=130) -> (x+y=w226:i32)
                    n123 = Add(x=w224, y=260) -> (x+y=w223:i32)
                    n124 = Subtract(x=w233, y=w232) -> (x-y=w220:dbl)
                    n125 = Divide(x=130.0 ("y"), y=w220) -> (x/y=w231:dbl)
                    n126 = Multiply(x=w230, y=w231) -> (x*y=w227:dbl)
                    n127 = Subtract(x=w223, y=w227) -> (x-y=w222:dbl)
                    n128 = In Range and Coerce(upper limit=w223, x=w222, lower limit=w226) -> (coerced(x)=w237:dbl)  [unwired: 1 out]
                    n129 = property class="Clust"(reference=w234, error in=w229, "Top"=w237) -> ()  [unwired: 2 out]
                  }
                  event Value Change {
                    w245 = 300.0 ("x")
                    n130 = event-data() -> ("CtlRef"=w262:refnum<vi>)  [unwired: 1 in, 5 out]
                    n131 = Unbundle By Name(w240) -> ("Servo"=w239:T10[])
                    n132 = call "Extract axis properties.vi"("Name"=Axis_names."AxisX", "All servo status"=w239) -> ("Servo"=w260:T10, "Index"=w251:i32)  [unwired: 6 in, 1 out]
                    n133 = property class="Bool"(reference=w262, "Value"=FALSE) -> ()  [unwired: 1 in, 2 out]
                    n134 = Unbundle By Name(w260) -> ("Pos limit"=w247:dbl, "Neg limit"=w246:dbl, "Position"=w248:dbl)
                    n135 = Subtract(x=w245, y=w248) -> (x-y=w242:dbl)
                    n136 = In Range and Coerce(upper limit=w247, x=w245, lower limit=w246) -> (In Range?=w244:bool)  [unwired: 1 out]
                    n137 = Select(t=w242, s=w244, f=0.0) -> (s? t:f=w241:dbl)
                    n138 = Initialize Array(0.0 ("element"), 5 ("dimension size")) -> (w249:dbl[])
                    n139 = Replace Array Subset(array=w249, new element=w241, index=w251) -> (w250:dbl[])
                    n140 = Unbundle By Name(w253) -> ("Table_C"=w254:refnum<queue>)
                    n141 = Bundle By Name(cluster=T39 {"Command"=enum."Move by", "Data"=variant(dbl[] [])} ("MSG to Servo"), "Command"=Servo_commands."Move by", "Data"=w250) -> (w252:T39)
                    n142 = call "Put in mailbox.vi"("Message"=w252, "Queue in"=w254) -> ()  [unwired: 7 in, 3 out]
                  }
                  event Value Change {
                    n143 = event-data() -> ("CtlRef"=w272:refnum<vi>, "NewVal"=w269:bool)  [unwired: 1 in, 2 out]
                    n144 = Unbundle By Name(w265) -> ("Servo"=w264:T10[])
                    n145 = property class="Bool"(reference=w272, "Value"=FALSE) -> ()  [unwired: 1 in, 2 out]
                    n146 = call "Timeout dialoge Abbort.vi"("Enable"=w269, "Message to Display"="Really go to measurement position?", "timeout[ms]"=u32 3000) -> ("Yes"=w266:bool)  [unwired: 15 in, 1 out]
                    n147 = case shown="True" w266 {
                      tunnel: w270 -> [_ w287]
                      tunnel: w264 -> [_ w275]
                      frame False {
                      }
                      frame True {
                        w274 = 916.0 ("x")
                        # "previous\n890\n895\n899"
                        n148 = call "Extract axis properties.vi"("Name"=Axis_names."AxisX", "All servo status"=w275) -> ("Servo"=w294:T10, "Index"=w285:i32)  [unwired: 6 in, 1 out]
                        n149 = Unbundle By Name(w294) -> ("Pos limit"=w281:dbl, "Neg limit"=w280:dbl, "Position"=w282:dbl)
                        n150 = Subtract(x=w274, y=w282) -> (x-y=w277:dbl)
                        n151 = In Range and Coerce(upper limit=w281, x=w274, lower limit=w280) -> (In Range?=w279:bool)  [unwired: 1 out]
                        n152 = Unbundle By Name(w287) -> ("Table_C"=w288:refnum<queue>)
                        n153 = Select(t=w277, s=w279, f=0.0) -> (s? t:f=w276:dbl)
                        n154 = Initialize Array(0.0 ("element"), 5 ("dimension size")) -> (w283:dbl[])
                        n155 = Replace Array Subset(array=w283, new element=w276, index=w285) -> (w284:dbl[])
                        n156 = Bundle By Name(cluster=T39 {"Command"=enum."Move by", "Data"=variant(dbl[] [])} ("MSG to Servo"), "Command"=Servo_commands."Move by", "Data"=w284) -> (w286:T39)
                        n157 = call "Put in mailbox.vi"("Message"=w286, "Queue in"=w288) -> ()  [unwired: 7 in, 3 out]
                      }
                    }
                  }
                  event Value Change {
                    n158 = event-data() -> ("CtlRef"=w301:refnum<vi>)  [unwired: 1 in, 4 out]
                    n159 = Unbundle By Name(w299) -> ("Table_C"=w296:refnum<queue>)
                    n160 = Bundle By Name(cluster=T39 {"Command"=enum."Stop", "Data"=variant(dbl[] [])} ("MSG to Servo"), "Command"=Servo_commands."Stop") -> (w295:T39)
                    n161 = property class="Bool"(reference=w301, "Value"=FALSE) -> ()  [unwired: 1 in, 2 out]
                    n162 = call "Put in mailbox.vi"("Message"=w295, "Queue in"=w296) -> ()  [unwired: 7 in, 3 out]
                  }
                  event Value Change {
                    # "X position limit"
                    n163 = event-data() -> ("CtlRef"=w305:refnum<vi>)  [unwired: 1 in, 5 out]
                    n164 = Unbundle By Name(w304) -> ("Servo"=w303:T10[])
                    n165 = call "Extract axis properties.vi"("Name"=Axis_names."AxisX", "All servo status"=w303) -> ("Servo"=w313:T10, "Index"=w310:i32)  [unwired: 6 in, 1 out]
                    n166 = property class="Bool"(reference=w305, "Value"=FALSE) -> ()  [unwired: 1 in, 2 out]
                    n167 = Unbundle By Name(w313) -> ("Position"=w308:dbl, "Pos limit"=w311:dbl)
                    n168 = property on="Step\n[mm]" class="DigNum (strict)"() -> ("Value"=w309:dbl)  [unwired: 2 in, 2 out]
                    n169 = Subtract(x=w311, y=w309) -> (x-y=w315:dbl)
                    n170 = Less?(x=w308, y=w315) -> (x < y?=w314:bool)
                    n171 = case shown="True" w314 {
                      tunnel: w309 -> [_ w325]
                      tunnel: w310 -> [_ w321]
                      tunnel: w307 -> [_ w318]
                      frame False {
                      }
                      frame True {
                        n172 = Initialize Array(0.0 ("element"), 5 ("dimension size")) -> (w326:dbl[])
                        n173 = Replace Array Subset(array=w326, new element=w325, index=w321) -> (w322:dbl[])
                        n174 = Bundle By Name(cluster=T39 {"Command"=enum."Move by", "Data"=variant(dbl[] [])} ("MSG to Servo"), "Command"=Servo_commands."Move by", "Data"=w322) -> (w319:T39)
                        n175 = Unbundle By Name(w318) -> ("Table_C"=w320:refnum<queue>)
                        n176 = call "Put in mailbox.vi"("Message"=w319, "Queue in"=w320) -> ()  [unwired: 7 in, 3 out]
                      }
                    }
                  }
                  event Value Change {
                    n177 = event-data() -> ("CtlRef"=w330:refnum<vi>)  [unwired: 1 in, 5 out]
                    n178 = Unbundle By Name(w328) -> ("Servo"=w329:T10[])
                    n179 = property on="Step\n[mm]" class="DigNum (strict)"() -> ("Value"=w334:dbl)  [unwired: 2 in, 2 out]
                    n180 = call "Extract axis properties.vi"("Name"=Axis_names."AxisX", "All servo status"=w329) -> ("Servo"=w338:T10, "Index"=w335:i32)  [unwired: 6 in, 1 out]
                    n181 = property class="Bool"(reference=w330, "Value"=FALSE) -> ()  [unwired: 1 in, 2 out]
                    n182 = Unbundle By Name(w338) -> ("Position"=w333:dbl, "Neg limit"=w336:dbl)
                    n183 = Add(x=w336, y=w334) -> (x+y=w339:dbl)
                    n184 = Greater?(x=w333, y=w339) -> (0:w340:bool)
                    n185 = case shown="True" w340 {
                      tunnel: w334 -> [_ w350]
                      tunnel: w335 -> [_ w346]
                      tunnel: w332 -> [_ w343]
                      frame False {
                      }
                      frame True {
                        n186 = Negate(x=w350) -> (-x=w352:dbl)
                        n187 = Initialize Array(0.0 ("element"), 5 ("dimension size")) -> (w351:dbl[])
                        n188 = Replace Array Subset(array=w351, new element=w352, index=w346) -> (w347:dbl[])
                        n189 = Unbundle By Name(w343) -> ("Table_C"=w344:refnum<queue>)
                        n190 = Bundle By Name(cluster=T39 {"Command"=enum."Move by", "Data"=variant(dbl[] [])} ("MSG to Servo"), "Command"=Servo_commands."Move by", "Data"=w347) -> (w342:T39)
                        n191 = call "Put in mailbox.vi"("Message"=w342, "Queue in"=w344) -> ()  [unwired: 7 in, 3 out]
                      }
                    }
                  }
                  event Value Change {
                    w364 = 0.5 ("y")
                    n192 = event-data() -> ("CtlRef"=w356:refnum<vi>)  [unwired: 1 in, 3 out]
                    n193 = Unbundle By Name(w354) -> ("Servo"=w355:T10[])
                    n194 = call "Extract axis properties.vi"("Name"=Axis_names."AxisY", "All servo status"=w355) -> ("Servo"=w363:T10, "Index"=w360:i32)  [unwired: 6 in, 1 out]
                    n195 = Unbundle By Name(w363) -> ("Position"=w359:dbl, "Pos limit"=w361:dbl)
                    n196 = property class="Bool"(reference=w356, "Value"=FALSE) -> ()  [unwired: 1 in, 2 out]
                    n197 = Subtract(x=w361, y=w364) -> (x-y=w365:dbl)
                    n198 = Less?(x=w359, y=w365) -> (x < y?=w366:bool)
                    n199 = case shown="True" w366 {
                      tunnel: w364 -> [_ w376]
                      tunnel: w360 -> [_ w372]
                      tunnel: w358 -> [_ w368]
                      frame False {
                      }
                      frame True {
                        n200 = Initialize Array(0.0 ("element"), 5 ("dimension size")) -> (w377:dbl[])
                        n201 = Replace Array Subset(array=w377, new element=w376, index=w372) -> (w373:dbl[])
                        n202 = Bundle By Name(cluster=T39 {"Command"=enum."Move by", "Data"=variant(dbl[] [])} ("MSG to Servo"), "Command"=Servo_commands."Move by", "Data"=w373) -> (w369:T39)
                        n203 = Unbundle By Name(w368) -> ("Table_C"=w370:refnum<queue>)
                        n204 = call "Put in mailbox.vi"("Message"=w369, "Queue in"=w370) -> ()  [unwired: 7 in, 3 out]
                      }
                    }
                  }
                  event Value Change {
                    w390 = 0.5 ("y")
                    n205 = event-data() -> ("CtlRef"=w381:refnum<vi>)  [unwired: 1 in, 5 out]
                    n206 = Unbundle By Name(w379) -> ("Servo"=w380:T10[])
                    n207 = call "Extract axis properties.vi"("Name"=Axis_names."AxisY", "All servo status"=w380) -> ("Servo"=w388:T10, "Index"=w385:i32)  [unwired: 6 in, 1 out]
                    n208 = Unbundle By Name(w388) -> ("Position"=w384:dbl, "Neg limit"=w387:dbl)
                    n209 = property class="Bool"(reference=w381, "Value"=FALSE) -> ()  [unwired: 1 in, 2 out]
                    n210 = Add(x=w387, y=w390) -> (x+y=w389:dbl)
                    n211 = Negate(x=w390) -> (-x=w391:dbl)
                    n212 = Greater?(x=w384, y=w389) -> (0:w396:bool)
                    n213 = Initialize Array(0.0 ("element"), 5 ("dimension size")) -> (w395:dbl[])
                    n214 = Replace Array Subset(array=w395, new element=w391, index=w385) -> (w392:dbl[])
                    n215 = case shown="True" w396 {
                      tunnel: w392 -> [_ w402]
                      tunnel: w383 -> [_ w399]
                      frame False {
                      }
                      frame True {
                        n216 = Unbundle By Name(w399) -> ("Table_C"=w400:refnum<queue>)
                        n217 = Bundle By Name(cluster=T39 {"Command"=enum."Move by", "Data"=variant(dbl[] [])} ("MSG to Servo"), "Command"=Servo_commands."Move by", "Data"=w402) -> (w398:T39)
                        n218 = call "Put in mailbox.vi"("Message"=w398, "Queue in"=w400) -> ()  [unwired: 7 in, 3 out]
                      }
                    }
                  }
                  event Value Change {
                    w427 = 0.5 ("y")
                    n219 = event-data() -> ("CtlRef"=w406:refnum<vi>)  [unwired: 1 in, 5 out]
                    n220 = Unbundle By Name(w405) -> ("Servo"=w404:T10[])
                    n221 = call "Extract axis properties.vi"("Name"=Axis_names."AxisZ_right", "All servo status"=w404) -> ("Servo"=w425:T10, "Index"=w416:i32)  [unwired: 6 in, 1 out]
                    n222 = call "Extract axis properties.vi"("Name"=Axis_names."AxisZ_middle", "All servo status"=w404) -> ("Servo"=w424:T10, "Index"=w415:i32)  [unwired: 6 in, 1 out]
                    n223 = call "Extract axis properties.vi"("Name"=Axis_names."AxisZ_left", "All servo status"=w404) -> ("Servo"=w426:T10, "Index"=w417:i32)  [unwired: 6 in, 1 out]
                    n224 = property class="Bool"(reference=w406, "Value"=FALSE) -> ()  [unwired: 1 in, 2 out]
                    n225 = Unbundle By Name(w425) -> ("Position"=w411:dbl, "Pos limit"=w419:dbl)
                    n226 = Unbundle By Name(w424) -> ("Position"=w410:dbl, "Pos limit"=w418:dbl)
                    n227 = Unbundle By Name(w426) -> ("Position"=w409:dbl, "Pos limit"=w420:dbl)
                    n228 = Subtract(x=w419, y=w427) -> (x-y=w430:dbl)
                    n229 = Subtract(x=w420, y=w427) -> (x-y=w431:dbl)
                    n230 = Subtract(x=w418, y=w427) -> (x-y=w429:dbl)
                    n231 = Less?(x=w409, y=w431) -> (x < y?=w412:bool)
                    n232 = Less?(x=w411, y=w430) -> (x < y?=w413:bool)
                    n233 = Less?(x=w410, y=w429) -> (x < y?=w414:bool)
                    n234 = Compound Arithmetic op=AND(w413, w414, w412) -> (w428:bool)
                    n235 = case shown="True" w428 {
                      tunnel: w427 -> [_ w439]
                      tunnel: w417 -> [_ w440]
                      tunnel: w416 -> [_ w438]
                      tunnel: w415 -> [_ w437]
                      tunnel: w408 -> [_ w434]
                      frame False {
                      }
                      frame True {
                        n236 = Initialize Array(0.0 ("element"), 5 ("dimension size")) -> (w446:dbl[])
                        n237 = Replace Array Subset(array=w446, new element=w439, index=w438) -> (w443:dbl[])
                        n238 = Replace Array Subset(array=w443, new element=w439, index=w437) -> (w442:dbl[])
                        n239 = Replace Array Subset(array=w442, new element=w439, index=w440) -> (w441:dbl[])
                        n240 = Bundle By Name(cluster=T39 {"Command"=enum."Move by", "Data"=variant(dbl[] [])} ("MSG to Servo"), "Command"=Servo_commands."Move by", "Data"=w441) -> (w435:T39)
                        n241 = Unbundle By Name(w434) -> ("Table_C"=w436:refnum<queue>)
                        n242 = call "Put in mailbox.vi"("Message"=w435, "Queue in"=w436) -> ()  [unwired: 7 in, 3 out]
                      }
                    }
                  }
                  event Value Change {
                    w469 = 0.5 ("y")
                    n243 = event-data() -> ("CtlRef"=w450:refnum<vi>)  [unwired: 1 in, 2 out]
                    n244 = Unbundle By Name(w448) -> ("Servo"=w449:T10[])
                    n245 = property class="Bool"(reference=w450, "Value"=FALSE) -> ()  [unwired: 1 in, 2 out]
                    n246 = call "Extract axis properties.vi"("Name"=Axis_names."AxisZ_middle", "All servo status"=w449) -> ("Servo"=w465:T10, "Index"=w458:i32)  [unwired: 6 in, 1 out]
                    n247 = call "Extract axis properties.vi"("Name"=Axis_names."AxisZ_left", "All servo status"=w449) -> ("Servo"=w468:T10, "Index"=w457:i32)  [unwired: 6 in, 1 out]
                    n248 = call "Extract axis properties.vi"("Name"=Axis_names."AxisZ_right", "All servo status"=w449) -> ("Servo"=w466:T10, "Index"=w456:i32)  [unwired: 6 in, 1 out]
                    n249 = Unbundle By Name(w468) -> ("Position"=w455:dbl, "Neg limit"=w462:dbl)
                    n250 = Unbundle By Name(w465) -> ("Position"=w453:dbl, "Neg limit"=w460:dbl)
                    n251 = Unbundle By Name(w466) -> ("Position"=w454:dbl, "Neg limit"=w461:dbl)
                    n252 = Add(x=w462, y=w469) -> (x+y=w476:dbl)
                    n253 = Add(x=w461, y=w469) -> (x+y=w475:dbl)
                    n254 = Add(x=w460, y=w469) -> (x+y=w474:dbl)
                    n255 = Greater?(x=w455, y=w476) -> (0:w473:bool)
                    n256 = Greater?(x=w454, y=w475) -> (0:w472:bool)
                    n257 = Greater?(x=w453, y=w474) -> (0:w470:bool)
                    n258 = Negate(x=w469) -> (-x=w459:dbl)
                    n259 = Compound Arithmetic op=AND(w473, w472, w470) -> (w471:bool)
                    n260 = case shown="True" w471 {
                      tunnel: w459 -> [_ w485]
                      tunnel: w458 -> [_ w484]
                      tunnel: w457 -> [_ w483]
                      tunnel: w456 -> [_ w482]
                      tunnel: w452 -> [_ w478]
                      frame False {
                      }
                      frame True {
                        n261 = Initialize Array(0.0 ("element"), 5 ("dimension size")) -> (w491:dbl[])
                        n262 = Replace Array Subset(array=w491, new element=w485, index=w484) -> (w488:dbl[])
                        n263 = Replace Array Subset(array=w488, new element=w485, index=w483) -> (w487:dbl[])
                        n264 = Replace Array Subset(array=w487, new element=w485, index=w482) -> (w486:dbl[])
                        n265 = Bundle By Name(cluster=T39 {"Command"=enum."Move by", "Data"=variant(dbl[] [])} ("MSG to Servo"), "Command"=Servo_commands."Move by", "Data"=w486) -> (w479:T39)
                        n266 = Unbundle By Name(w478) -> ("Table_C"=w480:refnum<queue>)
                        n267 = call "Put in mailbox.vi"("Message"=w479, "Queue in"=w480) -> ()  [unwired: 7 in, 3 out]
                      }
                    }
                  }
                  event Value Change {
                    w503 = 0.5 ("y")
                    n268 = event-data() -> ("CtlRef"=w495:refnum<vi>)  [unwired: 1 in, 2 out]
                    n269 = Unbundle By Name(w494) -> ("Servo"=w493:T10[])
                    n270 = call "Extract axis properties.vi"("Name"=Axis_names."AxisZ_left", "All servo status"=w493) -> ("Servo"=w502:T10, "Index"=w499:i32)  [unwired: 6 in, 1 out]
                    n271 = Unbundle By Name(w502) -> ("Position"=w498:dbl, "Pos limit"=w500:dbl)
                    n272 = property class="Bool"(reference=w495, "Value"=FALSE) -> ()  [unwired: 1 in, 2 out]
                    n273 = Subtract(x=w500, y=w503) -> (x-y=w504:dbl)
                    n274 = Less?(x=w498, y=w504) -> (x < y?=w505:bool)
                    n275 = case shown="True" w505 {
                      tunnel: w503 -> [_ w516]
                      tunnel: w499 -> [_ w511]
                      tunnel: w497 -> [_ w507]
                      frame False {
                      }
                      frame True {
                        n276 = Initialize Array(0.0 ("element"), 5 ("dimension size")) -> (w515:dbl[])
                        n277 = Replace Array Subset(array=w515, new element=w516, index=w511) -> (w512:dbl[])
                        n278 = Bundle By Name(cluster=T39 {"Command"=enum."Move by", "Data"=variant(dbl[] [])} ("MSG to Servo"), "Command"=Servo_commands."Move by", "Data"=w512) -> (w508:T39)
                        n279 = Unbundle By Name(w507) -> ("Table_C"=w509:refnum<queue>)
                        n280 = call "Put in mailbox.vi"("Message"=w508, "Queue in"=w509) -> ()  [unwired: 7 in, 3 out]
                      }
                    }
                  }
                  event Value Change {
                    w528 = 0.5 ("y")
                    n281 = event-data() -> ("CtlRef"=w520:refnum<vi>)  [unwired: 1 in, 3 out]
                    n282 = Unbundle By Name(w518) -> ("Servo"=w519:T10[])
                    n283 = call "Extract axis properties.vi"("Name"=Axis_names."AxisZ_left", "All servo status"=w519) -> ("Servo"=w527:T10, "Index"=w524:i32)  [unwired: 6 in, 1 out]
                    n284 = Unbundle By Name(w527) -> ("Position"=w523:dbl, "Neg limit"=w525:dbl)
                    n285 = property class="Bool"(reference=w520, "Value"=FALSE) -> ()  [unwired: 1 in, 2 out]
                    n286 = Add(x=w525, y=w528) -> (x+y=w529:dbl)
                    n287 = Greater?(x=w523, y=w529) -> (0:w530:bool)
                    n288 = case shown="True" w530 {
                      tunnel: w528 -> [_ w540]
                      tunnel: w524 -> [_ w536]
                      tunnel: w522 -> [_ w533]
                      frame False {
                      }
                      frame True {
                        n289 = Negate(x=w540) -> (-x=w542:dbl)
                        n290 = Initialize Array(0.0 ("element"), 5 ("dimension size")) -> (w541:dbl[])
                        n291 = Replace Array Subset(array=w541, new element=w542, index=w536) -> (w537:dbl[])
                        n292 = Unbundle By Name(w533) -> ("Table_C"=w534:refnum<queue>)
                        n293 = Bundle By Name(cluster=T39 {"Command"=enum."Move by", "Data"=variant(dbl[] [])} ("MSG to Servo"), "Command"=Servo_commands."Move by", "Data"=w537) -> (w532:T39)
                        n294 = call "Put in mailbox.vi"("Message"=w532, "Queue in"=w534) -> ()  [unwired: 7 in, 3 out]
                      }
                    }
                  }
                  event Value Change {
                    w554 = 0.5 ("y")
                    n295 = event-data() -> ("CtlRef"=w546:refnum<vi>)  [unwired: 1 in, 3 out]
                    n296 = Unbundle By Name(w544) -> ("Servo"=w545:T10[])
                    n297 = call "Extract axis properties.vi"("Name"=Axis_names."AxisZ_right", "All servo status"=w545) -> ("Servo"=w553:T10, "Index"=w550:i32)  [unwired: 6 in, 1 out]
                    n298 = Unbundle By Name(w553) -> ("Position"=w549:dbl, "Pos limit"=w551:dbl)
                    n299 = property class="Bool"(reference=w546, "Value"=FALSE) -> ()  [unwired: 1 in, 2 out]
                    n300 = Subtract(x=w551, y=w554) -> (x-y=w556:dbl)
                    n301 = Less?(x=w549, y=w556) -> (x < y?=w555:bool)
                    n302 = case shown="True" w555 {
                      tunnel: w554 -> [_ w566]
                      tunnel: w550 -> [_ w562]
                      tunnel: w548 -> [_ w558]
                      frame False {
                      }
                      frame True {
                        n303 = Initialize Array(0.0 ("element"), 5 ("dimension size")) -> (w567:dbl[])
                        n304 = Replace Array Subset(array=w567, new element=w566, index=w562) -> (w563:dbl[])
                        n305 = Bundle By Name(cluster=T39 {"Command"=enum."Move by", "Data"=variant(dbl[] [])} ("MSG to Servo"), "Command"=Servo_commands."Move by", "Data"=w563) -> (w559:T39)
                        n306 = Unbundle By Name(w558) -> ("Table_C"=w560:refnum<queue>)
                        n307 = call "Put in mailbox.vi"("Message"=w559, "Queue in"=w560) -> ()  [unwired: 7 in, 3 out]
                      }
                    }
                  }
                  event Value Change {
                    w578 = 0.5 ("y")
                    n308 = event-data() -> ("CtlRef"=w571:refnum<vi>)  [unwired: 1 in, 4 out]
                    n309 = Unbundle By Name(w569) -> ("Servo"=w570:T10[])
                    n310 = call "Extract axis properties.vi"("Name"=Axis_names."AxisZ_right", "All servo status"=w570) -> ("Servo"=w577:T10, "Index"=w575:i32)  [unwired: 6 in, 1 out]
                    n311 = property class="Bool"(reference=w571, "Value"=FALSE) -> ()  [unwired: 1 in, 2 out]
                    n312 = Unbundle By Name(w577) -> ("Position"=w574:dbl, "Neg limit"=w580:dbl)
                    n313 = Add(x=w580, y=w578) -> (x+y=w579:dbl)
                    n314 = Greater?(x=w574, y=w579) -> (0:w581:bool)
                    n315 = case shown="True" w581 {
                      tunnel: w578 -> [_ w591]
                      tunnel: w575 -> [_ w587]
                      tunnel: w573 -> [_ w583]
                      frame False {
                      }
                      frame True {
                        n316 = Negate(x=w591) -> (-x=w593:dbl)
                        n317 = Initialize Array(0.0 ("element"), 5 ("dimension size")) -> (w592:dbl[])
                        n318 = Replace Array Subset(array=w592, new element=w593, index=w587) -> (w588:dbl[])
                        n319 = Unbundle By Name(w583) -> ("Table_C"=w585:refnum<queue>)
                        n320 = Bundle By Name(cluster=T39 {"Command"=enum."Move by", "Data"=variant(dbl[] [])} ("MSG to Servo"), "Command"=Servo_commands."Move by", "Data"=w588) -> (w584:T39)
                        n321 = call "Put in mailbox.vi"("Message"=w584, "Queue in"=w585) -> ()  [unwired: 7 in, 3 out]
                      }
                    }
                  }
                  event Value Change {
                    w605 = 0.5 ("y")
                    n322 = event-data() -> ("CtlRef"=w597:refnum<vi>)  [unwired: 1 in, 3 out]
                    n323 = Unbundle By Name(w595) -> ("Servo"=w596:T10[])
                    n324 = call "Extract axis properties.vi"("Name"=Axis_names."AxisZ_middle", "All servo status"=w596) -> ("Servo"=w604:T10, "Index"=w601:i32)  [unwired: 6 in, 1 out]
                    n325 = Unbundle By Name(w604) -> ("Position"=w600:dbl, "Pos limit"=w602:dbl)
                    n326 = property class="Bool"(reference=w597, "Value"=FALSE) -> ()  [unwired: 1 in, 2 out]
                    n327 = Subtract(x=w602, y=w605) -> (x-y=w606:dbl)
                    n328 = Less?(x=w600, y=w606) -> (x < y?=w607:bool)
                    n329 = case shown="True" w607 {
                      tunnel: w605 -> [_ w617]
                      tunnel: w601 -> [_ w613]
                      tunnel: w599 -> [_ w609]
                      frame False {
                      }
                      frame True {
                        n330 = Initialize Array(0.0 ("element"), 5 ("dimension size")) -> (w618:dbl[])
                        n331 = Replace Array Subset(array=w618, new element=w617, index=w613) -> (w614:dbl[])
                        n332 = Bundle By Name(cluster=T39 {"Command"=enum."Move by", "Data"=variant(dbl[] [])} ("MSG to Servo"), "Command"=Servo_commands."Move by", "Data"=w614) -> (w610:T39)
                        n333 = Unbundle By Name(w609) -> ("Table_C"=w611:refnum<queue>)
                        n334 = call "Put in mailbox.vi"("Message"=w610, "Queue in"=w611) -> ()  [unwired: 7 in, 3 out]
                      }
                    }
                  }
                  event Value Change {
                    w630 = 0.5 ("y")
                    n335 = event-data() -> ("CtlRef"=w622:refnum<vi>)  [unwired: 1 in, 3 out]
                    n336 = Unbundle By Name(w620) -> ("Servo"=w621:T10[])
                    n337 = call "Extract axis properties.vi"("Name"=Axis_names."AxisZ_middle", "All servo status"=w621) -> ("Servo"=w628:T10, "Index"=w626:i32)  [unwired: 6 in, 1 out]
                    n338 = Unbundle By Name(w628) -> ("Position"=w625:dbl, "Neg limit"=w627:dbl)
                    n339 = property class="Bool"(reference=w622, "Value"=FALSE) -> ()  [unwired: 1 in, 2 out]
                    n340 = Add(x=w627, y=w630) -> (x+y=w631:dbl)
                    n341 = Greater?(x=w625, y=w631) -> (0:w632:bool)
                    n342 = case shown="True" w632 {
                      tunnel: w630 -> [_ w642]
                      tunnel: w626 -> [_ w638]
                      tunnel: w624 -> [_ w635]
                      frame False {
                      }
                      frame True {
                        n343 = Negate(x=w642) -> (-x=w644:dbl)
                        n344 = Initialize Array(0.0 ("element"), 5 ("dimension size")) -> (w643:dbl[])
                        n345 = Replace Array Subset(array=w643, new element=w644, index=w638) -> (w639:dbl[])
                        n346 = Unbundle By Name(w635) -> ("Table_C"=w636:refnum<queue>)
                        n347 = Bundle By Name(cluster=T39 {"Command"=enum."Move by", "Data"=variant(dbl[] [])} ("MSG to Servo"), "Command"=Servo_commands."Move by", "Data"=w639) -> (w634:T39)
                        n348 = call "Put in mailbox.vi"("Message"=w634, "Queue in"=w636) -> ()  [unwired: 7 in, 3 out]
                      }
                    }
                  }
                  event Value Change {
                    n349 = event-data() -> ("CtlRef"=w648:refnum<vi>)  [unwired: 1 in, 5 out]
                    n350 = local read "Piezo controls"() -> (w655:T15)
                    n351 = Unbundle By Name(w654) -> ("Angle_C"=w653:refnum<queue>)
                    n352 = property class="Bool (strict)"(reference=w648, "Value"=FALSE) -> ()  [unwired: 1 in, 2 out]
                    n353 = Unbundle By Name(w655) -> ("Axes properties"=w646:T16[], "Safe to \nmove?"=w647:bool)
                    n354 = for {
                      tunnel: [w661] -> w650 mode=indexing
                      tunnel: w647 -> [w659]
                      tunnel: w646 -> [w658] mode=indexing
                      n355 = Unbundle By Name(w658) -> ("Target [mm|°]"=w657:dbl)
                      n356 = Bundle By Name(cluster=T42 {"Relative?"=FALSE, "Position [°]"=0.0, "Safe to move?"=FALSE} ("output cluster"), "Position [°]"=w657, "Safe to move?"=w659) -> (w661:T42)
                    }
                    n357 = Bundle By Name(cluster=T40 {"Command"=enum."Set position", "Data"=variant} ("MSG to rotator"), "Data"=w650) -> (w651:T40)
                    n358 = call "Put in mailbox.vi"("Message"=w651, "Queue in"=w653) -> ()  [unwired: 7 in, 3 out]
                  }
                  event Value Change {
                    n359 = event-data() -> ("CtlRef"=w662:refnum<vi>)  [unwired: 1 in, 5 out]
                    n360 = Unbundle By Name(w667) -> ("Angle_C"=w666:refnum<queue>)
                    n361 = Unbundle By Name("Piezo controls") -> ("Axes properties"=w665:T16[])
                    n362 = for {
                      tunnel: w665 -> [w673] mode=indexing
                      tunnel: [w675] -> w664
                      i -> [w672]
                      n363 = Unbundle By Name(w673) -> ("DC voltage [V]"=w674:dbl)
                      n364 = Greater Than 0?(x=w674) -> (x > 0?=w679:bool)
                      n365 = case shown="True" w679 {
                        tunnel: [_ w684] -> w678
                        tunnel: w672 -> [_ w681]
                        frame False {
                        }
                        frame True {
                          n366 = Format Into String(format string="DC Voltage at axis %d is not zero.\nDo you realy want to set it?" ("message"), w681) -> (resulting string=w680:string)  [unwired: 2 in, 1 out]
                          n367 = Two Button Dialog(message=w680, 1:"Set to zero" ("F button name (\"Cancel\")")) -> (T button?=w684:bool)  [unwired: 1 in]
                        }
                      }
                      n368 = Select(t=w674, s=w678, f=0.0) -> (s? t:f=w676:dbl)
                      n369 = Bundle By Name(cluster=w673, "DC voltage [V]"=w676) -> (w675:T16)
                    }
                    n370 = property class="Bool (strict)"(reference=w662, "Value"=FALSE) -> ()  [unwired: 1 in, 2 out]
                    n371 = Bundle By Name(cluster=T40 {"Command"=enum."Set parameters", "Data"=variant} ("MSG to rotator"), "Data"=w664) -> (w668:T40)
                    n372 = call "Put in mailbox.vi"("Message"=w668, "Queue in"=w666) -> ()  [unwired: 7 in, 3 out]
                  }
                  event Value Change {
                    n373 = event-data() -> ("CtlRef"=w685:refnum<vi>)  [unwired: 1 in, 5 out]
                    n374 = Unbundle By Name(w688) -> ("Angle_C"=w687:refnum<queue>)
                    n375 = property class="Bool (strict)"(reference=w685, "Value"=FALSE) -> ()  [unwired: 1 in, 2 out]
                    n376 = call "Put in mailbox.vi"("Message"=T40 {"Command"=enum."Stop movement", "Data"=variant} ("MSG to rotator"), "Queue in"=w687) -> ()  [unwired: 7 in, 3 out]
                  }
                  event Value Change {
                    n377 = event-data() -> ()  [unwired: 1 in, 6 out]
                    n378 = Unbundle By Name("THz control") -> ("AMC"=w701:u16, "Multip"=w700:u16, "Base frequency [GHz]"=w708:dbl, "End frequency [GHz]"=w709:dbl, "Im frequency [MHz]"=w710:dbl, "Sweep up [ms]"=w694:dbl, "Reset trigger?"=w693:bool)
                    n379 = Unbundle By Name(w703) -> ("MW_C"=w702:refnum<queue>)
                    n380 = Multiply(x=w701, y=w700) -> (x*y=w696:u16)
                    n381 = Divide(x=w708, y=w696) -> (x/y=w699:dbl)
                    n382 = Divide(x=w709, y=w696) -> (x/y=w698:dbl)
                    n383 = Divide(x=w694, y=2.0) -> (x/y=w692:dbl)
                    n384 = Divide(x=w710, y=w696) -> (x/y=w697:dbl)
                    n385 = Bundle By Name(cluster=T44 {"Start [GHz]"=8.0, "End [GHz] "=8.0, "Sweep up\ntime [ms]"=0.0, "Sweep down\ntime [ms]"=0.0, "Intermidiate [MHz]"=0.0, "Reset trigger"=FALSE} ("Sweep parameters"), "Start [GHz]"=w699, "End [GHz]"=w698, "Intermidiate [MHz]"=w697, "Sweep up\ntime [ms]"=w694, "Sweep down\ntime [ms]"=w692, "Reset trigger"=w693) -> (w705:T44)
                    n386 = Bundle By Name(cluster=T45 {"Command"=enum."Set parameters", "Data"=variant} ("Incoming msg"), "Command"=THz_commands_enum."Set parameters", "Data"=w705) -> (w706:T45)
                    n387 = call "Put in mailbox.vi"("Message"=w706, "Queue in"=w702) -> ()  [unwired: 7 in, 3 out]
                  }
                  event Value Change {
                    n388 = event-data() -> ()  [unwired: 1 in, 6 out]
                    n389 = local read "THz control"() -> (w720:T21)
                    n390 = Unbundle By Name(w720) -> ("AMC"=w717:u16, "Multip"=w716:u16)
                    n391 = Multiply(x=w717, y=w716) -> (x*y=w715:u16)
                    n392 = Multiply(x=14.0, y=w715) -> (x*y=w714:dbl)
                    n393 = Multiply(x=0.01, y=w715) -> (x*y=w713:dbl)
                    n394 = property on="End frequency [GHz]" class="DigNum (strict)"("Minimum"=w713, "Maximum"=w714) -> ()  [unwired: 2 in, 2 out]
                    n395 = property on="Base frequency [GHz]" class="DigNum (strict)"("Minimum"=w713, "Maximum"=w714) -> ()  [unwired: 2 in, 2 out]
                  }
                  event Value Change {
                    n396 = event-data() -> ("CtlRef"=w728:refnum<vi>, "NewVal"=w725:dbl)  [unwired: 1 in]
                    n397 = Unbundle By Name(w735) -> ("Data_Aq"=w734:refnum<queue>)
                    n398 = property class="DigNum (strict)"(reference=w728) -> ("Label.Text"=w727:string)  [unwired: 1 in, 2 out]
                    n399 = case shown="\"Phase [°]\"" w727 {
                      tunnel: [MFLI_node."None" ("parameter") MFLI_node."filter_constant [ms]" ("parameter") MFLI_node."filter_order [-]" ("parameter") MFLI_node."osc_freq [kHz]" ("parameter") MFLI_node."Phase_deg" ("parameter") MFLI_node."out_ampl [V]" ("parameter")] -> w723
                      tunnel: w725 -> [_ w739 w741 w743 w745 w749]
                      tunnel: [_ w739 w741 w743 w745 w761] -> w726
                      tunnel: "Acquisition controls" -> [_ _ _ _ _ w759]
                      tunnel: [_ _ _ _ _ w747] -> _
                      frame "Unknown", Default {
                      }
                      frame "Time constant [ms]" {
                      }
                      frame "Filter order" {
                      }
                      frame "F_Mod [kHz]" {
                      }
                      frame "Phase [°]" {
                      }
                      frame "Amp_Mod [mV]" {
                        n400 = Unbundle By Name(w759) -> ("ACQ parameters.F_Mod [kHz]"=w756:dbl, "Sample holder"=w746:T20)
                        n401 = case shown="\"Carousel\"" w746 {
                          tunnel: [w765 w768 w771 w774] -> w758
                          tunnel: [w764 w767 w770 w773] -> w754
                          tunnel: [w763 w766 w769 w772] -> w748
                          frame "Simple", Default {
                            w763 = 0.0  # G/A
                            w764 = 8.9  # R
                            w765 = 0.0017  # L
                          }
                          frame "Carousel" {
                            w766 = 0.0  # G/A
                            w767 = 8.9  # R
                            w768 = 0.0017  # L
                          }
                          frame "Chip" {
                            w769 = 0.0  # G/A
                            w770 = 8.9  # R
                            w771 = 0.0017  # L
                          }
                          frame "Rotator" {
                            w772 = 0.0  # G/A
                            w773 = 8.9  # R
                            w774 = 0.0017  # L
                          }
                        }
                        n402 = Divide(x=w749, y=1000.0) -> (x/y=w761:dbl)
                        n403 = Square(x=w754) -> (x^2=w752:dbl)
                        n404 = Compound Arithmetic op=MULTIPLY(w756, 6.283185307179586, w758) -> (w755:dbl)
                        n405 = Square(x=w755) -> (x^2=w753:dbl)
                        n406 = Add(x=w753, y=w752) -> (x+y=w751:dbl)
                        n407 = Square Root(x=w751) -> (sqrt(x)=w750:dbl)
                        n408 = Compound Arithmetic op=MULTIPLY(w748, w750) -> (w747:dbl)
                      }
                    }
                    n409 = Bundle(cluster=T46 {"parameter"=enum."filter_order [-]", "value"=0.0} ("Parameter to set"), "parameter"=w723, "value"=w726) -> (w729:T46)
                    n410 = Build Array(w729) -> (w724:T46[])
                    n411 = Bundle By Name(cluster=T49 {"Command"=enum."Initialize", "Data"=variant} ("MSG for  ACQ"), "Command"=MFLI_command_enum."Set individual parameters", "Data"=w724) -> (w731:T49)
                    n412 = call "Put in mailbox.vi"("Message"=w731, "Queue in"=w734) -> ()  [unwired: 7 in, 3 out]
                  }
                  event Value Change {
                    w778 = T46 {"parameter"=enum."filter_order [-]", "value"=0.0} ("Parameter to set")
                    n413 = event-data() -> ("NewVal"=w776:u16)  [unwired: 1 in, 2 out]
                    n414 = Unbundle By Name(w786) -> ("Data_Aq"=w785:refnum<queue>)
                    n415 = Bundle(cluster=w778, "parameter"=MFLI_node."enable output", "value"=w776) -> (w781:T46)
                    n416 = Bundle(cluster=w778, "parameter"=MFLI_node."enamble ampl", "value"=w776) -> (w775:T46)
                    n417 = Build Array(w781, w775) -> (w780:T46[])
                    n418 = Bundle By Name(cluster=T49 {"Command"=enum."Initialize", "Data"=variant} ("MSG for  ACQ"), "Command"=MFLI_command_enum."Set individual parameters", "Data"=w780) -> (w782:T49)
                    n419 = call "Put in mailbox.vi"("Message"=w782, "Queue in"=w785) -> ()  [unwired: 7 in, 3 out]
                  }
                  event Value Change {
                    n420 = event-data() -> ("CtlRef"=w795:refnum<vi>)  [unwired: 1 in, 3 out]
                    n421 = Unbundle By Name(w793) -> ("Data_Aq"=w792:refnum<queue>)
                    n422 = property class="Bool (strict)"(reference=w795, "Value"=FALSE) -> ()  [unwired: 1 in, 2 out]
                    n423 = Build Array(T46 {"parameter"=enum."in_autorange", "value"=1.0} ("Parameter to set")) -> (w789:T46[])
                    n424 = Bundle By Name(cluster=T49 {"Command"=enum."Set individual parameters", "Data"=variant} ("MSG for  ACQ"), "Data"=w789) -> (w788:T49)
                    n425 = call "Put in mailbox.vi"("Message"=w788, "Queue in"=w792) -> ()  [unwired: 7 in, 3 out]
                  }
                  event Value Change {
                    n426 = event-data() -> ("CtlRef"=w802:refnum<vi>, "NewVal"=w800:dbl)  [unwired: 1 in]
                    n427 = property class="DigNum (strict)"(reference=w802) -> ("Label.Text"=w801:string)  [unwired: 1 in, 2 out]
                    n428 = Unbundle By Name(w806) -> ("Tmp_C"=w803:refnum<queue>)
                    n429 = Bundle(cluster=T50 {"Heater"="None", "Tmp [K]"=0.0} ("Set point"), "Heater"=w801, "Tmp [K]"=w800) -> (w797:T50)
                    n430 = Bundle By Name(cluster=T52 {"Command"=enum."Initialize", "Data"=variant}, "Command"=TC_commands."Set point", "Data"=w797) -> (w804:T52)
                    n431 = call "Put in mailbox.vi"("Message"=w804, "Queue in"=w803) -> ()  [unwired: 7 in, 3 out]
                  }
                  event "SMU controls.Apply": Value Change {
                    n432 = event-data() -> ()  [unwired: 1 in, 5 out]
                    n433 = Unbundle By Name(w811) -> ("Field_M"=w813:refnum<queue>)
                    n434 = Bundle By Name(cluster="SMU controls", "Apply"=FALSE) -> (w812:T14)
                    n435 = Unbundle By Name(w812) -> ("Measurement settings"=w808:T13)
                    n436 = local write "SMU controls"(w812) -> ()
                    n437 = Bundle By Name(cluster=T53 {"Command"=enum."Set measurement", "Data"=variant} ("MSG to Source meter"), "Data"=w808) -> (w809:T53)
                    n438 = call "Put in mailbox.vi"("Message"=w809, "Queue in"=w813) -> ()  [unwired: 7 in, 3 out]
                  }
                  event "SMU controls.Record": Value Change {
                    n439 = event-data() -> ()  [unwired: 1 in, 6 out]
                    n440 = local read "SMU controls"() -> (w822:T14)
                    n441 = Unbundle By Name(w817) -> ("Field_M"=w819:refnum<queue>)
                    n442 = Bundle By Name(cluster=w822, "Record"=FALSE ("Apply")) -> (w821:T14)
                    n443 = call "Put in mailbox.vi"("Message"=T53 {"Command"=enum."Start measurement", "Data"=variant} ("MSG to Source meter"), "Queue in"=w819) -> ()  [unwired: 7 in, 3 out]
                    n444 = local write "SMU controls"(w821) -> ()
                  }
                  event "SMU controls.Stop": Value Change {
                    n445 = event-data() -> ()  [unwired: 1 in, 6 out]
                    n446 = Unbundle By Name(w826) -> ("Field_M"=w825:refnum<queue>)
                    n447 = local read "SMU controls"() -> (w829:T14)
                    n448 = call "Put in mailbox.vi"("Message"=T53 {"Command"=enum."Stop measurement", "Data"=variant} ("MSG to Source meter"), "Queue in"=w825) -> ()  [unwired: 7 in, 3 out]
                    n449 = Bundle By Name(cluster=w829, "Stop"=FALSE ("Apply")) -> (w828:T14)
                    n450 = local write "SMU controls"(w828) -> ()
                  }
                  event "Password": Value Change {
                    n451 = event-data() -> ("NewVal"=w835:string)  [unwired: 1 in, 1 out]
                    n452 = Equal?(x="admin", y=w835) -> (x = y?=w831:bool)
                    n453 = case shown="False" w831 {
                      tunnel: [T33."Disabled and Grayed Out" ("Disabled") T33."Enabled" ("Disabled")] -> w832
                      frame False {
                      }
                      frame True {
                      }
                    }
                    n454 = local read "Instr control refs"() -> (w833:refnum<vi>[])
                    n455 = call "Dis- or en- able controls.vi"("Disabled"=w832, "Control referencies"=w833) -> ()  [unwired: 9 in, 1 out]
                  }
                }
              }
              frame "CW measurement" {
                n456 = event shown="[3] \"Script Array\": Value Change" {
                  selector: _ -> [_ _ _ _ _ _]
                  dyn-events: _ -> [_ _ _ _ _ _]
                  timeout: 0 -> [_ _ _ _ _ _]
                  tunnel: w846 -> [w849 w868 w899 w931 w969 w975]
                  tunnel: [w849 w867 w899 w931 w969 w975] -> w845
                  tunnel: w843 -> [_ _ w898 _ _ _]
                  tunnel: [w847 w863 w895 w930 w966 w974] -> w842
                  tunnel: w841 -> [w847 w860 w895 w930 w966 w974]
                  tunnel: [w848 w864 w894 w929 w965 w973] -> w839
                  tunnel: w840 -> [w848 w865 w893 w929 w965 w973]
                  event Timeout {
                    n457 = event-data() -> ()  [unwired: 1 in, 3 out]
                  }
                  event "Run script btn": Value Change {
                    n458 = event-data() -> ()  [unwired: 1 in, 6 out]
                    n459 = local read "Script Array"() -> (w866:T26[])
                    n460 = local read "THz control"() -> (w858:T21)
                    n461 = Unbundle By Name(w858) -> ("AMC"=w856:u16, "Multip"=w857:u16)
                    n462 = Multiply(x=w856, y=w857) -> (x*y=w855:u16)
                    n463 = for {
                      tunnel: w866 -> [w873] mode=indexing
                      tunnel: [w872] -> w862
                      tunnel: [w873] -> w861
                      tunnel: [w871] -> w859
                      tunnel: w855 -> [w870]
                      tunnel: [w869] -> w853
                      i -> [w871]
                      stop <- w872 stop-if-true
                      n464 = local read "Instr status"() -> (w874:T1)
                      n465 = call "verify executabiity of line.vi"("Freq multiplication factor"=w870, "Instr status"=w874, "Script cluster"=w873) -> ("Response"=w869:string, "is executable"=w872:bool)  [unwired: 7 in]
                    }
                    n466 = One Button Dialog(message="Absorbers!!!", button name ("OK")="OK, run measurement!") -> (true=w852:bool)
                    n467 = case shown="False" w862 {
                      tunnel: w865 -> [w879 w888]
                      tunnel: [w879 w887] -> w864
                      tunnel: [w878 w885] -> w863
                      tunnel: w861 -> [_ w885]
                      tunnel: w860 -> [w878 _]
                      tunnel: w859 -> [_ w883]
                      tunnel: [w876 w881] -> w854
                      tunnel: w853 -> [w877 _]
                      tunnel: w852 -> [_ _]
                      frame False {
                        n468 = Concatenate Strings("Line is not executable beause:" ("string"), w877) -> (w876:string)
                      }
                      frame True {
                        n469 = local read "Controls referencies"() -> (w889:T2)
                        n470 = Unbundle By Name(w889) -> ("To disable"=w880:refnum<vi>[])
                        n471 = Build Array(w883) -> (w884:i32[])
                        n472 = Bundle By Name(cluster=w888, "Experiment state"=experiment_state."Preparation" ("Value")) -> (w887:T24)
                        n473 = Format Into String(format string="%d sctrip lines skipped", w883) -> (resulting string=w881:string)  [unwired: 2 in, 1 out]
                        n474 = property on="Script Array" class="Arr (strict)"("Selection Start []"=w884) -> ()  [unwired: 2 in, 2 out]
                        n475 = call "Dis- or en- able controls.vi"("Disabled"=T33."Disabled and Grayed Out", "Control referencies"=w880) -> ()  [unwired: 9 in, 1 out]
                      }
                    }
                    n476 = call "simple Shift string array.vi"("Element in"=w854, "Array in"=w868) -> ("Array out"=w867:string[])  [unwired: 8 in, 1 out]
                  }
                  event "Direct stop meas. btn": Value Change {
                    n477 = event-data() -> ("NewVal"=w897:bool)  [unwired: 1 in, 5 out]
                    n478 = call "Timeout dialoge Abbort.vi"("Enable"=w897, "Message to Display"="Realy abbort measurement?", "timeout[ms]"=u32 5000) -> ("Yes"=w896:bool)  [unwired: 15 in, 1 out]
                    n479 = case shown="True" w896 {
                      tunnel: w898 -> [_ w917]
                      tunnel: w893 -> [w900 w904]
                      tunnel: [w900 w903] -> w894
                      frame False {
                      }
                      frame True {
                        n480 = Unbundle By Name(w917) -> ("Field_C"=w911:refnum<queue>, "Tmp_C"=w912:refnum<queue>, "Angle_C"=w913:refnum<queue>)
                        n481 = local read "Controls referencies"() -> (w906:T2)
                        n482 = local write "Run script btn"(FALSE ("Direct stop meas. btn")) -> ()
                        n483 = Bundle By Name(cluster=w904, "Experiment state"=experiment_state."Save" ("Value")) -> (w903:T24)
                        n484 = Unbundle By Name(w906) -> ("To disable"=w907:refnum<vi>[])
                        n485 = call "Put in mailbox.vi"("Message"=T37 {"Command"=enum."Stop ramping", "Data"=variant} ("MSG to magnet"), "Queue in"=w911) -> ("error out"=w910:errorcluster)  [unwired: 7 in, 2 out]
                        n486 = call "Put in mailbox.vi"("error in (no error)"=w910, "Message"=T52 {"Command"=enum."Stop tmp change", "Data"=variant} ("MSG for VTI"), "Queue in"=w912) -> ("error out"=w909:errorcluster)  [unwired: 6 in, 2 out]
                        n487 = call "Put in mailbox.vi"("error in (no error)"=w909, "Message"=T40 {"Command"=enum."Stop movement", "Data"=variant} ("MSG to rotator"), "Queue in"=w913) -> ("error out"=w901:errorcluster)  [unwired: 6 in, 2 out]
                        n488 = call "Dis- or en- able controls.vi"("error in"=w901, "Disabled"=T33."Enabled", "Control referencies"=w907) -> ()  [unwired: 8 in, 1 out]
                      }
                    }
                  }
                  event "Script Array": Value Change {
                    # "Verification of values"
                    n489 = event-data() -> ("OldVal"=w924:T26[], "NewVal"=w923:T26[])  [unwired: 1 in, 2 out]
                    n490 = local read "THz control"() -> (w922:T21)
                    n491 = Unbundle By Name(w922) -> ("AMC"=w920:u16, "Multip"=w921:u16)
                    n492 = Array Size(array=w923) -> (size(s)=w927:i32)
                    n493 = Array Size(array=w924) -> (size(s)=w926:i32)
                    n494 = Multiply(x=w920, y=w921) -> (x*y=w919:u16)
                    n495 = Equal?(x=w926, y=w927) -> (x = y?=w925:bool)
                    n496 = case shown="False" w925 {
                      tunnel: w924 -> [w936 w954]
                      tunnel: w923 -> [w937 w953]
                      tunnel: [w935 w952] -> w918
                      tunnel: w926 -> [w938 _]
                      tunnel: w927 -> [w939 _]
                      tunnel: T55 {"min synth f"=9.0, "max synth f"=14.0, "Ramp limits [mT/s]"=[7.5, 5.5, 4.2, 3.1, 1.5], "Field ranges [T]"=[3.0, 9.6, 13.3, 15.5, 16.0]} ("Limits") -> [w933 w951]
                      tunnel: w919 -> [w932 w950]
                      frame False {
                        n497 = Greater?(x=w938, y=w939) -> (0:w934:bool)
                        n498 = case shown="False" w934 {
                          tunnel: w937 -> [w940 w945]
                          tunnel: [w940 w941] -> w935
                          tunnel: w936 -> [_ w943]
                          tunnel: w933 -> [_ w948]
                          tunnel: w932 -> [_ w947]
                          frame True {
                          }
                          frame False {
                            n499 = Reverse 1D Array(array=w945) -> (reversed array=w946:T26[])
                            n500 = Index Array(array=w946) -> (element=w944:T26)  [unwired: 1 in]
                            n501 = call "Check polymorh script.vi"("Multipl factor"=w947, "Limits"=w948, "New val"=w944, "Old val"=T26 {"Start"=0.0, "Start Caption"="Start [T]", "End"=0.0, "End Caption"="End [T]", "Sweep"=0.0, "Sweep caption"="Rate [mT/s]", "Constant"=-1.0, "Constant caption"="Freq [GHz]", "Mod_F [kHz]"=0.1, "Mod_A [G]"=0.0, "Tau [ms]"=0.0, "Positioners [mm|°]"=[-1.0], "Tmp [K]"=0.0, "Wait [min]"=0.0, "Carousel"=-1, "Comment"="", "Auto-mod"=TRUE, "Execute"=FALSE} ("Old Row")) -> ("Row out"=w942:T26)  [unwired: 7 in]
                            n502 = Insert Into Array(array=w943, new element=w942) -> (w941:T26[])  [unwired: 1 in]
                          }
                        }
                      }
                      frame True {
                        n503 = for {
                          tunnel: w954 -> [w959] mode=indexing
                          tunnel: w953 -> [w958] mode=indexing
                          tunnel: [w957] -> w952 mode=indexing
                          tunnel: w951 -> [w956]
                          tunnel: w950 -> [w955]
                          n504 = call "Check polymorh script.vi"("Multipl factor"=w955, "Limits"=w956, "New val"=w958, "Old val"=w959) -> ("Row out"=w957:T26)  [unwired: 7 in]
                        }
                      }
                    }
                    n505 = local write "Script Array"(w918) -> ()
                  }
                  event "Sample name", "Global comment": Value Change {
                    n506 = event-data() -> ("CtlRef"=w964:refnum<vi>, "NewVal"=w968:string)  [unwired: 1 in, 4 out]
                    n507 = Search and Replace String(replace all?=TRUE ("replace all? (F)"), input string=w968, search string="[<>:\"/\\|?*%]" ("regular expression"), replace string="-" ("replace string (\"\")")) -> (result string=w962:string)  [unwired: 4 in, 3 out]
                    n508 = call <vilib>:"Space Constant.vi"() -> ("String"=w961:string)
                    n509 = Search and Replace String(input string=w962, search string="\r\n", replace string=w961) -> (result string=w963:string)  [unwired: 5 in, 3 out]
                    n510 = property class="Str"(reference=w964, "Value"=w963) -> ()  [unwired: 1 in, 2 out]
                  }
                  event "Paste from Editor": Value Change {
                    n511 = event-data() -> ()  [unwired: 1 in, 6 out]
                    n512 = local read "Edited script"() -> (w972:T26[])
                    n513 = local write "Script Array"(w972) -> ()
                  }
                }
              }
              frame "Script Editor" {
                n514 = event shown="[1] \"Generate Script btn\": Value Change" {
                  selector: _ -> [_ _ _ _ _ _ _ _ _ _ _]
                  dyn-events: _ -> [_ _ _ _ _ _ _ _ _ _ _]
                  timeout: 0 -> [_ _ _ _ _ _ _ _ _ _ _]
                  event Timeout {
                    n515 = event-data() -> ()  [unwired: 1 in, 3 out]
                  }
                  event "Generate Script btn": Value Change {
                    n516 = event-data() -> ()  [unwired: 1 in, 4 out]
                    n517 = local read "Edited script"() -> (w983:T26[])
                    n518 = call "Generate script array elements.vi"("Script in"=w983, "Generator options"="Generator options", "Prototype line"="Prototype line") -> ("Script out"=w982:T26[])  [unwired: 2 in]
                    n519 = Array Size(array=w982) -> (size(s)=w986:i32)
                    n520 = case shown="1, Default" w986 {
                      selector: w986 -> [w987 w989]
                      tunnel: [w987 w988] -> w985
                      tunnel: [w987 w990] -> w984
                      frame 0 {
                      }
                      frame 1, Default {
                        n521 = Decrement(x=w989) -> (x-1=w988:i32)
                        n522 = Negate(x=w989) -> (-x=w990:i32)
                      }
                    }
                    n523 = local write "Edited script"(w982) -> ()
                    n524 = property on="Select line" class="DigNum (strict)"("Maximum"=w985, "Minimum"=w984) -> ()  [unwired: 2 in, 2 out]
                  }
                  event "Load script btn": Value Change {
                    n525 = event-data() -> ()  [unwired: 1 in, 3 out]
                    n526 = local read "THz control"() -> (w995:T21)
                    n527 = call "Load script file.vi"() -> ("Array"=w991:T26[], "Multiplication factor"=w992:i32)  [unwired: 10 in]
                    n528 = Unbundle By Name(w995) -> ("AMC"=w996:u16, "Multip"=w997:u16)
                    n529 = Array Size(array=w991) -> (size(s)=w998:i32)
                    n530 = Multiply(x=w996, y=w997) -> (x*y=w993:u16)
                    n531 = Greater Than 0?(x=w998) -> (x > 0?=w1001:bool)
                    n532 = Not Equal?(x=w993, y=w992) -> (x != y?=w994:bool)
                    n533 = case shown="True" w1001 {
                      tunnel: w991 -> [_ w1011]
                      frame False {
                      }
                      frame True {
                        n534 = local write "Edited script"(w1011) -> ()
                      }
                    }
                    n535 = case shown="1, Default" w998 {
                      selector: w998 -> [w1007 w1009]
                      tunnel: [w1007 w1008] -> w1000
                      tunnel: [w1007 w1010] -> w999
                      frame 0 {
                      }
                      frame 1, Default {
                        n536 = Negate(x=w1009) -> (-x=w1010:i32)
                        n537 = Decrement(x=w1009) -> (x-1=w1008:i32)
                      }
                    }
                    n538 = case shown="True" w994 {
                      tunnel: w993 -> [_ w1004]
                      tunnel: w992 -> [_ w1003]
                      frame False {
                      }
                      frame True {
                        n539 = Format Into String(format string="Actual multiplication factor is %d, but in script is %d.", initial string="Warning!\n", w1004, w1003) -> (resulting string=w1002:string)  [unwired: 1 in, 1 out]
                        n540 = One Button Dialog(message=w1002) -> ()  [unwired: 1 in, 1 out]
                      }
                    }
                    n541 = property on="Select line" class="DigNum (strict)"("Maximum"=w1000, "Minimum"=w999) -> ()  [unwired: 2 in, 2 out]
                  }
                  event "Remove from script btn": Value Change {
                    n542 = event-data() -> ()  [unwired: 1 in, 6 out]
                    n543 = local read "Edited script"() -> (w1023:T26[])
                    n544 = local read "Select line"() -> (w1013:i32)
                    n545 = Decrement(x=w1013) -> (x-1=w1012:i32)
                    n546 = Array Size(array=w1023) -> (size(s)=w1021:i32)
                    n547 = Build Array(w1012) -> (w1014:i32[])
                    n548 = Add(x=w1021, y=w1013) -> (x+y=w1020:i32)
                    n549 = Less Than 0?(x=w1013) -> (x < 0?=w1022:bool)
                    n550 = local write "Select line"(w1012) -> ()
                    n551 = Select(t=w1020, s=w1022, f=w1013) -> (s? t:f=w1019:i32)
                    n552 = property on="Edited script" class="Arr (strict)"("Selection Start []"=w1014) -> ()  [unwired: 2 in, 2 out]
                    n553 = Delete From Array(array=w1023, index=w1019) -> (array with subset deleted=w1015:T26[])  [unwired: 1 in, 1 out]
                    n554 = Array Size(array=w1015) -> (size(s)=w1016:i32)
                    n555 = local write "Edited script"(w1015) -> ()
                    n556 = case shown="1, Default" w1016 {
                      selector: w1016 -> [w1024 w1026]
                      tunnel: [w1024 w1025] -> w1018
                      tunnel: [w1024 w1027] -> w1017
                      frame 0 {
                      }
                      frame 1, Default {
                        n557 = Decrement(x=w1026) -> (x-1=w1025:i32)
                        n558 = Negate(x=w1026) -> (-x=w1027:i32)
                      }
                    }
                    n559 = property on="Select line" class="DigNum (strict)"("Maximum"=w1018, "Minimum"=w1017) -> ()  [unwired: 2 in, 2 out]
                  }
                  event "Clear script btn": Value Change {
                    n560 = event-data() -> ()  [unwired: 1 in, 6 out]
                    n561 = local write "Edited script"(T26[] [] ("Edited script")) -> ()
                  }
                  event "Set as adj tab btn": Value Change {
                    n562 = event-data() -> ()  [unwired: 1 in, 4 out]
                    n563 = local read "Acquisition controls"() -> (w1033:T18)
                    n564 = local read "Magnet controls"() -> (w1037:T23)
                    n565 = local read "THz control"() -> (w1035:T21)
                    n566 = Unbundle By Name(w1035) -> ("Base frequency [GHz]"=w1034:dbl)
                    n567 = Unbundle By Name(w1033) -> ("ACQ parameters.F_Mod [kHz]"=w1030:dbl, "ACQ parameters.Filter tau [ms]"=w1031:dbl, "Desired [G]"=w1032:dbl, "Auto-modulation"=w1029:bool)
                    n568 = Unbundle By Name(w1037) -> ("Set Field [T]"=w1036:dbl)
                    n569 = Bundle By Name(cluster=T26 {"Start"=0.0, "Start Caption"="Start [T]", "End"=0.0, "End Caption"="End [T]", "Sweep"=3.0, "Sweep caption"="Rate [mT/s]", "Constant"=210.0, "Constant caption"="Freq [GHz]", "Mod_F [kHz]"=69.1, "Mod_A [G]"=1.0, "Tau [ms]"=100.0, "Positioners [mm|°]"=[-1.0], "Tmp [K]"=2.0, "Wait [min]"=0.1, "Carousel"=0, "Comment"="No comment", "Auto-mod"=TRUE, "Execute"=TRUE} ("Prototype line"), "Start"=w1036, "Constant"=w1034, "Mod_F [kHz]"=w1030, "Tau [ms]"=w1031, "Mod_A [G]"=w1032, "Auto-mod"=w1029) -> (w1038:T26)
                    n570 = local write "Prototype line"(w1038) -> ()
                  }
                  event "Select line": Value Change {
                    n571 = event-data() -> ("CtlRef"=w1040:refnum<vi>)  [unwired: 1 in, 5 out]
                    n572 = Less Than 0?(x="Select line") -> (x < 0?=w1045:bool)
                    n573 = case shown="False" w1045 {
                      tunnel: "Select line" -> [w1047 w1048]
                      tunnel: w1040 -> [_ w1053]
                      tunnel: [w1047 w1051] -> w1042
                      frame False {
                      }
                      frame True {
                        n574 = property class="DigNum (strict)"(reference=w1053) -> ("Maximum"=w1052:dbl)  [unwired: 1 in, 2 out]
                        n575 = To Long Integer(number=w1052) -> (32bit integer=w1050:i32)
                        n576 = Increment(x=w1050) -> (x+1=w1049:i32)
                        n577 = Add(x=w1048, y=w1049) -> (x+y=w1051:i32)
                      }
                    }
                    n578 = To Unsigned Long Integer(number=w1042) -> (unsigned 32bit integer=w1043:u32)
                    n579 = Build Array(w1043) -> (w1046:u32[])
                    n580 = property on="Edited script" class="Arr (strict)"("Selection Start []"=w1046, "Selection Size []"=u32[] [1] ("Selection Size[]")) -> ()  [unwired: 2 in, 2 out]
                  }
                  event "Edited script": Mouse Down {
                    n581 = event-data() -> ("CtlRef"=w1054:refnum<vi>)  [unwired: 1 in, 7 out]
                    n582 = property class="Arr (strict)"(reference=w1054) -> (reference out=w1065:refnum<vi>, "Index Values"=w1061:u32[], "Array Element.Top"=w1059:i32, "Top"=w1058:i32, "Array Element.Height"=w1057:u32)  [unwired: 1 in, 1 out]
                    n583 = Subtract(x=w1059, y=w1058) -> (x-y=w1060:i32)
                    n584 = Index Array(array=w1061) -> (element=w1062:u32)  [unwired: 1 in]
                    n585 = Quotient & Remainder(x=w1060, y=w1057) -> (floor(x/y)=w1063:u32)  [unwired: 1 out]
                    n586 = Add(x=w1062, y=w1063) -> (x+y=w1056:u32)
                    n587 = Build Array(w1056) -> (w1064:u32[])
                    n588 = property class="Arr (strict)"(reference=w1065, "Selection Size []"=u32[] [1] ("Selection Size[]"), "Selection Start []"=w1064) -> ()  [unwired: 1 in, 2 out]
                    n589 = local write "Select line"(w1056) -> ()
                  }
                  event "Edited script": Value Change {
                    n590 = event-data() -> ("NewVal"=w1066:T26[])  [unwired: 1 in, 5 out]
                    n591 = Array Size(array=w1066) -> (size(s)=w1067:i32)
                    n592 = case shown="1, Default" w1067 {
                      selector: w1067 -> [w1070 w1072]
                      tunnel: [w1070 w1071] -> w1069
                      tunnel: [w1070 w1073] -> w1068
                      frame 0 {
                      }
                      frame 1, Default {
                        n593 = Decrement(x=w1072) -> (x-1=w1071:i32)
                        n594 = Negate(x=w1072) -> (-x=w1073:i32)
                      }
                    }
                    n595 = property on="Select line" class="DigNum (strict)"("Maximum"=w1069, "Minimum"=w1068) -> ()  [unwired: 2 in, 2 out]
                  }
                  event "Save script file btn": Value Change {
                    n596 = event-data() -> ()  [unwired: 1 in, 6 out]
                    n597 = local read "THz control"() -> (w1078:T21)
                    n598 = Unbundle By Name(w1078) -> ("AMC"=w1077:u16, "Multip"=w1076:u16)
                    n599 = Multiply(x=w1077, y=w1076) -> (x*y=w1075:u16)
                    n600 = call "Save script file.vi"("Multiplication factor"=w1075, "Script Array"="Edited script") -> ()  [unwired: 10 in]
                  }
                  event "Paste from meeasurrement": Value Change {
                    n601 = event-data() -> ()  [unwired: 1 in, 6 out]
                    n602 = local read "Script Array"() -> (w1079:T26[])
                    n603 = local write "Edited script"(w1079) -> ()
                  }
                }
              }
              frame "Measurement review" {
                n604 = event shown="[1] \"Data file to show\": Value Change" {
                  selector: _ -> [_ _ _ _]
                  dyn-events: _ -> [_ _ _ _]
                  timeout: 0 -> [_ _ _ _]
                  event Timeout {
                    n605 = event-data() -> ()  [unwired: 1 in, 3 out]
                  }
                  event "Data file to show": Value Change {
                    n606 = event-data() -> ("Type"=w1089:T78)  [unwired: 1 in, 3 out]
                    n607 = Format Into String(w1089) -> ()  [unwired: 3 in, 2 out]
                    n608 = local read "Results"() -> (w1088:T5)
                    n609 = Build Array("Data file to show") -> (w1090:u16[])
                    n610 = property on="Header" class="Arr (strict)"("Index Values"=w1090) -> ()  [unwired: 2 in, 2 out]
                    n611 = Index Array(array=w1088, index="Data file to show") -> (element=w1086:T56)
                    n612 = Unbundle(w1086) -> ("Mode"=w1084:T4, "Array"=w1085:cluster{"Array":dbl[], "Array":dbl[]}[])
                    n613 = case shown="\"MD EPR\", Default" w1084 {
                      frame "MD EPR", Default {
                        n614 = property on="Review Graph" class="XYGraph (strict)"("XScale.NameLbl.Text"="B [T]" ("X Scale.Name Label.Text")) -> ()  [unwired: 2 in, 2 out]
                      }
                      frame "FD EPR" {
                        n615 = property on="Review Graph" class="XYGraph (strict)"("XScale.NameLbl.Text"="F [GHz]" ("X Scale.Name Label.Text")) -> ()  [unwired: 2 in, 2 out]
                      }
                    }
                    n616 = local write "Review Graph"(w1085) -> ()
                  }
                  event "Open measurement": Value Change {
                    n617 = event-data() -> ()  [unwired: 1 in, 1 out]
                    n618 = local read "Main data folder"() -> (w1093:path)
                    n619 = call "Read data file.vi"("Application Directory"=w1093) -> ("Graph data"=w1095:cluster{"Array":dbl[], "Array":dbl[]}[], "Header"=w1097:string, "Mode"=w1096:T4, "Name"=w1098:string, "Error Out"=w1094:errorcluster)  [unwired: 6 in]
                    n620 = case shown="No Error" w1094 {
                      tunnel: w1098 -> [w1111 _]
                      tunnel: w1097 -> [w1106 _]
                      tunnel: w1096 -> [w1099 _]
                      tunnel: w1095 -> [w1101 _]
                      frame No Error {
                        n621 = local read "Data file to show"() -> (w1102:u16)
                        n622 = Bundle(cluster=T56 {"Mode"=enum."MD EPR", "Array"=[]} ("Cluster 2"), "Mode"=w1099, "Array"=w1101) -> (w1104:T56)
                        n623 = local read "Header"() -> (w1108:string[])
                        n624 = local read "Results"() -> (w1105:T5)
                        n625 = property on="Data file to show" class="Ring (strict)"() -> ("Strings []"=w1110:string[])  [unwired: 2 in, 2 out]
                        n626 = Replace Array Subset(array=w1110, new element=w1111, index=w1102) -> (w1109:string[])
                        n627 = Replace Array Subset(array=w1108, new element=w1106, index=w1102) -> (→"Header":string[])
                        n628 = Replace Array Subset(array=w1105, new element=w1104, index=w1102) -> (w1103:T5)
                        n629 = property on="Data file to show" class="Ring (strict)"("Strings []"=w1109) -> ()  [unwired: 2 in, 2 out]
                        n630 = local write "Results"(w1103) -> ()
                        "Review Graph" <- w1101
                      }
                      frame Error {
                      }
                    }
                  }
                  event "Shift data btn": Value Change {
                    n631 = event-data() -> ()  [unwired: 1 in, 2 out]
                    n632 = local read "Review Graph"() -> (w1120:cluster{"Array":dbl[], "Array":dbl[]}[])
                    n633 = Boolean To (0,1)(Boolean="Edit Channel") -> (0, 1=w1122:i16)
                    n634 = Index Array(array=w1120, index=w1122) -> (element=w1124:cluster{"Array":dbl[], "Array":dbl[]})
                    n635 = Unbundle(w1124) -> ("Array"=w1116:dbl[], "Array"=w1125:dbl[])
                    n636 = Array Max & Min(array=w1116) -> (max value=w1115:dbl, min value=w1114:dbl)  [unwired: 2 out]
                    n637 = Subtract(x=w1115, y=w1114) -> (x-y=w1113:dbl)
                    n638 = for {
                      tunnel: w1116 -> [w1138] mode=indexing
                      tunnel: "From point [T]" -> [w1139]
                      shift-right: [w1135] -> w1112
                      shift-left: -1 -> [w1134]
                      shift-right: [w1133] -> _
                      shift-left: w1113 -> [w1130]
                      i -> [w1136]
                      n639 = Subtract(x=w1138, y=w1139) -> (x-y=w1137:dbl)
                      n640 = Absolute Value(x=w1137) -> (abs(x)=w1131:dbl)
                      n641 = Less?(x=w1131, y=w1130) -> (x < y?=w1132:bool)
                      n642 = Select(t=w1131, s=w1132, f=w1130) -> (s? t:f=w1133:dbl)
                      n643 = Select(t=w1136, s=w1132, f=w1134) -> (s? t:f=w1135:i32)
                    }
                    n644 = Array Subset(array=w1125, index=w1112) -> (w1128:dbl[])  [unwired: 1 in]
                    n645 = Add(x=w1128, y="Amlitude shift [-]") -> (x+y=w1126:dbl[])
                    n646 = Replace Array Subset(array=w1125, new element=w1126, index=w1112) -> (w1123:dbl[])
                    n647 = Bundle(cluster=w1124, "Array"=w1116, "Array"=w1123) -> (w1121:cluster{"Array":dbl[], "Array":dbl[]})
                    n648 = Replace Array Subset(array=w1120, new element=w1121, index=w1122) -> (w1119:cluster{"Array":dbl[], "Array":dbl[]}[])
                    n649 = local write "Review Graph"(w1119) -> ()
                  }
                }
              }
              frame "Help" {
              }
            }
          }
          event Value Change {
            n650 = event-data() -> ("NewVal"=w1144:T6)  [unwired: 1 in, 3 out]
            n651 = case shown="\"Adjustment\"" w1144 {
              frame "Page Status", Default {
              }
              frame "Adjustment" {
              }
            }
          }
          event "Disconnect": Value Change {
            n652 = event-data() -> ()  [unwired: 1 in, 6 out]
            n653 = local read "Select module"() -> (w1148:T7)
            n654 = Equal?(x=w1148, y=Module_selection."All") -> (x = y?=w1149:bool)
            n655 = case shown="True" w1149 {
              tunnel: w1147 -> [w1154 w1184]
              tunnel: w1148 -> [w1155 _]
              frame False {
                n656 = case shown="\"MAG\"" w1155 {
                  tunnel: w1154 -> [w1159 w1163 w1167 w1168 w1175 w1179 w1183 _]
                  frame "MAG" {
                    n657 = Unbundle By Name(w1159) -> ("Field_C"=w1157:refnum<queue>)
                    n658 = call "Put in mailbox.vi"("Priority? (F)"=TRUE ("Priority?"), "Message"=T37 {"Command"=enum."Disconnect", "Data"=variant} ("MSG to magnet"), "Queue in"=w1157) -> ()  [unwired: 6 in, 3 out]
                  }
                  frame "VTI" {
                    n659 = Unbundle By Name(w1163) -> ("Tmp_C"=w1161:refnum<queue>)
                    n660 = call "Put in mailbox.vi"("Priority? (F)"=TRUE ("Priority?"), "Message"=T52 {"Command"=enum."Disconnect", "Data"=variant} ("MSG for VTI"), "Queue in"=w1161) -> ()  [unwired: 6 in, 3 out]
                  }
                  frame "THz" {
                    n661 = Unbundle By Name(w1167) -> ("MW_C"=w1165:refnum<queue>)
                    n662 = call "Put in mailbox.vi"("Priority? (F)"=TRUE ("Priority?"), "Message"=T45 {"Command"=enum."Disconnect", "Data"=variant} ("Incoming msg"), "Queue in"=w1165) -> ()  [unwired: 6 in, 3 out]
                  }
                  frame "ACQ" {
                    n663 = Unbundle By Name(w1168) -> ("Data_Aq"=w1170:refnum<queue>)
                    n664 = call "Put in mailbox.vi"("Priority? (F)"=TRUE ("Priority?"), "Message"=T49 {"Command"=enum."Disconnect", "Data"=variant} ("MSG for  ACQ"), "Queue in"=w1170) -> ()  [unwired: 6 in, 3 out]
                  }
                  frame "SERV" {
                    n665 = Unbundle By Name(w1175) -> ("Table_C"=w1173:refnum<queue>)
                    n666 = call "Put in mailbox.vi"("Priority? (F)"=TRUE ("Priority?"), "Message"=T39 {"Command"=enum."Disconnect", "Data"=variant(dbl[] [])} ("MSG to Servo"), "Queue in"=w1173) -> ()  [unwired: 6 in, 3 out]
                  }
                  frame "ROT" {
                    n667 = Unbundle By Name(w1179) -> ("Angle_C"=w1177:refnum<queue>)
                    n668 = call "Put in mailbox.vi"("Priority? (F)"=TRUE ("Priority?"), "Message"=cluster{"Command":T41, "Data":variant} {"Command"=enum."Disconnect", "Data"=variant} ("MSG to rotator"), "Queue in"=w1177) -> ()  [unwired: 6 in, 3 out]
                  }
                  frame "SMU" {
                    n669 = Unbundle By Name(w1183) -> ("Mod_M"=w1181:refnum<queue>)
                    n670 = call "Put in mailbox.vi"("Priority? (F)"=TRUE ("Priority?"), "Message"=T53 {"Command"=enum."Disconnect", "Data"=variant} ("MSG to Source meter"), "Queue in"=w1181) -> ()  [unwired: 6 in, 3 out]
                  }
                  frame "None", Default {
                  }
                }
              }
              frame True {
                n671 = control-ref of="Instr status"() -> (w1185:refnum<vi>)
                n672 = property class="Clust (strict)"(reference=w1185) -> ("Controls[]"=w1186:refnum<vi>[])  [unwired: 1 in, 2 out]
                n673 = for {
                  tunnel: w1186 -> [w1192] mode=indexing
                  tunnel: w1184 -> [w1190]
                  n674 = property class="Ctl"(reference=w1192) -> ("Label.Text"=w1191:string, "Value"=w1189:variant)  [unwired: 1 in, 2 out]
                  n675 = Variant To Data(type=FALSE, Variant=w1189) -> (data=w1187:bool)  [unwired: 1 in, 1 out]
                  n676 = case shown="True" w1187 {
                    tunnel: w1191 -> [_ w1194]
                    tunnel: w1190 -> [_ w1193]
                    frame False {
                    }
                    frame True {
                      n677 = case shown="\"MFLI\"" w1194 {
                        tunnel: w1193 -> [w1198 w1202 w1206 w1210 w1214 w1218 w1222 _]
                        frame "Mag" {
                          n678 = Unbundle By Name(w1198) -> ("Field_C"=w1196:refnum<queue>)
                          n679 = call "Put in mailbox.vi"("Priority? (F)"=TRUE ("Priority?"), "Message"=T37 {"Command"=enum."Disconnect", "Data"=variant} ("MSG to magnet"), "Queue in"=w1196) -> ()  [unwired: 6 in, 3 out]
                        }
                        frame "SMU" {
                          n680 = Unbundle By Name(w1202) -> ("Mod_M"=w1200:refnum<queue>)
                          n681 = call "Put in mailbox.vi"("Priority? (F)"=TRUE ("Priority?"), "Message"=T53 {"Command"=enum."Disconnect", "Data"=variant} ("MSG to Source meter"), "Queue in"=w1200) -> ()  [unwired: 6 in, 3 out]
                        }
                        frame "VTI" {
                          n682 = Unbundle By Name(w1206) -> ("Tmp_C"=w1204:refnum<queue>)
                          n683 = call "Put in mailbox.vi"("Priority? (F)"=TRUE ("Priority?"), "Message"=T52 {"Command"=enum."Disconnect", "Data"=variant} ("MSG for VTI"), "Queue in"=w1204) -> ()  [unwired: 6 in, 3 out]
                        }
                        frame "THz" {
                          n684 = Unbundle By Name(w1210) -> ("MW_C"=w1208:refnum<queue>)
                          n685 = call "Put in mailbox.vi"("Priority? (F)"=TRUE ("Priority?"), "Message"=T45 {"Command"=enum."Disconnect", "Data"=variant} ("Incoming msg"), "Queue in"=w1208) -> ()  [unwired: 6 in, 3 out]
                        }
                        frame "MFLI" {
                          n686 = Unbundle By Name(w1214) -> ("Data_Aq"=w1212:refnum<queue>)
                          n687 = call "Put in mailbox.vi"("Priority? (F)"=TRUE ("Priority?"), "Message"=T49 {"Command"=enum."Disconnect", "Data"=variant} ("MSG for  ACQ"), "Queue in"=w1212) -> ()  [unwired: 6 in, 3 out]
                        }
                        frame "Serv" {
                          n688 = Unbundle By Name(w1218) -> ("Table_C"=w1216:refnum<queue>)
                          n689 = call "Put in mailbox.vi"("Priority? (F)"=TRUE ("Priority?"), "Message"=T39 {"Command"=enum."Disconnect", "Data"=variant(dbl[] [])} ("MSG to Servo"), "Queue in"=w1216) -> ()  [unwired: 6 in, 3 out]
                        }
                        frame "Rot" {
                          n690 = Unbundle By Name(w1222) -> ("Angle_C"=w1220:refnum<queue>)
                          n691 = call "Put in mailbox.vi"("Priority? (F)"=TRUE ("Priority?"), "Message"=cluster{"Command":T41, "Data":variant} {"Command"=enum."Disconnect", "Data"=variant} ("MSG to rotator"), "Queue in"=w1220) -> ()  [unwired: 6 in, 3 out]
                        }
                        frame "Ignore", Default {
                        }
                      }
                    }
                  }
                }
              }
            }
          }
          event "Stop": Value Change {
            n692 = event-data() -> ("NewVal"=w1228:bool)  [unwired: 1 in, 5 out]
            n693 = case shown="True" w1228 {
              tunnel: w1227 -> [_ w1232]
              tunnel: [_ w1231] -> w1226
              frame False {
              }
              frame True {
                # "Can not stop application just like that,\nAll modules must respond first, \nthat they are done."
                n694 = control-ref of="Instr status"() -> (w1234:refnum<vi>)
                n695 = property class="Clust (strict)"(reference=w1234) -> ("Value"=w1229:T79)  [unwired: 1 in, 2 out]
                n696 = property class="Clust (strict)"(reference=w1234) -> ("Controls[]"=w1235:refnum<vi>[])  [unwired: 1 in, 2 out]
                n697 = Cluster To Array(cluster=w1229) -> (array=w1233:bool[])
                n698 = Or Array Elements(Boolean array=w1233) -> (logical OR=w1230:bool)
                n699 = for {
                  tunnel: w1235 -> [w1241] mode=indexing
                  tunnel: w1232 -> [w1239]
                  n700 = property class="Ctl"(reference=w1241) -> ("Label.Text"=w1240:string, "Value"=w1238:variant)  [unwired: 1 in, 2 out]
                  n701 = Variant To Data(type=FALSE, Variant=w1238) -> (data=w1236:bool)  [unwired: 1 in, 1 out]
                  n702 = case shown="True" w1236 {
                    tunnel: w1240 -> [_ w1243]
                    tunnel: w1239 -> [_ w1242]
                    frame False {
                    }
                    frame True {
                      n703 = case shown="\"Ignore\", Default" w1243 {
                        tunnel: w1242 -> [w1247 w1251 w1255 w1259 w1263 w1267 w1271 _]
                        frame "Mag" {
                          n704 = Unbundle By Name(w1247) -> ("Field_C"=w1245:refnum<queue>)
                          n705 = call "Put in mailbox.vi"("Priority? (F)"=TRUE ("Priority?"), "Message"=T37 {"Command"=enum."Disconnect", "Data"=variant} ("MSG to magnet"), "Queue in"=w1245) -> ()  [unwired: 6 in, 3 out]
                        }
                        frame "VTI" {
                          n706 = Unbundle By Name(w1251) -> ("Tmp_C"=w1249:refnum<queue>)
                          n707 = call "Put in mailbox.vi"("Priority? (F)"=TRUE ("Priority?"), "Message"=T52 {"Command"=enum."End", "Data"=variant} ("MSG for VTI"), "Queue in"=w1249) -> ()  [unwired: 6 in, 3 out]
                        }
                        frame "THz" {
                          n708 = Unbundle By Name(w1255) -> ("MW_C"=w1253:refnum<queue>)
                          n709 = call "Put in mailbox.vi"("Priority? (F)"=TRUE ("Priority?"), "Message"=T45 {"Command"=enum."End", "Data"=variant} ("Incoming msg"), "Queue in"=w1253) -> ()  [unwired: 6 in, 3 out]
                        }
                        frame "MFLI" {
                          n710 = Unbundle By Name(w1259) -> ("Data_Aq"=w1257:refnum<queue>)
                          n711 = call "Put in mailbox.vi"("Priority? (F)"=TRUE ("Priority?"), "Message"=T49 {"Command"=enum."End", "Data"=variant} ("MSG for  ACQ"), "Queue in"=w1257) -> ()  [unwired: 6 in, 3 out]
                        }
                        frame "Serv" {
                          n712 = Unbundle By Name(w1263) -> ("Table_C"=w1261:refnum<queue>)
                          n713 = call "Put in mailbox.vi"("Priority? (F)"=TRUE ("Priority?"), "Message"=T39 {"Command"=enum."End", "Data"=variant(dbl[] [])} ("MSG to Servo"), "Queue in"=w1261) -> ()  [unwired: 6 in, 3 out]
                        }
                        frame "Rot" {
                          n714 = Unbundle By Name(w1267) -> ("Angle_C"=w1265:refnum<queue>)
                          n715 = call "Put in mailbox.vi"("Priority? (F)"=TRUE ("Priority?"), "Message"=cluster{"Command":T41, "Data":variant} {"Command"=enum."End", "Data"=variant} ("MSG to rotator"), "Queue in"=w1265) -> ()  [unwired: 6 in, 3 out]
                        }
                        frame "SMU" {
                          n716 = Unbundle By Name(w1271) -> ("Mod_M"=w1269:refnum<queue>)
                          n717 = call "Put in mailbox.vi"("Priority? (F)"=TRUE ("Priority?"), "Message"=T53 {"Command"=enum."End", "Data"=variant} ("MSG to Source meter"), "Queue in"=w1269) -> ()  [unwired: 6 in, 3 out]
                        }
                        frame "Ignore", Default {
                        }
                      }
                    }
                  }
                }
                n718 = case shown="False" w1230 {
                  tunnel: w1229 -> [_ _]
                  tunnel: w1232 -> [w1294 _]
                  tunnel: [TRUE _] -> w1231
                  frame False {
                    n719 = Cluster To Array(cluster=w1294) -> (array=w1295:refnum<queue>[])
                    n720 = local read "loggersRef"() -> (w1286:refnum<file>)
                    n721 = for {
                      tunnel: w1295 -> [w1303] mode=indexing
                      tunnel: [w1296] -> w1291
                      n722 = Wait (ms)(milliseconds to wait=u32 100) -> ()  [unwired: 1 out]
                      n723 = Get Queue Status(queue=w1303) -> (queue out=w1302:refnum<queue>, error out=w1297:errorcluster, # elements in queue=w1300:i32)  [unwired: 2 in, 5 out]
                      n724 = Less Or Equal?(x=w1300, y=0) -> (x <= y?=w1298:bool)
                      n725 = Release Queue(queue=w1302, force destroy? (F)=w1298, error in (no error)=w1297) -> (error out=w1296:errorcluster)  [unwired: 2 out]
                    }
                    n726 = Wait (ms)(milliseconds to wait=u32 2000) -> ()  [unwired: 1 out]
                    n727 = local read "Temperature log ref"() -> (w1290:refnum<file>)
                    n728 = call "Add actual date time to string.vi"("String in"="Program ended") -> ("String out"=w1287:string)  [unwired: 4 in]
                    n729 = call "Write in logger.vi"("String in"=w1287, "logger refnum"=w1286) -> ("refnum out"=w1285:refnum<file>)  [unwired: 2 in, 1 out]
                    n730 = local read "System config file path"() -> (w1284:path)
                    n731 = local read "Acquisition controls"() -> (w1281:T18)
                    n732 = local read "THz control"() -> (w1280:T21)
                    n733 = Close File(refnum=w1285, error in=w1291) -> (error out=w1289:errorcluster)  [unwired: 1 out]
                    n734 = Close File(refnum=w1290, error in=w1289) -> ()  [unwired: 2 out]
                    n735 = call "Open config file.vi"("MAG config file path"=w1284) -> ("error out"=w1282:errorcluster, "Refnum out"=w1283:T76)  [unwired: 7 in, 2 out]
                    n736 = Unbundle By Name(w1281) -> ("ACQ parameters"=w1277:T19)
                    n737 = call <userlib>:"Write Section Cluster__ogtk.vi"("error in (no error)"=w1282, "Section Formatted Cluster"=w1280, "refnum"=w1283) -> ("error out"=w1279:errorcluster, "dup refnum"=w1278:T76)  [unwired: 7 in]
                    n738 = local read "Instr info"() -> (w1272:T8)
                    n739 = call <userlib>:"Write Section Cluster__ogtk.vi"("error in (no error)"=w1279, "Section Formatted Cluster"=w1277, "refnum"=w1278) -> ("error out"=w1274:errorcluster, "dup refnum"=w1276:T76)  [unwired: 7 in]
                    n740 = call <userlib>:"Write Section Cluster__ogtk.vi"("error in (no error)"=w1274, "Section Formatted Cluster"=w1272, "refnum"=w1276) -> ("error out"=w1273:errorcluster, "dup refnum"=w1275:T76)  [unwired: 7 in]
                    n741 = call <vilib>:"Close Config Data.vi"("error in (no error)"=w1273, "refnum"=w1275) -> ()  [unwired: 8 in, 2 out]
                  }
                  frame True {
                  }
                }
              }
            }
          }
          event "Re-connect instruments": Value Change {
            n742 = event-data() -> ()  [unwired: 1 in, 4 out]
            n743 = local read "System config file path"() -> (w1305:path)
            n744 = case shown="\"ROT\"" "Select module" {
              tunnel: w1310 -> [w1315 w1324 w1362 _ w1372 w1384 w1391 w1397 w1408]
              tunnel: w1305 -> [w1314 _ w1356 _ _ w1376 _ _ _]
              tunnel: w1309 -> [w1313 w1325 w1363 w1364 w1373 w1385 w1389 w1398 w1405]
              tunnel: [w1313 w1325 w1363 w1364 w1373 w1385 w1389 w1398 w1405] -> w1308
              tunnel: "Use previous settings" -> [_ w1316 _ _ _ _ _ _ _]
              frame "All", Default {
                n745 = call "Send message to initialize all modules.vi"("System config file path"=w1314, "Messenger referencies"=w1315) -> ()  [unwired: 10 in]
                n746 = property on="Select module" class="Enum (strict)"("DisabledEnum"=T33."Enabled" ("Disabled")) -> ()  [unwired: 2 in, 2 out]
              }
              frame "ACQ" {
                w1317 = T49 {"Command"=enum."Initialize", "Data"=variant} ("MSG for  ACQ")
                n747 = Unbundle By Name(w1324) -> ("Data_Aq"=w1321:refnum<queue>)
                n748 = Bundle By Name(cluster=w1317, "Command"=MFLI_command_enum."Initialize", "Data"="MF-DEV4029") -> (w1322:T49)
                n749 = call "Put in mailbox.vi"("Priority? (F)"=TRUE, "Message"=w1322, "Queue in"=w1321) -> ("Queue out"=w1318:refnum<queue>)  [unwired: 6 in, 2 out]
                n750 = case shown="True" w1316 {
                  tunnel: w1318 -> [_ w1347]
                  tunnel: w1317 -> [_ w1345]
                  frame False {
                  }
                  frame True {
                    w1334 = T46 {"parameter"=enum."filter_order [-]", "value"=0.0} ("Parameter to set")
                    n751 = local read "Acquisition controls"() -> (w1343:T18)
                    n752 = Unbundle By Name(w1343) -> ("ACQ parameters"=w1330:T19)
                    n753 = Unbundle By Name(w1330) -> ("Filter order"=w1342:dbl, "Filter tau [ms]"=w1341:dbl, "F_Mod [kHz]"=w1340:dbl, "Amp_Mod [mV]"=w1339:dbl)
                    n754 = Divide(x=w1339, y=1000.0) -> (x/y=w1338:dbl)
                    n755 = Bundle(cluster=w1334, "parameter"=MFLI_node."osc_freq [kHz]", "value"=w1340) -> (w1332:T46)
                    n756 = Bundle(cluster=w1334, "parameter"=MFLI_node."filter_constant [ms]", "value"=w1341) -> (w1333:T46)
                    n757 = Bundle(cluster=w1334, "parameter"=MFLI_node."out_ampl [V]", "value"=w1338) -> (w1336:T46)
                    n758 = Bundle(cluster=w1334, "parameter"=MFLI_node."filter_order [-]", "value"=w1342) -> (w1335:T46)
                    n759 = Build Array(w1335, w1333, w1332, w1336) -> (w1331:T46[])
                    n760 = Bundle By Name(cluster=w1345, "Command"=MFLI_command_enum."Set individual parameters", "Data"=w1331) -> (w1346:T49)
                    n761 = call "Put in mailbox.vi"("Message"=w1346, "Queue in"=w1347) -> ()  [unwired: 7 in, 3 out]
                  }
                }
              }
              frame "MAG" {
                n762 = call "Read magnet system configuration.vi"("MAG config file path"=w1356) -> ("error out"=w1358:errorcluster, "Magnet Constantsout"=w1354:T80)  [unwired: 8 in, 1 out]
                n763 = Unbundle By Name(w1362) -> ("Field_C"=w1357:refnum<queue>)
                n764 = Unbundle By Name(w1354) -> ("Maximum field [T]"=w1353:dbl, "Field Constant [T/A]"=w1351:dbl, "Ramp limits [A/s]"=w1352:dbl[])
                n765 = Bundle By Name(cluster=T37 {"Command"=enum."Connect", "Data"=variant(enum16{"Ramping", "Perzistant"} enum."Ramping")} ("MSG to magnet"), "Command"=Magnet_Orders."Connect" ("Order"), "Data"=w1354) -> (w1360:T37)
                n766 = Index Array(array=w1352) -> (element=w1350:dbl)  [unwired: 1 in]
                n767 = call "Put in mailbox.vi"("Priority? (F)"=TRUE, "error in (no error)"=w1358, "Message"=w1360, "Queue in"=w1357) -> ()  [unwired: 5 in, 3 out]
                n768 = Compound Arithmetic op=MULTIPLY(w1351, w1350, 1000.0 ("value")) -> (w1348:dbl)
                n769 = property on="Set Field [T]" class="DigNum (strict)"("Maximum"=w1353) -> ()  [unwired: 2 in, 2 out]
                n770 = property on="Desired ramp\nrate [mT/s]" class="DigNum (strict)"("Maximum"=w1348) -> ()  [unwired: 2 in, 2 out]
              }
              frame "None" {
              }
              frame "ROT" {
                n771 = Unbundle By Name(w1372) -> ("Angle_C"=w1369:refnum<queue>)
                n772 = disable-structure shown="TARGET_BITNESS==64, Default" {
                  disable-tunnel: [path "C:/Program Files/National Instruments/LabVIEW 2024/instr.lib/ANC350/Win32/anc350v4.dll" ("File Path Control") path "C:/Programs/Debug/ANC350 lib/Software_ANC350v4/Windows/ANC350_Library/lib64/anc350v4.dll" ("File Path Control")] -> w1365
                  frame condition #0 {
                  }
                  frame condition #1 (active) {
                  }
                }
                n773 = Build Array (concatenate)(w1365, path[] [path "C:/Programs/Debug/HFEPR spectrometer SW 2024/Multi-HFEPR app/SystemData/ANRv51-C4-124.LUT"] ("File Path Control")) -> (w1367:path[])
                n774 = Bundle By Name(cluster=T40 {"Command"=enum."Initialize", "Data"=variant} ("MSG to rotator"), "Command"=Rotator_commands."Initialize", "Data"=w1367) -> (w1371:T40)
                n775 = call "Put in mailbox.vi"("Message"=w1371, "Queue in"=w1369) -> ()  [unwired: 7 in, 3 out]
              }
              frame "SERV" {
                n776 = Unbundle By Name(w1384) -> ("Table_C"=w1377:refnum<queue>)
                n777 = call "Servo Read system configuration.vi"("MAG config file path"=w1376) -> ("error out"=w1381:errorcluster, "IP addresses"=w1382:string[])  [unwired: 8 in, 1 out]
                n778 = Bundle By Name(cluster=T39 {"Command"=enum."Initialize", "Data"=variant(dbl[] [])} ("MSG to Servo"), "Command"=Servo_commands."Initialize", "Data"=w1382) -> (w1383:T39)
                n779 = call "Put in mailbox.vi"("Priority? (F)"=TRUE, "error in (no error)"=w1381, "Message"=w1383, "Queue in"=w1377) -> ()  [unwired: 5 in, 3 out]
              }
              frame "SMU" {
                n780 = Unbundle By Name(w1391) -> ("Field_M"=w1390:refnum<queue>)
                n781 = Bundle By Name(cluster=T53 {"Command"=enum."Connect", "Data"=variant} ("MSG to Source meter"), "Data"="USB0::0x05E6::0x2450::04405250::INSTR") -> (w1387:T53)
                n782 = call "Put in mailbox.vi"("Message"=w1387, "Queue in"=w1390) -> ()  [unwired: 7 in, 3 out]
              }
              frame "THz" {
                n783 = disable-structure shown="Disabled" {
                  disable-tunnel: [T57[] [{"Lower limit [GHz]"=8.0, "Upper limit [GHz]"=20.0, "Device name"="VDIS0122", "Connection"="", "Description"="VDI Synth", "Connected"=FALSE, "Last settings"="", "Operation mode"=enum."Disabled", "Enable ch 1"=FALSE, "Enable ch 2"=FALSE}, {"Lower limit [GHz]"=8.0, "Upper limit [GHz]"=20.0, "Device name"="VDIYT7", "Connection"="", "Description"="VDI Tracking", "Connected"=FALSE, "Last settings"="", "Operation mode"=enum."Disabled", "Enable ch 1"=FALSE, "Enable ch 2"=FALSE}] ("Array") w1400] -> w1392
                  frame Disabled {
                  }
                  frame Enabled {
                    n784 = Bundle By Name(cluster=T57 {"Lower limit [GHz]"=0.0, "Upper limit [GHz]"=0.0, "Device name"="", "Connection"="", "Description"="", "Connected"=FALSE, "Last settings"="", "Operation mode"=enum."Disabled", "Enable ch 1"=FALSE, "Enable ch 2"=FALSE} ("Configuration"), "Connection"="USB0::0x03EB::0xAFFF::848-0B4424003-0065::INSTR") -> (w1401:T57)
                    n785 = Build Array(w1401) -> (w1400:T57[])
                  }
                }
                n786 = Unbundle By Name(w1397) -> ("MW_C"=w1394:refnum<queue>)
                n787 = Bundle By Name(cluster=T45 {"Command"=enum."Connect", "Data"=variant} ("Incoming msg"), "Data"=w1392) -> (w1396:T45)
                n788 = call "Put in mailbox.vi"("Priority? (F)"=TRUE, "Message"=w1396, "Queue in"=w1394) -> ()  [unwired: 6 in, 3 out]
              }
              frame "VTI" {
                n789 = Unbundle By Name(w1408) -> ("Tmp_C"=w1407:refnum<queue>)
                n790 = Bundle By Name(cluster=T52 {"Command"=enum."Initialize", "Data"=variant} ("MSG for VTI"), "Command"=TC_commands."Initialize", "Data"="COM4") -> (w1406:T52)
                n791 = call "Put in mailbox.vi"("Message"=w1406, "Queue in"=w1407) -> ()  [unwired: 7 in, 3 out]
              }
            }
          }
        }
        "Actual measurement" <- w114
        "Logger" <- w113
        n792 = Index Array(array=w113) -> (element=w118:string)  [unwired: 1 in]
        n793 = Bundle By Name(cluster=w117, "Last log"=w118) -> (w115:T24)
        n794 = local write "Infobar"(w115) -> ()
      }
      frame "Check message" {
        n795 = Unbundle By Name(w1415) -> ("TOP"=w1432:refnum<queue>)
        n796 = call "Receive message by TOP.vi"("timeout (100)"=10 ("timeout in ms (-1)"), "Mailbox in"=w1432) -> ("error out"=w1425:errorcluster, "timed out?"=w1427:bool, "Unread"=w1424:i32, "MSG packet"=w1431:T81)  [unwired: 6 in]
        n797 = Or(x=w1427, y=w1425) -> (x .or. y?=w1426:bool)
        n798 = local read "Busy"() -> (w1421:bool)
        n799 = Unbundle By Name(w1412) -> ("Experiment state"=w1411:T25)
        n800 = Not(x=w1421) -> (.not. x?=w1419:bool)
        n801 = Greater?(x=w1424, y=2) -> (0:w1422:bool)
        n802 = And(x=w1422, y=w1419) -> (x .and. y?=w1420:bool)
        n803 = case shown="False" w1426 {
          tunnel: w1431 -> [w1454 _]
          tunnel: w1429 -> [w1451 w2921]
          tunnel: [w1450 w2921] -> w1428
          tunnel: w1412 -> [w1445 w2920]
          tunnel: [w1444 w2920] -> w1417
          tunnel: w1416 -> [w1447 _]
          tunnel: w1415 -> [w1446 _]
          tunnel: w1414 -> [w1443 w2919]
          tunnel: [w1442 w2919] -> w1413
          frame False {
            n804 = Unbundle By Name(w1454) -> ("Time"=w1449:timestamp, "Module"=w1453:T82, "Response"=w1452:string, "Data"=w1448:variant)
            n805 = case "Message from module:" shown="\"Rotator\"" w1453 {
              selector: w1453 -> [_ _ _ _ _ _ _ _ _ _ w2666 w2915]
              tunnel: w1452 -> [w1465 w1781 w1917 w1932 w1947 w1965 w1988 w2122 w2264 w2391 w2670 w2913]
              tunnel: w1448 -> [w1464 w1778 w1914 w1929 w1944 w1962 w1985 w2121 w2263 w2394 w2669 _]
              tunnel: w1451 -> [w1463 w1780 w1916 w1931 w1946 w1964 w1987 w2118 w2262 w2393 w2668 w2918]
              tunnel: [w1462 w1779 w1915 w1930 w1945 w1963 w1986 w2117 w2261 w2392 w2667 w2917] -> w1450
              tunnel: w1449 -> [w1461 w1777 w1913 w1928 w1943 w1961 w1984 w2120 w2256 w2385 w2659 _]
              tunnel: w1445 -> [w1460 w1775 w1911 w1926 w1941 w1959 w1982 w2119 w2254 w2390 w2665 w2911]
              tunnel: [w1459 w1776 w1912 w1927 w1942 w1960 w1983 w2119 w2260 w2390 w2665 w2911] -> w1444
              tunnel: w1447 -> [_ _ w1910 w1925 w1940 w1958 w1981 _ _ _ _ _]
              tunnel: w1446 -> [_ _ _ _ _ _ _ w2112 _ _ _ _]
              tunnel: w1443 -> [w1458 w1774 w1909 w1924 w1939 w1957 w1980 w2113 w2259 w2389 w2663 w2910]
              tunnel: [w1456 w1772 w1907 w1922 w1937 w1955 w1978 w2114 w2258 w2388 w2661 w2910] -> w1442
              frame "Magnet" {
                # "list of responses:"
                n806 = Unbundle By Name(w1458) -> ("Magnet"=w1457:T83)
                n807 = case shown="\"Update\"" w1465 {
                  selector: w1465 -> [w1472 _ _ _ _ _ _ _ _ _ _ w1669 _ _ _ _]
                  tunnel: w1464 -> [w1468 w1515 w1529 w1540 w1564 w1593 w1603 w1618 w1631 w1641 w1656 w1673 w1706 w1744 _ _]
                  tunnel: w1463 -> [w1470 w1512 w1522 w1536 w1548 w1585 w1598 w1616 w1629 w1638 w1653 w1666 w1689 w1745 w1749 w1761]
                  tunnel: [w1471 w1495 w1523 w1535 w1547 w1584 w1599 w1617 w1630 w1639 w1654 w1665 w1690 w1745 w1748 w1760] -> w1462
                  tunnel: w1461 -> [_ _ _ _ w1551 _ _ _ _ _ _ _ w1681 w1740 _ _]
                  tunnel: w1460 -> [w1467 w1500 w1521 w1532 w1554 w1581 w1597 w1615 w1628 w1637 w1652 w1664 w1675 w1741 w1751 w1763]
                  tunnel: [w1467 w1500 w1521 w1532 w1553 w1581 w1597 w1615 w1628 w1637 w1652 w1664 w1687 w1741 w1751 w1763] -> w1459
                  tunnel: w1457 -> [w1466 w1499 w1520 w1530 w1552 w1580 w1596 w1614 w1627 w1636 w1651 w1663 w1685 w1730 w1747 w1759]
                  tunnel: [w1466 w1494 w1519 w1530 w1550 w1580 w1596 w1614 w1627 w1636 w1651 w1662 w1680 w1730 w1747 w1759] -> w1455
                  frame "ignore", Default {
                    n808 = Match Pattern(string=w1472, regular expression="Error") -> (after substring=w1469:string, offset past match=w1474:i32)  [unwired: 1 in, 2 out]
                    n809 = Greater Or Equal To 0?(x=w1474) -> (x >= 0?=w1473:bool)
                    n810 = case shown="True" w1473 {
                      tunnel: w1470 -> [w1478 w1488]
                      tunnel: w1472 -> [w1477 w1487]
                      tunnel: [w1476 w1489] -> w1471
                      tunnel: w1469 -> [_ _]
                      tunnel: w1468 -> [_ w1485]
                      frame False {
                        n811 = call "simple Shift string array.vi"("Element in"=w1477, "Array in"=w1478) -> ("Array out"=w1476:string[])  [unwired: 8 in, 1 out]
                      }
                      frame True {
                        n812 = Variant To Data(type=errorcluster {"status"=FALSE, "code"=0, "source"=""} ("error constant"), Variant=w1485) -> (data=w1483:errorcluster)  [unwired: 1 in, 1 out]
                        n813 = Unbundle By Name(w1483) -> ("source"=w1482:string)
                        n814 = call <vilib>:"Space Constant.vi"() -> ("String"=w1486:string)
                        n815 = Concatenate Strings("Magnet: " ("string"), w1487, w1486, w1482) -> (w1480:string)
                        n816 = local read "loggersRef"() -> (w1481:refnum<file>)
                        n817 = call "Write in logger.vi"("String in"=w1480, "logger refnum"=w1481) -> ()  [unwired: 2 in, 2 out]
                        n818 = call "simple Shift string array.vi"("Element in"=w1480, "Array in"=w1488) -> ("Array out"=w1489:string[])  [unwired: 8 in, 1 out]
                      }
                    }
                  }
                  frame "Connect" {
                    w1507 = TRUE ("PSU")
                    w1506 = T33."Enabled" ("Disabled")
                    n819 = Variant To Data(type="", Variant=w1515) -> (data=w1491:string)  [unwired: 1 in, 1 out]
                    n820 = local read "Instr status"() -> (w1510:T1)
                    n821 = Bundle By Name(cluster=w1510, "Mag"=w1507) -> (w1514:T1)
                    n822 = Unbundle By Name(w1510) -> ("THz"=w1509:bool, "MFLI"=w1508:bool)
                    n823 = local write "Instr status"(w1514) -> ()
                    n824 = control-ref of="Magnet controls"() -> (w1511:refnum<vi>)
                    n825 = Compound Arithmetic op=AND(w1509, w1508, w1507) -> (w1505:bool)
                    n826 = call "Add actual date time to string.vi"("String in"="Magnet module initialized") -> ("String out"=w1503:string)  [unwired: 4 in]
                    n827 = Select(t=w1506, s=w1505, f=T33."Disabled and Grayed Out" ("Disabled")) -> (s? t:f=w1501:T33)
                    n828 = local read "loggersRef"() -> (w1502:refnum<file>)
                    n829 = property class="Clust (strict)"(reference=w1511, "DisabledEnum"=w1506) -> ()  [unwired: 1 in, 2 out]
                    n830 = Concatenate Strings(w1503, "\r\n", w1491) -> (w1493:string)
                    n831 = call "simple Shift string array.vi"("Element in"=w1503, "Array in"=w1512) -> ("Array out"=w1496:string[])  [unwired: 8 in, 1 out]
                    n832 = call "Write in logger.vi"("String in"=w1493, "logger refnum"=w1502) -> ()  [unwired: 2 in, 2 out]
                    n833 = call "Add actual date time to string.vi"("String in"=w1491) -> ("String out"=w1497:string)  [unwired: 4 in]
                    n834 = call "simple Shift string array.vi"("Element in"=w1497, "Array in"=w1496) -> ("Array out"=w1495:string[])  [unwired: 8 in, 1 out]
                    n835 = property on="Run script btn" class="Bool (strict)"("DisabledEnum"=w1501) -> ()  [unwired: 2 in, 2 out]
                    n836 = Bundle By Name(cluster=w1499, "PSU"="SMS120" ("regular expression")) -> (w1494:T83)
                  }
                  frame "TM revision" {
                    n837 = Variant To Data(type=T58 {"Instr Serial Number"="", "Instr Driver Revision"="", "Instr Firmware Revision"="", "Instr Model Number"=""} ("TM Revision"), Variant=w1529) -> (data=w1527:T58)  [unwired: 1 in, 1 out]
                    n838 = Unbundle By Name(w1527) -> ("Instr Model Number"=w1518:string)
                    n839 = call <vilib>:"Space Constant.vi"() -> ("String"=w1525:string)
                    n840 = Concatenate Strings("Temperature monitor:" ("string"), w1525, w1518) -> (w1524:string)
                    n841 = Bundle By Name(cluster=w1520, "T monitor"=w1518) -> (w1519:T83)
                    n842 = call "Add actual date time to string.vi"("String in"=w1524) -> ("String out"=w1516:string)  [unwired: 4 in]
                    n843 = local read "loggersRef"() -> (w1517:refnum<file>)
                    n844 = call "simple Shift string array.vi"("Element in"=w1516, "Array in"=w1522) -> ("Array out"=w1523:string[])  [unwired: 8 in, 1 out]
                    n845 = call "Write in logger.vi"("String in"=w1516, "logger refnum"=w1517) -> ()  [unwired: 2 in, 2 out]
                  }
                  frame "Initialization error" {
                    n846 = Variant To Data(type=errorcluster {"status"=FALSE, "code"=0, "source"=""} ("error constant"), Variant=w1540) -> (data=w1538:errorcluster, error out=w1531:errorcluster)  [unwired: 1 in]
                    n847 = Unbundle By Name(w1538) -> ("source"=w1537:string)
                    n848 = call "Add actual date time to string.vi"("String in"=w1537) -> ("String out"=w1534:string)  [unwired: 4 in]
                    n849 = call "simple Shift string array.vi"("Element in"=w1534, "Array in"=w1536) -> ("Array out"=w1535:string[])  [unwired: 8 in, 1 out]
                    n850 = local read "loggersRef"() -> (w1533:refnum<file>)
                    n851 = call "Write in logger.vi"("error in"=w1531, "String in"=w1534, "logger refnum"=w1533) -> ()  [unwired: 1 in, 2 out]
                  }
                  frame "Update" {
                    n852 = Variant To Data(type=T59 {"Desired"={"Field [T]"=0.0, "Ramp [T/s]"=0.0, "Custom Ramp?"=TRUE, "Mode"=enum."Persistant"}, "Actual"={"Mode"=enum."Persistant", "Ramping output"=enum."At Target", "Ready for change"=FALSE, "Switch heater"=FALSE, "Cooler Overheat"=FALSE, "Coil overheat"=FALSE, "Energized"=FALSE, "Output [T]"=0.0, "Field [T]"=0.0, "Ramp[T/s]"=0.0, "Switch\ntemperature [K]"=1.0, "Voltage [V]"=0.0, "Current direction"=FALSE}} ("output cluster"), Variant=w1564) -> (data=w1546:T59)  [unwired: 1 in, 1 out]
                    n853 = Unbundle By Name(w1546) -> ("Actual.Ready for change"=w1544:bool, "Actual.Mode"=w1545:T61, "Actual.Field [T]"=w1542:dbl)
                    n854 = local read "Instr status"() -> (w1562:T1)
                    n855 = local read "Magnet controls"() -> (w1557:T23)
                    n856 = Bundle By Name(cluster=w1562, "Mag"=TRUE ("PSU")) -> (w1561:T1)
                    n857 = Bundle By Name(cluster=w1554, "Field [T]"=w1542) -> (w1553:T24)
                    n858 = local write "Instr status"(w1561) -> ()
                    n859 = call "Magnet update rewiring.vi"("output cluster"=w1546, "Time"=w1551, "Magnet in"=w1552, "Magnet controls in"=w1557) -> ("Magnet out"=w1550:T83, "Magnet controls out"=w1556:T23)  [unwired: 6 in]
                    n860 = Greater?(x=w1542, y=0.01) -> (0:→"Magnetic\nfield state":bool)
                    n861 = local write "Magnet controls"(w1556) -> ()
                    n862 = case shown="\"Quenched\"" w1545 {
                      selector: w1545 -> [_ _ _ w1573]
                      tunnel: [w1566 w1567 w1570 w1575] -> w1547
                      tunnel: w1548 -> [w1566 w1567 w1570 w1574]
                      tunnel: [T33."Enabled" ("Disabled") T33."Disabled and Grayed Out" ("f") T33."Disabled and Grayed Out" ("f") T33."Disabled and Grayed Out" ("f")] -> w1549
                      frame "Persistant", Default {
                      }
                      frame "Switching" {
                      }
                      frame "Ramping" {
                      }
                      frame "Quenched" {
                        n863 = Format Into String(w1573) -> (resulting string=w1572:string)  [unwired: 3 in, 1 out]
                        n864 = call "Add actual date time to string.vi"("String in"=w1572) -> ("String out"=w1576:string)  [unwired: 4 in]
                        n865 = local read "loggersRef"() -> (w1577:refnum<file>)
                        n866 = call "simple Shift string array.vi"("Element in"=w1576, "Array in"=w1574) -> ("Array out"=w1575:string[])  [unwired: 8 in, 1 out]
                        n867 = call "Write in logger.vi"("String in"=w1576, "logger refnum"=w1577) -> ()  [unwired: 2 in, 2 out]
                      }
                    }
                    n868 = Select(t=T33."Enabled" ("Disabled"), s=w1544, f=T33."Disabled and Grayed Out") -> (s? t:f=w1555:T33)
                    n869 = property on="Mode switch" class="Bool (strict)"("DisabledEnum"=w1555) -> ()  [unwired: 2 in, 2 out]
                    n870 = property on="Equalize" class="Bool (strict)"("DisabledEnum"=w1549) -> ()  [unwired: 2 in, 2 out]
                    n871 = property on="Discharge" class="Bool (strict)"("DisabledEnum"=w1549) -> ()  [unwired: 2 in, 2 out]
                  }
                  frame "Update error" {
                    # "ReInitialize Magnet?"
                    n872 = Variant To Data(type=errorcluster {"status"=FALSE, "code"=0, "source"=""} ("error in (no error)"), Variant=w1593) -> (data=w1591:errorcluster)  [unwired: 1 in, 1 out]
                    n873 = Unbundle By Name(w1591) -> ("source"=w1588:string)
                    n874 = local read "Instr status"() -> (w1587:T1)
                    n875 = Bundle By Name(cluster=w1587, "Mag"=FALSE ("PSU")) -> (w1586:T1)
                    n876 = local write "Instr status"(w1586) -> ()
                    n877 = Concatenate Strings("Magnet Update error: " ("String in"), w1588) -> (w1589:string)
                    n878 = property on="Magnet controls" class="Clust (strict)"("DisabledEnum"=T33."Disabled and Grayed Out" ("Disabled")) -> ()  [unwired: 2 in, 2 out]
                    n879 = local read "loggersRef"() -> (w1579:refnum<file>)
                    n880 = call "Add actual date time to string.vi"("String in"=w1589) -> ("String out"=w1578:string)  [unwired: 4 in]
                    n881 = call "Write in logger.vi"("String in"=w1578, "logger refnum"=w1579) -> ()  [unwired: 2 in, 2 out]
                    n882 = call "simple Shift string array.vi"("Element in"=w1578, "Array in"=w1585) -> ("Array out"=w1584:string[])  [unwired: 8 in, 1 out]
                  }
                  frame "Switch mode acepted" {
                    n883 = Variant To Data(type=Magnet_mode_public."Ramping" ("Operation mode"), Variant=w1603) -> (data=w1601:T34)  [unwired: 1 in, 1 out]
                    n884 = case shown="\"Ramping\", Default" w1601 {
                      tunnel: ["Switching to ramping mode" "Switching to perzistant mode"] -> w1600
                      frame "Ramping", Default {
                      }
                      frame "Persistant" {
                      }
                    }
                    n885 = call "Add actual date time to string.vi"("String in"=w1600) -> ("String out"=w1594:string)  [unwired: 4 in]
                    n886 = local read "loggersRef"() -> (w1595:refnum<file>)
                    n887 = call "simple Shift string array.vi"("Element in"=w1594, "Array in"=w1598) -> ("Array out"=w1599:string[])  [unwired: 8 in, 1 out]
                    n888 = call "Write in logger.vi"("String in"=w1594, "logger refnum"=w1595) -> ()  [unwired: 2 in, 2 out]
                  }
                  frame "Equalize output" {
                    n889 = Variant To Data(type=T35 {"Field [T]"=0.0, "Ramp [T/s]"=0.0, "Custom Ramp?"=TRUE, "Mode"=enum."Persistant"} ("Desired"), Variant=w1618) -> (data=w1610:T35)  [unwired: 1 in, 1 out]
                    n890 = Unbundle By Name(w1610) -> ("Field [T]"=w1606:dbl, "Ramp [T/s]"=w1609:dbl)
                    n891 = Equal To 0?(x=w1609) -> (x = 0?=w1608:bool)
                    n892 = case shown="False" w1608 {
                      tunnel: [w1619 "Output equalization command ignored"] -> w1607
                      tunnel: w1606 -> [w1621 _]
                      frame False {
                        n893 = Format Into String(format string="Output equalized to %f T ", w1621) -> (resulting string=w1619:string)  [unwired: 2 in, 1 out]
                      }
                      frame True {
                      }
                    }
                    n894 = call "Add actual date time to string.vi"("String in"=w1607) -> ("String out"=w1612:string)  [unwired: 4 in]
                    n895 = local read "loggersRef"() -> (w1613:refnum<file>)
                    n896 = call "simple Shift string array.vi"("Element in"=w1612, "Array in"=w1616) -> ("Array out"=w1617:string[])  [unwired: 8 in, 1 out]
                    n897 = call "Write in logger.vi"("String in"=w1612, "logger refnum"=w1613) -> ()  [unwired: 2 in, 2 out]
                  }
                  frame "Stop ramping" {
                    n898 = Variant To Data(type="" ("Desired"), Variant=w1631) -> (data=w1623:string)  [unwired: 1 in, 1 out]
                    n899 = call "Add actual date time to string.vi"("String in"=w1623) -> ("String out"=w1625:string)  [unwired: 4 in]
                    n900 = local read "loggersRef"() -> (w1626:refnum<file>)
                    n901 = call "simple Shift string array.vi"("Element in"=w1625, "Array in"=w1629) -> ("Array out"=w1630:string[])  [unwired: 8 in, 1 out]
                    n902 = call "Write in logger.vi"("String in"=w1625, "logger refnum"=w1626) -> ()  [unwired: 2 in, 2 out]
                  }
                  frame "Flip polarity" {
                    n903 = Variant To Data(type="" ("Operation mode"), Variant=w1641) -> (data=w1633:string, error out=w1632:errorcluster)  [unwired: 1 in]
                    n904 = call "Add actual date time to string.vi"("String in"=w1633) -> ("String out"=w1634:string)  [unwired: 4 in]
                    n905 = local read "loggersRef"() -> (w1635:refnum<file>)
                    n906 = call "simple Shift string array.vi"("Element in"=w1634, "Array in"=w1638) -> ("Array out"=w1639:string[])  [unwired: 8 in, 1 out]
                    n907 = call "Write in logger.vi"("error in"=w1632, "String in"=w1634, "logger refnum"=w1635) -> ()  [unwired: 1 in, 2 out]
                  }
                  frame "Zero output" {
                    n908 = Variant To Data(type=TRUE, Variant=w1656) -> (data=w1647:bool, error out=w1648:errorcluster)  [unwired: 1 in]
                    n909 = Select(t="confirmed", s=w1647, f="denied") -> (s? t:f=w1644:string)
                    n910 = Concatenate Strings("Zero output ", w1644) -> (w1642:string)
                    n911 = call "Add actual date time to string.vi"("String in"=w1642) -> ("String out"=w1649:string)  [unwired: 4 in]
                    n912 = local read "loggersRef"() -> (w1650:refnum<file>)
                    n913 = call "simple Shift string array.vi"("Element in"=w1649, "Array in"=w1653) -> ("Array out"=w1654:string[])  [unwired: 8 in, 1 out]
                    n914 = call "Write in logger.vi"("error in"=w1648, "String in"=w1649, "logger refnum"=w1650) -> ()  [unwired: 1 in, 2 out]
                  }
                  frame "Ramping" {
                    n915 = Variant To Data(type=T35 {"Field [T]"=0.0, "Ramp [T/s]"=0.0, "Custom Ramp?"=TRUE, "Mode"=enum."Persistant"} ("Set Field"), Variant=w1673) -> (data=w1671:T35)  [unwired: 1 in, 1 out]
                    n916 = Unbundle By Name(w1671) -> ("Field [T]"=w1668:dbl, "Ramp [T/s]"=w1660:dbl)
                    n917 = Multiply(x=w1660, y=1000.0) -> (x*y=w1659:dbl)
                    n918 = Bundle By Name(cluster=w1663, "Ramp [mT/s]"=w1659) -> (w1662:T83)
                    n919 = Format Into String(format string=" B= %f [T] Ramp= %f [mT/s]", initial string=w1669, w1668, w1659) -> (resulting string=w1667:string)  [unwired: 1 in, 1 out]
                    n920 = call "Add actual date time to string.vi"("String in"=w1667) -> ("String out"=w1657:string)  [unwired: 4 in]
                    n921 = local read "loggersRef"() -> (w1658:refnum<file>)
                    n922 = call "simple Shift string array.vi"("Element in"=w1657, "Array in"=w1666) -> ("Array out"=w1665:string[])  [unwired: 8 in, 1 out]
                    n923 = call "Write in logger.vi"("String in"=w1657, "logger refnum"=w1658) -> ()  [unwired: 2 in, 2 out]
                  }
                  frame "Set field" {
                    n924 = Unbundle By Name(w1675) -> ("Experiment state"=w1688:T25)
                    n925 = local read "Magnet controls"() -> (w1704:T23)
                    n926 = Variant To Data(type=T35 {"Field [T]"=0.0, "Ramp [T/s]"=0.0, "Custom Ramp?"=TRUE, "Mode"=enum."Persistant"} ("Set Field"), Variant=w1706) -> (data=w1703:T35, error out=w1676:errorcluster)  [unwired: 1 in]
                    n927 = Unbundle By Name(w1685) -> ("Field [T]"=w1692:dbl)
                    n928 = case shown="\"Begin\"" w1688 {
                      selector: w1688 -> [w1708 _]
                      tunnel: [w1708 experiment_state."Acquisition" ("Value")] -> w1686
                      tunnel: w1681 -> [_ w1711]
                      tunnel: w1675 -> [w1707 w1709]
                      tunnel: [w1707 w1710] -> w1674
                      frame "Setup", Default {
                      }
                      frame "Begin" {
                        n929 = Bundle By Name(cluster=w1709, "Started"=w1711) -> (w1710:T24)
                      }
                    }
                    n930 = Unbundle By Name(w1703) -> ("Field [T]"=w1697:dbl, "Ramp [T/s]"=w1684:dbl, "Custom Ramp?"=w1702:bool)
                    n931 = Unbundle By Name(w1704) -> ("Desired ramp\nrate [mT/s]"=w1701:dbl)
                    n932 = Not(x=w1702) -> (.not. x?=w1700:bool)
                    n933 = call <userlib>:"MGI Approximately Equal.vi"("Numeric 2"=w1701, "Numeric 1"=w1684) -> ("approx = ?"=w1699:bool)
                    n934 = Multiply(x=w1684, y=1000.0 ("x")) -> (x*y=w1682:dbl)
                    n935 = Or(x=w1700, y=w1699) -> (x .or. y?=w1696:bool)
                    n936 = Bundle By Name(cluster=w1674, "Experiment state"=w1686) -> (w1687:T24)
                    n937 = case shown="False" w1696 {
                      tunnel: ["Warning: Custom ramp was adjusted" ""] -> w1694
                      frame False {
                      }
                      frame True {
                      }
                    }
                    n938 = Format Into String(format string="Setting magnetic field from %f [T ] to %f [T] with ramp %f [mT/s]", error in=w1676, w1692, w1697, w1682) -> (resulting string=w1695:string, error out=w1677:errorcluster)  [unwired: 1 in]
                    n939 = Concatenate Strings(w1695, "\r", w1694) -> (w1678:string)
                    n940 = call "Add actual date time to string.vi"("String in"=w1678) -> ("String out"=w1691:string)  [unwired: 4 in]
                    n941 = local read "loggersRef"() -> (w1679:refnum<file>)
                    n942 = Bundle By Name(cluster=w1685, "Last update"=w1681, "Ramp [mT/s]"=w1682) -> (w1680:T83)
                    n943 = call "simple Shift string array.vi"("Element in"=w1691, "Array in"=w1689) -> ("Array out"=w1690:string[])  [unwired: 8 in, 1 out]
                    n944 = call "Write in logger.vi"("error in"=w1677, "String in"=w1678, "logger refnum"=w1679) -> ()  [unwired: 1 in, 2 out]
                  }
                  frame "Temperatures" {
                    n945 = local read "Temperature monitor"() -> (w1727:T12)
                    n946 = Variant To Data(type=T62 {"First stage A [K]"=0.0, "Second stage A [K]"=0.0, "Firs stage B [K]"=0.0, "Second stage B [K]"=0.0, "Inner magnet [K]"=0.0, "Outer Magnet [K]"=0.0, "Switch [K]"=0.0, "Support plate [K]"=0.0, "Time stamp"=0.0} ("LSC218 sensors"), Variant=w1744) -> (data=w1734:T62)  [unwired: 1 in, 1 out]
                    n947 = local read "Drift[K/s]"() -> (w1728:dbl[])
                    n948 = property on="VTI" class="Clust (strict)"() -> ("Value"=w1739:T84)  [unwired: 2 in, 2 out]
                    n949 = Cluster To Array(cluster=w1734) -> (array=w1724:dbl[])
                    n950 = Unbundle By Name(w1730) -> ("Field [T]"=w1729:dbl)
                    n951 = local read "Temperature log ref"() -> (w1742:refnum<file>)
                    n952 = Cluster To Array(cluster=w1727) -> (array=w1726:dbl[])
                    n953 = Unbundle By Name(w1739) -> ("VTI [K]"=w1732:dbl, "Sample [K]"=w1731:dbl, "Trap[K]"=w1738:dbl, "HePot [K]"=w1737:dbl)
                    n954 = Array Subset(array=w1724, length=8) -> (w1716:dbl[])  [unwired: 1 in]
                    n955 = Array Subset(array=w1726, length=8) -> (w1721:dbl[])  [unwired: 1 in]
                    n956 = Subtract(x=w1716, y=w1721) -> (x-y=w1723:dbl[])
                    n957 = Divide(x=w1723, y=2.5) -> (x/y=w1720:dbl[])
                    n958 = call "Bundle temperatures.vi"("Sample"=w1731, "VTI space"=w1732, "LSC218 sensors"=w1734) -> ("Tmp [K]"=→"Tmp [K]":T3)  [unwired: 8 in]
                    n959 = Build Array (concatenate)(w1716, w1732, w1731, w1738, w1737) -> (w1736:dbl[])
                    n960 = call "Log temperatures.vi"("LSC218 sensors"=w1734, "Time"=w1740, "Tmp logfile in"=w1742, "VTI"=w1732, "Sample"=w1731, "Trap"=w1738, "HePot"=w1737, "Field [T]"=w1729, "Logging interval (10s)"=10.0 ("Logging interval (20s)")) -> ("Tmp logfile ref"=w1717:refnum<file>)  [unwired: 4 in, 2 out]
                    n961 = Replace Array Subset(array=w1728, new element=w1720) -> (→"Drift[K/s]":dbl[])  [unwired: 1 in]
                    n962 = Array To Cluster(array=w1736) -> (cluster=w1735:T12)
                    n963 = local write "Temperature log ref"(w1717) -> ()
                    n964 = flat-sequence {
                      tunnel: w1735 -> [w1746]
                      tunnel: w1721 -> [_]
                      frame #0 {
                        "Temperature monitor" <- w1746
                      }
                    }
                  }
                  frame "End" {
                    n965 = local read "loggersRef"() -> (w1753:refnum<file>)
                    n966 = local read "Instr status"() -> (w1757:T1)
                    n967 = call "Add actual date time to string.vi"("String in"="Magnet ended") -> ("String out"=w1750:string)  [unwired: 4 in]
                    n968 = Bundle By Name(cluster=w1757, "Mag"=FALSE ("PSU")) -> (w1758:T1)
                    n969 = call "Write in logger.vi"("String in"=w1750, "logger refnum"=w1753) -> ()  [unwired: 2 in, 2 out]
                    n970 = local write "Instr status"(w1758) -> ()
                    n971 = control-ref of="Magnet controls"() -> (w1755:refnum<vi>)
                    n972 = call "simple Shift string array.vi"("Element in"=w1750, "Array in"=w1749) -> ("Array out"=w1748:string[])  [unwired: 8 in, 1 out]
                    n973 = property class="Clust (strict)"(reference=w1755, "DisabledEnum"=T33."Disabled and Grayed Out" ("Disabled")) -> ()  [unwired: 1 in, 2 out]
                  }
                  frame "Disconnect" {
                    n974 = local read "loggersRef"() -> (w1765:refnum<file>)
                    n975 = local read "Instr status"() -> (w1769:T1)
                    n976 = call "Add actual date time to string.vi"("String in"="Magnet dissconnected") -> ("String out"=w1762:string)  [unwired: 4 in]
                    n977 = Bundle By Name(cluster=w1769, "Mag"=FALSE ("PSU")) -> (w1770:T1)
                    n978 = call "Write in logger.vi"("String in"=w1762, "logger refnum"=w1765) -> ()  [unwired: 2 in, 2 out]
                    n979 = local write "Instr status"(w1770) -> ()
                    n980 = call "simple Shift string array.vi"("Element in"=w1762, "Array in"=w1761) -> ("Array out"=w1760:string[])  [unwired: 8 in, 1 out]
                    n981 = control-ref of="Magnet controls"() -> (w1767:refnum<vi>)
                    n982 = property class="Clust (strict)"(reference=w1767, "DisabledEnum"=T33."Disabled and Grayed Out" ("Disabled")) -> ()  [unwired: 1 in, 2 out]
                  }
                }
                n983 = Bundle By Name(cluster=w1458, "Magnet"=w1455) -> (w1456:T8)
              }
              frame "Excitation" {
                n984 = Unbundle By Name(w1774) -> ("THz"=w1773:T85)
                n985 = case shown="\"Disconnect\"" w1781 {
                  selector: w1781 -> [w1784 _ _ _ _ _]
                  tunnel: w1780 -> [w1783 w1839 w1842 w1872 w1878 w1894]
                  tunnel: [w1782 w1838 w1842 w1873 w1879 w1895] -> w1779
                  tunnel: w1778 -> [w1785 w1830 _ w1871 w1880 w1896]
                  tunnel: w1777 -> [_ w1810 _ w1848 w1882 w1898]
                  tunnel: w1775 -> [w1790 w1829 w1841 w1844 w1886 w1902]
                  tunnel: [w1790 w1829 w1841 w1860 w1886 w1902] -> w1776
                  tunnel: w1773 -> [w1789 w1824 w1840 w1850 w1885 w1901]
                  tunnel: [w1789 w1823 w1840 w1849 w1884 w1900] -> w1771
                  frame "Ignore", Default {
                    n986 = Match Pattern(string=w1784, regular expression="Error") -> (offset past match=w1788:i32)  [unwired: 1 in, 3 out]
                    n987 = Greater Or Equal To 0?(x=w1788) -> (x >= 0?=w1786:bool)
                    n988 = case shown="False" w1786 {
                      tunnel: w1783 -> [w1793 w1803]
                      tunnel: w1784 -> [w1792 w1802]
                      tunnel: [w1791 w1804] -> w1782
                      tunnel: w1785 -> [_ w1800]
                      frame False {
                        n989 = call "simple Shift string array.vi"("Element in"=w1792, "Array in"=w1793) -> ("Array out"=w1791:string[])  [unwired: 8 in, 1 out]
                      }
                      frame True {
                        n990 = Variant To Data(type=errorcluster {"status"=FALSE, "code"=0, "source"=""} ("error constant"), Variant=w1800) -> (data=w1798:errorcluster)  [unwired: 1 in, 1 out]
                        n991 = Unbundle By Name(w1798) -> ("source"=w1797:string)
                        n992 = call <vilib>:"Space Constant.vi"() -> ("String"=w1801:string)
                        n993 = Concatenate Strings("THz: " ("string"), w1802, w1801, w1797) -> (w1795:string)
                        n994 = local read "loggersRef"() -> (w1796:refnum<file>)
                        n995 = call "Write in logger.vi"("String in"=w1795, "logger refnum"=w1796) -> ()  [unwired: 2 in, 2 out]
                        n996 = call "simple Shift string array.vi"("Element in"=w1795, "Array in"=w1803) -> ("Array out"=w1804:string[])  [unwired: 8 in, 1 out]
                      }
                    }
                  }
                  frame "Connect", "Initialize" {
                    w1807 = T33."Disabled and Grayed Out" ("f")
                    w1808 = T33."Enabled" ("Disabled")
                    n997 = Variant To Data(type="", Variant=w1830) -> (data=w1828:string, error out=w1822:errorcluster)  [unwired: 1 in]
                    n998 = call <vilib>:"Trim Whitespace.vi"("string"=w1828) -> ("trimmed string"=w1819:string)  [unwired: 1 in]
                    n999 = Concatenate Strings("Initializing..." ("string"), w1828) -> (w1812:string)
                    n1000 = Match Pattern(string=w1819, regular expression="Device:") -> (after substring=w1820:string)  [unwired: 1 in, 3 out]
                    n1001 = Match Pattern(string=w1820, regular expression="Description:") -> (before substring=w1817:string, after substring=w1816:string)  [unwired: 1 in, 2 out]
                    n1002 = Match Pattern(string=w1816, regular expression="Connection:") -> (before substring=w1814:string, offset past match=w1813:i32)  [unwired: 1 in, 2 out]
                    n1003 = Greater Or Equal To 0?(x=w1813) -> (x >= 0?=w1806:bool)
                    n1004 = local read "Instr status"() -> (w1835:T1)
                    n1005 = Bundle By Name(cluster=w1824, "Name"=w1817, "Description"=w1814, "Last update"=w1810) -> (w1823:T85)
                    n1006 = Bundle By Name(cluster=w1835, "THz"=w1806) -> (w1836:T1)
                    n1007 = local write "Instr status"(w1836) -> ()
                    n1008 = Unbundle By Name(w1835) -> ("Mag"=w1834:bool, "MFLI"=w1833:bool)
                    n1009 = local read "loggersRef"() -> (w1831:refnum<file>)
                    n1010 = Compound Arithmetic op=AND(w1806, w1834, w1833) -> (w1832:bool)
                    n1011 = call "Add actual date time to string.vi"("String in"=w1812) -> ("String out"=w1827:string)  [unwired: 4 in]
                    n1012 = Select(t=w1808, s=w1832, f=w1807) -> (s? t:f=w1809:T33)
                    n1013 = Select(t=w1808, s=w1806, f=w1807) -> (s? t:f=w1805:T33)
                    n1014 = property on="Run script btn" class="Bool (strict)"(error in=w1822, "DisabledEnum"=w1809) -> (error out=w1826:errorcluster)  [unwired: 1 in, 1 out]
                    n1015 = call "Write in logger.vi"("error in"=w1826, "String in"=w1827, "logger refnum"=w1831) -> ("error out"=w1825:errorcluster)  [unwired: 1 in, 1 out]
                    n1016 = property on="THz control" class="Clust (strict)"("DisabledEnum"=w1805) -> ()  [unwired: 2 in, 2 out]
                    n1017 = call "simple Shift string array.vi"("Element in"=w1812, "Array in"=w1839) -> ("Array out"=w1838:string[])  [unwired: 8 in, 1 out]
                    n1018 = call <vilib>:"Clear Errors.vi"("error in (no error)"=w1825) -> ()  [unwired: 5 in, 2 out]
                  }
                  frame "Update" {
                  }
                  frame "Set parameters" {
                    n1019 = Variant To Data(type=T44 {"Start [GHz]"=8.0, "End [GHz] "=8.0, "Sweep up\ntime [ms]"=0.0, "Sweep down\ntime [ms]"=0.0, "Intermidiate [MHz]"=0.0, "Reset trigger"=FALSE} ("Sweep parameters"), Variant=w1871) -> (data=w1859:T44, error out=w1861:errorcluster)  [unwired: 1 in]
                    n1020 = Unbundle By Name(w1844) -> ("Experiment state"=w1843:T25)
                    n1021 = Unbundle By Name(w1859) -> ("Start [GHz]"=w1856:dbl, "End [GHz]"=w1855:dbl, "Sweep up\ntime [ms]"=w1854:dbl, "Intermidiate [MHz]"=w1858:dbl)
                    n1022 = local read "THz control"() -> (w1867:T21)
                    n1023 = Unbundle By Name(w1867) -> ("AMC"=w1868:u16, "Multip"=w1869:u16)
                    n1024 = Multiply(x=w1868, y=w1869) -> (x*y=w1857:u16)
                    n1025 = Multiply(x=w1856, y=w1857) -> (x*y=w1847:dbl)
                    n1026 = Multiply(x=w1855, y=w1857) -> (x*y=w1846:dbl)
                    n1027 = Multiply(x=w1854, y=w1857) -> (x*y=w1853:dbl)
                    n1028 = Multiply(x=w1858, y=w1857) -> (x*y=w1845:dbl)
                    n1029 = Equal To 0?(x=w1853) -> (x = 0?=w1865:bool)
                    n1030 = Select(t="CW", s=w1865, f="Sweep") -> (s? t:f=w1862:string)
                    n1031 = Bundle By Name(cluster=w1844, "Experiment state"=w1843) -> (w1860:T24)
                    n1032 = Format Into String(format string="THz source set to %s mode at %f GHz ", error in=w1861, w1862, w1847) -> (resulting string=w1852:string)  [unwired: 1 in, 1 out]
                    n1033 = Bundle By Name(cluster=w1850, "Last update"=w1848, "Start [GHz]"=w1847, "End [GHz]"=w1846, "Im Freq[MHz]"=w1845) -> (w1849:T85)
                    n1034 = call "Add actual date time to string.vi"("String in"=w1852) -> ("String out"=w1851:string)  [unwired: 4 in]
                    n1035 = call "simple Shift string array.vi"("Element in"=w1851, "Array in"=w1872) -> ("Array out"=w1873:string[])  [unwired: 8 in, 1 out]
                  }
                  frame "End" {
                    w1883 = "None" ("Master")
                    n1036 = Variant To Data(type="", Variant=w1880) -> (data=w1875:string)  [unwired: 1 in, 1 out]
                    n1037 = Bundle By Name(cluster=w1885, "Name"=w1883, "Description"=w1883, "Last update"=w1882) -> (w1884:T85)
                    n1038 = property on="THz" class="Bool (strict)"("Value"=FALSE) -> ()  [unwired: 2 in, 2 out]
                    n1039 = call "Add actual date time to string.vi"("String in"="Excitation module (VDI) ended") -> ("String out"=w1877:string)  [unwired: 4 in]
                    n1040 = Concatenate Strings(w1877, "\r\n", w1875) -> (w1876:string)
                    n1041 = local read "loggersRef"() -> (w1888:refnum<file>)
                    n1042 = call "Write in logger.vi"("String in"=w1876, "logger refnum"=w1888) -> ()  [unwired: 2 in, 2 out]
                    n1043 = call "simple Shift string array.vi"("Element in"=w1876, "Array in"=w1878) -> ("Array out"=w1879:string[])  [unwired: 8 in, 1 out]
                  }
                  frame "Disconnect" {
                    w1899 = "None" ("Master")
                    n1044 = Variant To Data(type="", Variant=w1896) -> (data=w1891:string)  [unwired: 1 in, 1 out]
                    n1045 = Bundle By Name(cluster=w1901, "Name"=w1899, "Description"=w1899, "Last update"=w1898) -> (w1900:T85)
                    n1046 = property on="THz" class="Bool (strict)"("Value"=FALSE) -> ()  [unwired: 2 in, 2 out]
                    n1047 = call "Add actual date time to string.vi"("String in"="Microwave excitation module Disconnected") -> ("String out"=w1893:string)  [unwired: 4 in]
                    n1048 = Concatenate Strings(w1893, "\r\n", w1891) -> (w1892:string)
                    n1049 = local read "loggersRef"() -> (w1904:refnum<file>)
                    n1050 = call "Write in logger.vi"("String in"=w1892, "logger refnum"=w1904) -> ()  [unwired: 2 in, 2 out]
                    n1051 = call "simple Shift string array.vi"("Element in"=w1892, "Array in"=w1894) -> ("Array out"=w1895:string[])  [unwired: 8 in, 1 out]
                  }
                }
                n1052 = Bundle By Name(cluster=w1774, "THz"=w1771) -> (w1772:T8)
              }
              frame "Digitizer" {
                n1053 = Unbundle By Name(w1909) -> ("THz"=w1908:T85)
                n1054 = case shown="\"Ignore\", Default" w1917 {
                  tunnel: w1916 -> [w1920]
                  tunnel: [w1920] -> w1915
                  tunnel: w1914 -> [_]
                  tunnel: w1913 -> [_]
                  tunnel: w1911 -> [w1919]
                  tunnel: [w1919] -> w1912
                  tunnel: w1910 -> [_]
                  tunnel: w1908 -> [w1918]
                  tunnel: [w1918] -> w1906
                  frame "Ignore", Default {
                  }
                }
                n1055 = Bundle By Name(cluster=w1909, "THz"=w1906) -> (w1907:T8)
              }
              frame "Carousel" {
                n1056 = Unbundle By Name(w1924) -> ("THz"=w1923:T85)
                n1057 = case shown="\"Ignore\", Default" w1932 {
                  tunnel: w1931 -> [w1935]
                  tunnel: [w1935] -> w1930
                  tunnel: w1929 -> [_]
                  tunnel: w1928 -> [_]
                  tunnel: w1926 -> [w1934]
                  tunnel: [w1934] -> w1927
                  tunnel: w1925 -> [_]
                  tunnel: w1923 -> [w1933]
                  tunnel: [w1933] -> w1921
                  frame "Ignore", Default {
                  }
                }
                n1058 = Bundle By Name(cluster=w1924, "THz"=w1921) -> (w1922:T8)
              }
              frame "Multimeter" {
                n1059 = Unbundle By Name(w1939) -> ("THz"=w1938:T85)
                n1060 = case shown="\"Get value\"" w1947 {
                  tunnel: w1946 -> [w1950 w1953]
                  tunnel: [w1950 w1953] -> w1945
                  tunnel: w1944 -> [_ _]
                  tunnel: w1943 -> [_ _]
                  tunnel: w1941 -> [w1949 w1952]
                  tunnel: [w1949 w1952] -> w1942
                  tunnel: w1940 -> [_ _]
                  tunnel: w1938 -> [w1948 w1951]
                  tunnel: [w1948 w1951] -> w1936
                  frame "Ignore", Default {
                  }
                  frame "Get value" {
                  }
                }
                n1061 = Bundle By Name(cluster=w1939, "THz"=w1936) -> (w1937:T8)
              }
              frame "Power monitor" {
                n1062 = Unbundle By Name(w1957) -> ("PwrMonitor"=w1956:T86)
                n1063 = case shown="\"Update\"" w1965 {
                  tunnel: w1964 -> [w1968 w1973 w1976]
                  tunnel: [w1968 w1973 w1976] -> w1963
                  tunnel: w1962 -> [_ w1971 _]
                  tunnel: w1961 -> [_ _ _]
                  tunnel: w1959 -> [w1967 w1972 w1975]
                  tunnel: [w1967 w1972 w1975] -> w1960
                  tunnel: w1958 -> [_ _ _]
                  tunnel: w1956 -> [w1966 _ w1974]
                  tunnel: [w1966 w1969 w1974] -> w1954
                  frame "Ignore", Default {
                  }
                  frame "Update" {
                    n1064 = Variant To Data(type=T63 {"Name"="", "Last update"=timestamp(0 s since 1904-01-01), "Outage?"=FALSE, "Low"=FALSE, "No battery"=FALSE, "Battery [%]"=0, "Charging"=FALSE} ("PwrM"), Variant=w1971) -> (data=w1969:T63)  [unwired: 1 in, 1 out]
                  }
                  frame "End" {
                  }
                }
                n1065 = Bundle By Name(cluster=w1957, "PwrMonitor"=w1954) -> (w1955:T8)
              }
              frame "SMU2450" {
                n1066 = Unbundle By Name(w1980) -> ("SMU"=w1979:T87)
                n1067 = case shown="\"Update\"" w1988 {
                  tunnel: w1987 -> [w1991 w2012 w2015 w2036 w2049 w2082 w2101]
                  tunnel: [w1991 w2011 w2015 w2037 w2049 w2083 w2102] -> w1986
                  tunnel: w1985 -> [_ w2007 _ w2035 w2066 w2084 w2103]
                  tunnel: w1984 -> [_ w1997 _ w2031 w2063 w2085 w2104]
                  tunnel: w1982 -> [w1990 w2006 w2014 w2030 w2062 w2089 w2108]
                  tunnel: [w1990 w2006 w2014 w2030 w2062 w2089 w2108] -> w1983
                  tunnel: w1981 -> [_ _ _ _ _ _ _]
                  tunnel: w1979 -> [w1989 w2004 w2013 w2033 w2065 w2088 w2107]
                  tunnel: [w1989 w2003 w2013 w2032 w2064 w2087 w2106] -> w1977
                  frame "Ignore", Default {
                  }
                  frame "Connect" {
                    n1068 = Variant To Data(type=T64 {"VISA name"="", "Connected"=FALSE, "Name"="", "Message"="", "Error message"="", "Min voltage"=0.0, "Max voltage"=0.0, "Min Current"=0.0, "Max Current"=0.0, "Measurement value"=0.0, "Source Voltage"=0.0, "Measurement"=FALSE, "Source Current"=0.0, "Source Mode"=0, "Measure Function"=0} ("output cluster"), Variant=w2007) -> (data=w1999:T64, error out=w2000:errorcluster)  [unwired: 1 in]
                    n1069 = Unbundle By Name(w1999) -> ("Name"=w1992:string, "Message"=w1994:string, "Connected"=w1998:bool)  [unwired: 1 out]
                    n1070 = local read "Instr status"() -> (w2009:T1)
                    n1071 = Bundle By Name(cluster=w2009, "SMU"=w1998) -> (w2010:T1)
                    n1072 = local write "Instr status"(w2010) -> ()
                    n1073 = Concatenate Strings(w1992, " connected. " ("string"), w1994) -> (w1993:string)
                    n1074 = Bundle By Name(cluster=w2004, "Name"=w1992, "Last update"=w1997) -> (w2003:T87)
                    n1075 = property on="SMU controls" class="Clust (strict)"("DisabledEnum"=T33."Enabled" ("Disabled")) -> ()  [unwired: 2 in, 2 out]
                    n1076 = local read "loggersRef"() -> (w2008:refnum<file>)
                    n1077 = call "Add actual date time to string.vi"("String in"=w1993) -> ("String out"=w1996:string)  [unwired: 4 in]
                    n1078 = call "Write in logger.vi"("error in"=w2000, "String in"=w1996, "logger refnum"=w2008) -> ("error out"=w2005:errorcluster)  [unwired: 1 in, 1 out]
                    n1079 = call "simple Shift string array.vi"("Element in"=w1996, "Array in"=w2012) -> ("Array out"=w2011:string[])  [unwired: 8 in, 1 out]
                    n1080 = call <vilib>:"Clear Errors.vi"("error in (no error)"=w2005) -> ()  [unwired: 5 in, 2 out]
                  }
                  frame "Update" {
                  }
                  frame "Set measurement" {
                    # "add surce funcion and value"
                    n1081 = Variant To Data(type=T64 {"VISA name"="", "Connected"=FALSE, "Name"="", "Message"="", "Error message"="", "Min voltage"=0.0, "Max voltage"=0.0, "Min Current"=0.0, "Max Current"=0.0, "Measurement value"=0.0, "Source Voltage"=0.0, "Measurement"=FALSE, "Source Current"=0.0, "Source Mode"=0, "Measure Function"=0} ("SMU status out"), Variant=w2035) -> (data=w2029:T64)  [unwired: 1 in, 1 out]
                    n1082 = Unbundle By Name(w2029) -> ("Measurement value"=w2017:dbl, "Measurement"=w2027:bool, "Source Voltage"=w2025:dbl, "Source Current"=w2026:dbl, "Source Mode"=w2019:u16, "Measure Function"=w2023:u16)
                    n1083 = case shown="0, Default" w2019 {
                      tunnel: w2026 -> [_ w2043]
                      tunnel: w2025 -> [w2041 _]
                      tunnel: [w2041 w2043] -> w2018
                      tunnel: ["Voltage" "Current"] -> w2024
                      frame 0, Default {
                      }
                      frame 1 {
                      }
                    }
                    n1084 = case shown="0, Default" w2023 {
                      tunnel: ["Voltage" "Current"] -> w2022
                      frame 0, Default {
                      }
                      frame 1 {
                      }
                    }
                    n1085 = local read "SMU controls"() -> (w2021:T14)
                    n1086 = Bundle By Name(cluster=w2021, "Measurement settings.Source Mode"=w2019, "Measurement settings.Source Level"=w2018, "Value"=w2017) -> (w2020:T14)
                    n1087 = Bundle By Name(cluster=w2033, "Last update"=w2031, "MeasValue"=w2017, "Output"=w2027, "SourFunc"=w2024, "SourValue"=w2018, "MeasFunc"=w2022) -> (w2032:T87)
                    n1088 = local write "SMU controls"(w2020) -> ()
                    n1089 = call "Add actual date time to string.vi"("String in"="SMU set") -> ("String out"=w2034:string)  [unwired: 4 in]
                    n1090 = call "simple Shift string array.vi"("Element in"=w2034, "Array in"=w2036) -> ("Array out"=w2037:string[])  [unwired: 8 in, 1 out]
                  }
                  frame "Get actual results" {
                    # "add surce funcion and value"
                    n1091 = Variant To Data(type=T64 {"VISA name"="", "Connected"=FALSE, "Name"="", "Message"="", "Error message"="", "Min voltage"=0.0, "Max voltage"=0.0, "Min Current"=0.0, "Max Current"=0.0, "Measurement value"=0.0, "Source Voltage"=0.0, "Measurement"=FALSE, "Source Current"=0.0, "Source Mode"=0, "Measure Function"=0} ("SMU status out"), Variant=w2066) -> (data=w2061:T64)  [unwired: 1 in, 1 out]
                    n1092 = Unbundle By Name(w2061) -> ("Measurement value"=w2047:dbl, "Measurement"=w2059:bool, "Source Voltage"=w2057:dbl, "Source Current"=w2058:dbl, "Source Mode"=w2051:u16, "Measure Function"=w2050:u16)
                    n1093 = Add(x=w2047, y=3.7e-06) -> (x+y=w2045:dbl)
                    n1094 = case shown="1" w2051 {
                      tunnel: w2058 -> [_ w2072]
                      tunnel: w2057 -> [w2070 _]
                      tunnel: [w2070 w2072] -> w2056
                      tunnel: ["Voltage" "Current"] -> w2055
                      frame 0, Default {
                      }
                      frame 1 {
                      }
                    }
                    n1095 = case shown="0, Default" w2050 {
                      tunnel: ["Voltage" "Current"] -> w2054
                      frame 0, Default {
                      }
                      frame 1 {
                      }
                    }
                    n1096 = Divide(x=w2045, y=0.00998) -> (x/y=w2048:dbl)
                    n1097 = local read "SMU controls"() -> (w2053:T14)
                    n1098 = Bundle By Name(cluster=w2053, "Value"=w2045, "B[T]"=w2048) -> (w2052:T14)
                    n1099 = Bundle By Name(cluster=w2065, "Last update"=w2063, "MeasValue"=w2047, "Output"=w2059, "SourFunc"=w2055, "SourValue"=w2056, "MeasFunc"=w2054) -> (w2064:T87)
                    n1100 = local write "SMU controls"(w2052) -> ()
                  }
                  frame "End" {
                    n1101 = Variant To Data(type=T64 {"VISA name"="", "Connected"=FALSE, "Name"="", "Message"="", "Error message"="", "Min voltage"=0.0, "Max voltage"=0.0, "Min Current"=0.0, "Max Current"=0.0, "Measurement value"=0.0, "Source Voltage"=0.0, "Measurement"=FALSE, "Source Current"=0.0, "Source Mode"=0, "Measure Function"=0} ("SMU status out"), Variant=w2084) -> (data=w2077:T64)  [unwired: 1 in, 1 out]
                    n1102 = Unbundle By Name(w2077) -> ("Name"=w2075:string, "Measurement"=w2073:bool)
                    n1103 = Bundle By Name(cluster=w2088, "Name"="None" ("Master"), "Output"=w2073, "Last update"=w2085) -> (w2087:T87)
                    n1104 = property on="SMU" class="Bool (strict)"("Value"=FALSE) -> ()  [unwired: 2 in, 2 out]
                    n1105 = Concatenate Strings("SMU module " ("String in"), w2075, " ended." ("string")) -> (w2076:string)
                    n1106 = call "Add actual date time to string.vi"("String in"=w2076) -> ("String out"=w2081:string)  [unwired: 4 in]
                    n1107 = Concatenate Strings(w2081, "\r\n") -> (w2080:string)
                    n1108 = local read "loggersRef"() -> (w2091:refnum<file>)
                    n1109 = call "Write in logger.vi"("String in"=w2080, "logger refnum"=w2091) -> ()  [unwired: 2 in, 2 out]
                    n1110 = call "simple Shift string array.vi"("Element in"=w2080, "Array in"=w2082) -> ("Array out"=w2083:string[])  [unwired: 8 in, 1 out]
                  }
                  frame "Disconnect" {
                    n1111 = Variant To Data(type=T64 {"VISA name"="", "Connected"=FALSE, "Name"="", "Message"="", "Error message"="", "Min voltage"=0.0, "Max voltage"=0.0, "Min Current"=0.0, "Max Current"=0.0, "Measurement value"=0.0, "Source Voltage"=0.0, "Measurement"=FALSE, "Source Current"=0.0, "Source Mode"=0, "Measure Function"=0} ("SMU status out"), Variant=w2103) -> (data=w2098:T64)  [unwired: 1 in, 1 out]
                    n1112 = Unbundle By Name(w2098) -> ("Name"=w2094:string, "Measurement"=w2093:bool)
                    n1113 = Bundle By Name(cluster=w2107, "Name"="None" ("Master"), "Output"=w2093, "Last update"=w2104) -> (w2106:T87)
                    n1114 = property on="SMU" class="Bool (strict)"("Value"=FALSE) -> ()  [unwired: 2 in, 2 out]
                    n1115 = Concatenate Strings(w2094, " SMU disconnected." ("String in")) -> (w2095:string)
                    n1116 = call "Add actual date time to string.vi"("String in"=w2095) -> ("String out"=w2100:string)  [unwired: 4 in]
                    n1117 = Concatenate Strings(w2100, "\r\n") -> (w2099:string)
                    n1118 = local read "loggersRef"() -> (w2110:refnum<file>)
                    n1119 = call "Write in logger.vi"("String in"=w2099, "logger refnum"=w2110) -> ()  [unwired: 2 in, 2 out]
                    n1120 = call "simple Shift string array.vi"("Element in"=w2099, "Array in"=w2101) -> ("Array out"=w2102:string[])  [unwired: 8 in, 1 out]
                  }
                }
                n1121 = Bundle By Name(cluster=w1980, "SMU"=w1977) -> (w1978:T8)
              }
              frame "Acquisition" {
                n1122 = Unbundle By Name(w2113) -> ("MFLI"=w2116:T88)
                n1123 = case shown="\"Get ModA\"" w2122 {
                  tunnel: w2121 -> [w2147 w2163 w2185 w2204 w2213 w2232 w2242 w2251 _]
                  tunnel: w2120 -> [w2126 w2155 w2179 w2201 w2211 _ _ _ _]
                  tunnel: [w2131 w2159 w2184 w2195 w2214 w2233 w2236 w2245 w2253] -> w2117
                  tunnel: w2118 -> [w2132 w2160 w2184 w2195 w2214 w2233 w2237 w2246 w2253]
                  tunnel: w2116 -> [w2127 w2156 w2182 w2190 w2208 w2229 w2234 w2243 w2252]
                  tunnel: [w2124 w2150 w2180 w2190 w2208 w2229 w2234 w2243 w2252] -> w2115
                  tunnel: w2112 -> [_ _ _ _ _ w2222 _ _ _]
                  frame "Initialize" {
                    w2139 = TRUE ("PSU")
                    w2138 = T33."Enabled" ("Disabled")
                    n1124 = Variant To Data(type="", Variant=w2147) -> (data=w2125:string)  [unwired: 1 in, 1 out]
                    n1125 = Bundle By Name(cluster=w2127, "Last update"=w2126, "Lock-in"=w2125, "Multimeter"="Unknown") -> (w2124:T88)
                    n1126 = local read "Instr status"() -> (w2142:T1)
                    n1127 = Bundle By Name(cluster=w2142, "MFLI"=w2139) -> (w2144:T1)
                    n1128 = Unbundle By Name(w2142) -> ("THz"=w2141:bool, "Mag"=w2140:bool)
                    n1129 = local write "Instr status"(w2144) -> ()
                    n1130 = control-ref of="Acquisition controls"() -> (w2143:refnum<vi>)
                    n1131 = Compound Arithmetic op=AND(w2141, w2140, w2139) -> (w2137:bool)
                    n1132 = Concatenate Strings(w2125, " connected as ACQ" ("String in")) -> (w2129:string)
                    n1133 = Select(t=w2138, s=w2137, f=T33."Disabled and Grayed Out" ("Disabled")) -> (s? t:f=w2133:T33)
                    n1134 = property class="Clust (strict)"(reference=w2143, "DisabledEnum"=w2138) -> ()  [unwired: 1 in, 2 out]
                    n1135 = local read "loggersRef"() -> (w2136:refnum<file>)
                    n1136 = control-ref of="Run script btn"() -> (w2135:refnum<vi>)
                    n1137 = call "Add actual date time to string.vi"("String in"=w2129) -> ("String out"=w2128:string)  [unwired: 4 in]
                    n1138 = Build Array(w2135) -> (w2134:refnum<vi>[])
                    n1139 = call "Write in logger.vi"("String in"=w2128, "logger refnum"=w2136) -> ()  [unwired: 2 in, 2 out]
                    n1140 = call "Dis- or en- able controls.vi"("Disabled"=w2133, "Control referencies"=w2134) -> ()  [unwired: 9 in, 1 out]
                    n1141 = call "simple Shift string array.vi"("Element in"=w2128, "Array in"=w2132) -> ("Array out"=w2131:string[])  [unwired: 8 in, 1 out]
                  }
                  frame "Set parameters" {
                    n1142 = Variant To Data(type=T19 {"Filter order"=1.0, "Filter tau [ms]"=1.0, "F_Mod [kHz]"=0.0, "Amp_Mod [mV]"=0.0, "Enable output"=0, "Phase [°]"=0.0} ("ACQ parameters"), Variant=w2163) -> (data=w2148:T19)  [unwired: 1 in, 1 out]
                    n1143 = local read "Acquisition controls"() -> (w2149:T18)
                    n1144 = Unbundle By Name(w2148) -> ("F_Mod [kHz]"=w2154:dbl, "Amp_Mod [mV]"=w2153:dbl, "Enable output"=w2152:u16)
                    n1145 = property on="ACQ parameters" class="Clust (strict)"("Value"=w2148) -> ()  [unwired: 2 in, 2 out]
                    n1146 = Bundle By Name(cluster=w2149, "ACQ parameters"=w2148) -> (w2161:T18)
                    n1147 = Greater Or Equal To 0?(x=w2152) -> (x >= 0?=w2151:bool)
                    n1148 = local write "Acquisition controls"(w2161) -> ()
                    n1149 = call "Add actual date time to string.vi"("String in"="Lock-in: parameters set" ("Element in")) -> ("String out"=w2157:string)  [unwired: 4 in]
                    n1150 = call "simple Shift string array.vi"("Element in"=w2157, "Array in"=w2160) -> ("Array out"=w2159:string[])  [unwired: 8 in, 1 out]
                    n1151 = Bundle By Name(cluster=w2156, "Last update"=w2155, "Freq [kHz]"=w2154, "Ampl [mV]"=w2153, "OutEn"=w2151) -> (w2150:T88)
                  }
                  frame "Update" {
                    w2176 = 1000.0 ("x")
                    n1152 = Variant To Data(type=T65 {"In50"=FALSE, "InAC"=FALSE, "InDiff"=FALSE, "Out50"=FALSE, "OutEN"=FALSE, "OutF[Hz]"=0.0, "OutA[V]"=0.0, "DemEN"=FALSE, "Const[ms]"=0.0, "Order[-]"=0, "Phase [°]"=0.0} ("Lock-in info"), Variant=w2185) -> (data=w2181:T65)  [unwired: 1 in, 1 out]
                    n1153 = Unbundle By Name(w2181) -> ("OutF[Hz]"=w2178:dbl, "OutA[V]"=w2177:dbl, "OutEN"=w2172:bool, "Out50"=w2169:bool, "In50"=w2166:bool, "Order[-]"=w2168:i32, "Const[ms]"=w2167:dbl, "DemEN"=w2165:bool, "Phase [°]"=w2164:dbl)
                    n1154 = Divide(x=w2178, y=w2176) -> (x/y=w2171:dbl)
                    n1155 = Multiply(x=w2177, y=w2176) -> (x*y=w2170:dbl)
                    n1156 = Boolean To (0,1)(Boolean=w2172) -> (0, 1=w2173:i16)
                    n1157 = local read "Acquisition controls"() -> (w2175:T18)
                    n1158 = Bundle By Name(cluster=w2175, "ACQ parameters.Enable output"=w2173, "ACQ parameters.F_Mod [kHz]"=w2171, "ACQ parameters.Amp_Mod [mV]"=w2170, "Out50"=w2169, "In50"=w2166, "ACQ parameters.Filter order"=w2168, "ACQ parameters.Filter tau [ms]"=w2167, "DemEn"=w2165, "ACQ parameters.Phase [°]"=w2164) -> (w2174:T18)
                    n1159 = Bundle By Name(cluster=w2182, "Last update"=w2179, "Freq [kHz]"=w2171, "Ampl [mV]"=w2170, "OutEn"=w2172, "In50 Ohm"=w2166, "DemEn"=w2165) -> (w2180:T88)
                    n1160 = local write "Acquisition controls"(w2174) -> ()
                  }
                  frame "Get point" {
                    n1161 = local read "Acquisition controls"() -> (w2189:T18)
                    n1162 = Variant To Data(type=T67 {"Timestamps (ticks)"=0, "X (Vrms)"=0.0, "Y (Vrms)"=0.0, "Osc Phase (deg)"=0.0, "Freq (Hz)"=0.0, "DIO"=0, "AuxIn0 (V)"=0.0, "AuxIn1 (V)"=0.0, "Trigger"=0} ("Update data"), Variant=w2204) -> (data=w2202:T67)  [unwired: 1 in, 1 out]
                    n1163 = Unbundle By Name(w2202) -> ("X (Vrms)"=w2193:dbl, "Y (Vrms)"=w2192:dbl, "AuxIn0 (V)"=w2188:dbl, "AuxIn1 (V)"=w2187:dbl)
                    n1164 = Unbundle By Name(w2189) -> ("ACQ shot btn"=w2196:bool)
                    n1165 = Bundle By Name(cluster=w2189, "AuxIn0 [V]"=w2188, "AuxIn1 [V]"=w2187) -> (w2186:T18)
                    n1166 = local read "Tab Control"() -> (w2199:T6)
                    n1167 = local write "Acquisition controls"(w2186) -> ()
                    n1168 = Build Array(w2193, w2192) -> (→"Data":dbl[])
                    n1169 = Equal?(x=w2199, y=T66."Adjustment" ("Tab Control")) -> (x = y?=w2198:bool)
                    n1170 = And(x=w2198, y=w2196) -> (x .and. y?=w2197:bool)
                    n1171 = case shown="True" w2197 {
                      tunnel: w2193 -> [_ w2207]
                      tunnel: w2192 -> [_ w2206]
                      frame False {
                      }
                      frame True {
                        n1172 = Bundle("X (Vrms)"=w2207, "Y (Vrms)"=w2206) -> (→"lookup":cluster{"X (Vrms)":dbl, "Y (Vrms)":dbl})  [unwired: 1 in]
                      }
                    }
                    "New data" <- TRUE ("New data")
                    "data time" <- w2201
                  }
                  frame "Get array" {
                    n1173 = Variant To Data(type=dbl[] [], Variant=w2213) -> (data=w2209:dbl[])  [unwired: 1 in, 1 out]
                    n1174 = local write "data time"(w2211) -> ()
                    n1175 = local write "New data"(TRUE ("New data")) -> ()
                    n1176 = local write "Data"(w2209) -> ()
                  }
                  frame "Get ModA" {
                    n1177 = Variant To Data(type=0.0, Variant=w2232) -> (data=w2215:dbl)  [unwired: 1 in, 1 out]
                    n1178 = local read "Acquisition controls"() -> (w2228:T18)
                    n1179 = Unbundle By Name(w2228) -> ("Sample holder"=w2216:T20, "ACQ parameters.Amp_Mod [mV]"=w2225:dbl)
                    n1180 = local read "Acquisition controls"() -> (w2227:T18)
                    n1181 = Unbundle By Name(w2227) -> ("Desired [G]"=w2226:dbl, "Auto-modulation"=w2221:bool, "ACQ parameters.Enable output"=w2220:u16)
                    n1182 = call "Modulation current to field conversion.vi"("Sample holder"=w2216, "Modulation current (mA)"=w2215) -> ("Modulation field (G)"=w2217:dbl)  [unwired: 9 in]
                    n1183 = Unbundle By Name(w2222) -> ("Data_Aq"=w2223:refnum<queue>)
                    n1184 = Greater Than 0?(x=w2220) -> (x > 0?=w2218:bool)
                    n1185 = And(x=w2221, y=w2218) -> (x .and. y?=w2219:bool)
                    n1186 = call "Modulation amplitude auto adjustment.vi"("Amp_Mod [mV]"=w2225, "Enable auto adjustment"=w2219, "Actual [G]"=w2217, "Desired [G]"=w2226, "Queue in"=w2223) -> ("Adjusted"=w2224:bool)  [unwired: 6 in]
                    n1187 = Bundle By Name(cluster=w2227, "Modulation [A]"=w2215, "Actual [G]"=w2217, "Adj mod"=w2224) -> (w2230:T18)
                    n1188 = local write "Acquisition controls"(w2230) -> ()
                  }
                  frame "End" {
                    n1189 = Variant To Data(type=T68 {"handleValid"=FALSE, "Conn"=0, "Path Prefix"="", "Handle"=0, "Connected"=FALSE, "Clockbase(s)"=0.0} ("Handle Out"), Variant=w2242) -> ()  [unwired: 1 in, 2 out]
                    n1190 = local read "loggersRef"() -> (w2239:refnum<file>)
                    n1191 = property on="MFLI" class="Bool (strict)"("Value"=FALSE) -> ()  [unwired: 2 in, 2 out]
                    n1192 = call "Add actual date time to string.vi"("String in"="ACQ Ended") -> ("String out"=w2235:string)  [unwired: 4 in]
                    n1193 = call "Write in logger.vi"("String in"=w2235, "logger refnum"=w2239) -> ()  [unwired: 2 in, 2 out]
                    n1194 = call "simple Shift string array.vi"("Element in"=w2235, "Array in"=w2237) -> ("Array out"=w2236:string[])  [unwired: 8 in, 1 out]
                  }
                  frame "Disconnect" {
                    n1195 = Variant To Data(type=T68 {"handleValid"=FALSE, "Conn"=0, "Path Prefix"="", "Handle"=0, "Connected"=FALSE, "Clockbase(s)"=0.0} ("Handle Out"), Variant=w2251) -> ()  [unwired: 1 in, 2 out]
                    n1196 = local read "loggersRef"() -> (w2248:refnum<file>)
                    n1197 = property on="MFLI" class="Bool (strict)"("Value"=FALSE) -> ()  [unwired: 2 in, 2 out]
                    n1198 = call "Add actual date time to string.vi"("String in"="ACQ disconnected") -> ("String out"=w2244:string)  [unwired: 4 in]
                    n1199 = call "Write in logger.vi"("String in"=w2244, "logger refnum"=w2248) -> ()  [unwired: 2 in, 2 out]
                    n1200 = call "simple Shift string array.vi"("Element in"=w2244, "Array in"=w2246) -> ("Array out"=w2245:string[])  [unwired: 8 in, 1 out]
                  }
                  frame "Ignore", Default {
                  }
                }
                n1201 = Bundle By Name(cluster=w2113, "MFLI"=w2115) -> (w2114:T8)
              }
              frame "VTI" {
                n1202 = Unbundle By Name(w2259) -> ("VTI"=w2257:T84)
                n1203 = case shown="\"Update\"" w2264 {
                  tunnel: w2263 -> [_ w2284 w2319 w2335 _ _]
                  tunnel: w2262 -> [w2267 w2282 w2317 w2331 w2368 w2381]
                  tunnel: [w2267 w2281 w2317 w2330 w2367 w2380] -> w2261
                  tunnel: w2254 -> [w2266 w2272 w2315 w2333 w2363 w2376]
                  tunnel: [w2266 w2272 w2314 w2333 w2363 w2376] -> w2260
                  tunnel: w2257 -> [w2265 w2271 w2302 w2332 w2362 w2375]
                  tunnel: w2256 -> [_ _ w2306 _ _ _]
                  tunnel: [w2265 w2270 w2313 w2332 w2361 w2374] -> w2255
                  frame "Ignore", Default {
                  }
                  frame "Initialize" {
                    n1204 = Variant To Data(type="", Variant=w2284) -> (data=w2269:string)  [unwired: 1 in, 1 out]
                    n1205 = local read "Instr status"() -> (w2278:T1)
                    n1206 = Bundle By Name(cluster=w2278, "VTI"=TRUE) -> (w2277:T1)
                    n1207 = local write "Instr status"(w2277) -> ()
                    n1208 = Concatenate Strings("Temperature controller " ("string"), w2269, " initialized" ("string")) -> (w2273:string)
                    n1209 = local read "loggersRef"() -> (w2274:refnum<file>)
                    n1210 = call "Add actual date time to string.vi"("String in"=w2273) -> ("String out"=w2275:string)  [unwired: 4 in]
                    n1211 = call "Write in logger.vi"("String in"=w2275, "logger refnum"=w2274) -> ()  [unwired: 2 in, 2 out]
                    n1212 = property on="VTI control" class="Clust (strict)"("DisabledEnum"=T33."Enabled" ("Disabled")) -> ()  [unwired: 2 in, 2 out]
                    n1213 = Bundle By Name(cluster=w2271, "TempCtl"=w2269) -> (w2270:T84)
                    n1214 = call "simple Shift string array.vi"("Element in"=w2273, "Array in"=w2282) -> ("Array out"=w2281:string[])  [unwired: 8 in, 1 out]
                  }
                  frame "Update" {
                    n1215 = Variant To Data(type=T69 {"VTI space"=0.0, "Sample"=0.0, "He pot"=0.0, "Trap"=0.0, "Ambient"=0.0, "SetP_VTI"=0.0, "SetP_Smp"=0.0, "SetP_Pot"=0.0, "SetP_Trap"=0.0, "Range out 1"=1, "Out 1 [%]"=0.0, "Out 2 [%]"=0.0} ("TC sensors [K]"), Variant=w2319) -> (data=w2316:T69)  [unwired: 1 in, 1 out]
                    n1216 = Unbundle(w2316) -> ("VTI space"=w2288:dbl, "Sample"=w2285:dbl, "He pot"=w2286:dbl, "Trap"=w2287:dbl, "Ambient"=w2293:dbl, "SetP_VTI"=w2310:dbl, "SetP_Smp"=w2309:dbl, "SetP_Pot"=w2308:dbl, "SetP_Trap"=w2307:dbl, "Range out 1"=w2289:u16, "Out 1 [%]"=w2291:dbl, "Out 2 [%]"=w2290:dbl)
                    n1217 = Unbundle(w2302) -> ("VTI [K]"=w2298:dbl, "Sample [K]"=w2299:dbl, "Trap[K]"=w2300:dbl, "HePot [K]"=w2301:dbl)  [unwired: 3 out]
                    n1218 = local read "VTI control"() -> (w2312:T17)
                    n1219 = Bundle By Name(cluster=w2315, "T_sample [K]"=w2285) -> (w2314:T24)
                    n1220 = Build Array(w2288, w2285, w2287, w2286) -> (w2294:dbl[])
                    n1221 = Bundle By Name(cluster=w2302, "Last update"=w2306, "VTI [K]"=w2288, "Sample [K]"=w2285, "HePot [K]"=w2286, "Trap[K]"=w2287, "Ambient [K]"=w2293) -> (w2313:T84)
                    n1222 = Build Array(w2298, w2299, w2300, w2301) -> (w2297:dbl[])
                    n1223 = Bundle(cluster=w2312, "VTI space [K]"=w2310, "Sample [K]"=w2309, "Heater3 [K]"=w2308, "Heater4 [K]"=w2307, "Out 1 [%]"=w2291, "Out 2 [%]"=w2290, "Range out 1"=w2289) -> (w2311:T17)
                    n1224 = Subtract(x=w2294, y=w2297) -> (x-y=w2296:dbl[])
                    n1225 = local read "Drift[K/s]"() -> (w2305:dbl[])
                    n1226 = local write "VTI control"(w2311) -> ()
                    n1227 = Divide(x=w2296, y=2.0) -> (x/y=w2292:dbl[])
                    n1228 = Replace Array Subset(array=w2305, new element=w2292, index=8) -> (w2303:dbl[])
                    n1229 = local write "Drift[K/s]"(w2303) -> ()
                  }
                  frame "Set point" {
                    n1230 = Variant To Data(type=T50 {"Heater"="", "Tmp [K]"=0.0}, Variant=w2335) -> (data=w2334:T50)  [unwired: 1 in, 1 out]
                    n1231 = Unbundle By Name(w2334) -> ("Heater"=w2324:string, "Tmp [K]"=w2321:dbl)
                    n1232 = local read "VTI control"() -> (w2323:T17)
                    n1233 = case shown="\"VTI space [K]\"" w2324 {
                      selector: w2324 -> [_ w2339 w2344 w2352 w2357]
                      tunnel: [u16 0 ("Output's Control Loop (1:1)") w2343 w2348 w2353 w2358] -> _
                      tunnel: w2321 -> [_ w2340 w2345 w2349 w2354]
                      tunnel: w2323 -> [w2337 w2342 w2347 w2351 w2356]
                      tunnel: [w2337 w2341 w2346 w2350 w2355] -> w2322
                      tunnel: ["Unknown setpoint" w2339 w2344 w2352 w2357] -> w2320
                      frame "None", Default {
                      }
                      frame "VTI space [K]" {
                        w2343 = u16 1 items=["1"=1, "2"=2, "3"=3, "4"=4] ("Output's Control Loop (1:1)")
                        n1234 = Bundle By Name(cluster=w2342, "VTI space [K]"=w2340) -> (w2341:T17)
                      }
                      frame "Sample [K]" {
                        w2348 = u16 2 items=["1"=1, "2"=2, "3"=3, "4"=4] ("Output's Control Loop (1:1)")
                        n1235 = Bundle By Name(cluster=w2347, "Sample [K]"=w2345) -> (w2346:T17)
                      }
                      frame "Heater3 [K]" {
                        w2353 = u16 3 items=["1"=1, "2"=2, "3"=3, "4"=4] ("Output's Control Loop (1:1)")
                        n1236 = Bundle By Name(cluster=w2351, "Heater3 [K]"=w2349) -> (w2350:T17)
                      }
                      frame "Heater4 [K]" {
                        w2358 = u16 4 items=["1"=1, "2"=2, "3"=3, "4"=4] ("Output's Control Loop (1:1)")
                        n1237 = Bundle By Name(cluster=w2356, "Heater4 [K]"=w2354) -> (w2355:T17)
                      }
                    }
                    n1238 = local write "VTI control"(w2322) -> ()
                    n1239 = Format Into String(format string="%f K", initial string=w2320, w2321) -> (resulting string=w2328:string)  [unwired: 1 in, 1 out]
                    n1240 = local read "loggersRef"() -> (w2329:refnum<file>)
                    n1241 = call "Add actual date time to string.vi"("String in"=w2328) -> ("String out"=w2326:string)  [unwired: 4 in]
                    n1242 = call "simple Shift string array.vi"("Element in"=w2326, "Array in"=w2331) -> ("Array out"=w2330:string[])  [unwired: 8 in, 1 out]
                    n1243 = call "Write in logger.vi"("String in"=w2326, "logger refnum"=w2329) -> ()  [unwired: 2 in, 2 out]
                  }
                  frame "End" {
                    w2365 = "VTI closed" ("Element in")
                    n1244 = local read "Instr status"() -> (w2371:T1)
                    n1245 = Bundle By Name(cluster=w2362, "TempCtl"="None" ("TC")) -> (w2361:T84)
                    n1246 = Bundle By Name(cluster=w2371, "VTI"=FALSE) -> (w2369:T1)
                    n1247 = local write "Instr status"(w2369) -> ()
                    n1248 = property on="VTI control" class="Clust (strict)"("DisabledEnum"=T33."Disabled and Grayed Out" ("Disabled")) -> ()  [unwired: 2 in, 2 out]
                    n1249 = call "Add actual date time to string.vi"("String in"=w2365) -> ("String out"=w2364:string)  [unwired: 4 in]
                    n1250 = local read "loggersRef"() -> (w2366:refnum<file>)
                    n1251 = call "simple Shift string array.vi"("Element in"=w2365, "Array in"=w2368) -> ("Array out"=w2367:string[])  [unwired: 8 in, 1 out]
                    n1252 = call "Write in logger.vi"("String in"=w2364, "logger refnum"=w2366) -> ()  [unwired: 2 in, 2 out]
                  }
                  frame "Disconnect" {
                    w2378 = "VTI Disconnected" ("Element in")
                    n1253 = local read "Instr status"() -> (w2384:T1)
                    n1254 = Bundle By Name(cluster=w2375, "TempCtl"="None" ("TC")) -> (w2374:T84)
                    n1255 = Bundle By Name(cluster=w2384, "VTI"=FALSE) -> (w2382:T1)
                    n1256 = local write "Instr status"(w2382) -> ()
                    n1257 = property on="VTI control" class="Clust (strict)"("DisabledEnum"=T33."Disabled and Grayed Out" ("Disabled")) -> ()  [unwired: 2 in, 2 out]
                    n1258 = call "Add actual date time to string.vi"("String in"=w2378) -> ("String out"=w2377:string)  [unwired: 4 in]
                    n1259 = local read "loggersRef"() -> (w2379:refnum<file>)
                    n1260 = call "simple Shift string array.vi"("Element in"=w2378, "Array in"=w2381) -> ("Array out"=w2380:string[])  [unwired: 8 in, 1 out]
                    n1261 = call "Write in logger.vi"("String in"=w2377, "logger refnum"=w2379) -> ()  [unwired: 2 in, 2 out]
                  }
                }
                n1262 = Bundle By Name(cluster=w2259, "VTI"=w2255) -> (w2258:T8)
              }
              frame "Servo" {
                n1263 = Unbundle By Name(w2389) -> ("Servo"=w2387:T10[])
                n1264 = case shown="\"Update\"" w2391 {
                  selector: w2391 -> [w2411 w2459 w2512 _ _ w2654]
                  tunnel: w2394 -> [w2413 w2461 w2519 _ _ w2652]
                  tunnel: w2393 -> [w2409 w2457 w2515 w2598 w2638 w2657]
                  tunnel: [w2410 w2458 w2516 w2599 w2639 w2656] -> w2392
                  tunnel: w2387 -> [w2396 w2445 w2498 w2566 w2631 w2646]
                  tunnel: [w2395 w2447 w2497 w2595 w2634 w2646] -> w2386
                  tunnel: w2385 -> [w2397 _ w2495 _ _ _]
                  frame "Initialize" {
                    n1265 = Variant To Data(type=T70[] [] ("Servo status"), Variant=w2413) -> (data=w2399:T70[])  [unwired: 1 in, 1 out]
                    n1266 = Index Array(array=w2396) -> (element=w2398:T10)  [unwired: 1 in]
                    n1267 = for {
                      tunnel: w2399 -> [w2429] mode=indexing
                      tunnel: w2398 -> [w2425]
                      tunnel: w2397 -> [w2423]
                      tunnel: [w2417] -> w2395 mode=indexing
                      n1268 = Unbundle By Name(w2429) -> ("Servo constants.Name"=w2424:T11, "Servo variables.Actual position"=w2422:dbl, "Servo constants.Pos position limit [mm]"=w2419:dbl, "Servo constants.Neg position limit [mm]"=w2418:dbl, "Servo variables.Power ON"=w2420:bool, "Servo variables.Connected"=w2421:bool)
                      n1269 = Select(t=T33."Enabled" ("Disabled"), s=w2421, f=T33."Disabled and Grayed Out" ("Disabled")) -> (s? t:f=w2426:T33)
                      n1270 = Bundle By Name(cluster=w2425, "Name"=w2424, "Last update"=w2423, "Position"=w2422, "Pos limit"=w2419, "Neg limit"=w2418, "Power"=w2420) -> (w2417:T10)
                      n1271 = case shown="\"AxisX\", Default" w2424 {
                        tunnel: w2422 -> [w2431 w2433 w2435 w2437 w2439]
                        tunnel: w2421 -> [_ _ _ _ _]
                        tunnel: w2426 -> [w2430 w2432 w2434 w2436 w2438]
                        frame "AxisX", Default {
                          n1272 = property on="X backward" class="Bool"("DisabledEnum"=w2430) -> ()  [unwired: 2 in, 2 out]
                          n1273 = property on="X forward" class="Bool"("DisabledEnum"=w2430) -> ()  [unwired: 2 in, 2 out]
                          n1274 = property on="X" class="DigNum (strict)"("Val(Sgnl)"=w2431) -> ()  [unwired: 2 in, 2 out]
                        }
                        frame "AxisY" {
                          n1275 = property on="Y left" class="Bool"("DisabledEnum"=w2432) -> ()  [unwired: 2 in, 2 out]
                          n1276 = property on="Y right" class="Bool"("DisabledEnum"=w2432) -> ()  [unwired: 2 in, 2 out]
                          n1277 = property on="Y" class="DigNum (strict)"("Value"=w2433) -> ()  [unwired: 2 in, 2 out]
                        }
                        frame "AxisZ_left" {
                          n1278 = property on="ZLup" class="Bool"("DisabledEnum"=w2434) -> ()  [unwired: 2 in, 2 out]
                          n1279 = property on="ZLdown" class="Bool"("DisabledEnum"=w2434) -> ()  [unwired: 2 in, 2 out]
                          n1280 = property on="ZL" class="DigNum (strict)"("Value"=w2435) -> ()  [unwired: 2 in, 2 out]
                        }
                        frame "AxisZ_middle" {
                          n1281 = property on="ZM" class="DigNum (strict)"("Value"=w2437) -> ()  [unwired: 2 in, 2 out]
                          n1282 = property on="ZMdown" class="Bool"("DisabledEnum"=w2436) -> ()  [unwired: 2 in, 2 out]
                          n1283 = property on="ZMup" class="Bool"("DisabledEnum"=w2436) -> ()  [unwired: 2 in, 2 out]
                        }
                        frame "AxisZ_right" {
                          n1284 = property on="ZRup" class="Bool"("DisabledEnum"=w2438) -> ()  [unwired: 2 in, 2 out]
                          n1285 = property on="ZRdown" class="Bool"("DisabledEnum"=w2438) -> ()  [unwired: 2 in, 2 out]
                          n1286 = property on="ZR" class="DigNum (strict)"("Value"=w2439) -> ()  [unwired: 2 in, 2 out]
                        }
                      }
                    }
                    n1287 = for {
                      tunnel: w2399 -> [w2441] mode=indexing
                      tunnel: [w2440] -> w2403 mode=indexing
                      n1288 = Unbundle By Name(w2441) -> ("Servo variables.Connected"=w2440:bool)
                    }
                    n1289 = And Array Elements(Boolean array=w2403) -> (logical AND=w2402:bool)
                    n1290 = call <vilib>:"Space Constant.vi"() -> ("String"=w2405:string)
                    n1291 = case shown="True" w2402 {
                      frame False {
                      }
                      frame True {
                        n1292 = control-ref of="Servo controls"() -> (w2416:refnum<vi>)
                        n1293 = Build Array(w2416) -> (w2415:refnum<vi>[])
                        n1294 = call "Dis- or en- able controls.vi"("Disabled"=T33."Enabled", "Control referencies"=w2415) -> ()  [unwired: 9 in, 1 out]
                      }
                    }
                    n1295 = local read "Instr status"() -> (w2408:T1)
                    n1296 = Concatenate Strings("Servo" ("string"), w2405, w2411, w2405) -> (w2412:string)
                    n1297 = local read "loggersRef"() -> (w2401:refnum<file>)
                    n1298 = Bundle By Name(cluster=w2408, "Serv"=w2402) -> (w2407:T1)
                    n1299 = call "Add actual date time to string.vi"("String in"=w2412) -> ("String out"=w2400:string)  [unwired: 4 in]
                    n1300 = local write "Instr status"(w2407) -> ()
                    n1301 = call "simple Shift string array.vi"("Element in"=w2400, "Array in"=w2409) -> ("Array out"=w2410:string[])  [unwired: 8 in, 1 out]
                    n1302 = call "Write in logger.vi"("String in"=w2400, "logger refnum"=w2401) -> ()  [unwired: 2 in, 2 out]
                  }
                  frame "Move by" {
                    n1303 = Variant To Data(type=T73 {"Property"="", "Value"=variant, "Name"=enum."AxisX"} ("Array"), Variant=w2461) -> (data=w2453:T73)  [unwired: 1 in, 1 out]
                    n1304 = Unbundle By Name(w2453) -> ("Property"=w2452:string, "Value"=w2451:variant, "Name"=w2450:T11)
                    n1305 = call "Extract axis properties.vi"("Name"=w2450, "All servo status"=w2445) -> ("Servo"=w2444:T10, "Index"=w2446:i32, "Found?"=w2448:bool)  [unwired: 6 in]
                    n1306 = case shown="True" w2448 {
                      tunnel: w2452 -> [w2463 w2472]
                      tunnel: w2451 -> [_ w2471]
                      tunnel: w2450 -> [_ w2470]
                      tunnel: w2444 -> [_ w2469]
                      tunnel: w2446 -> [_ w2468]
                      tunnel: w2445 -> [w2462 w2467]
                      tunnel: [w2463 w2465] -> w2449
                      tunnel: [w2462 w2464] -> w2447
                      frame False {
                      }
                      frame True {
                        n1307 = case shown="\"Power ON\"" w2472 {
                          selector: w2472 -> [w2473 w2476 w2488]
                          tunnel: w2471 -> [_ w2475 w2494]
                          tunnel: w2470 -> [_ w2478 _]
                          tunnel: w2469 -> [w2474 w2481 w2492]
                          tunnel: [w2474 w2480 w2491] -> w2466
                          tunnel: [w2473 w2479 w2490] -> w2465
                          frame "Nothing", Default {
                          }
                          frame "Actual position" {
                            n1308 = Variant To Data(type=0.0, Variant=w2475) -> (data=w2477:dbl)  [unwired: 1 in, 1 out]
                            n1309 = case shown="\"AxisZ_right\"" w2478 {
                              tunnel: w2477 -> [w2483 w2484 w2485 w2486 w2487]
                              frame "AxisX", Default {
                                n1310 = property on="X" class="DigNum (strict)"("Val(Sgnl)"=w2483) -> ()  [unwired: 2 in, 2 out]
                              }
                              frame "AxisY" {
                                n1311 = property on="Y" class="DigNum (strict)"("Value"=w2484) -> ()  [unwired: 2 in, 2 out]
                              }
                              frame "AxisZ_left" {
                                n1312 = property on="ZL" class="DigNum (strict)"("Value"=w2485) -> ()  [unwired: 2 in, 2 out]
                              }
                              frame "AxisZ_middle" {
                                n1313 = property on="ZM" class="DigNum (strict)"("Value"=w2486) -> ()  [unwired: 2 in, 2 out]
                              }
                              frame "AxisZ_right" {
                                n1314 = property on="ZR" class="DigNum (strict)"("Value"=w2487) -> ()  [unwired: 2 in, 2 out]
                              }
                            }
                            n1315 = Bundle By Name(cluster=w2481, "Position"=w2477) -> (w2480:T10)
                            n1316 = Format Into String(initial string=w2476, w2477) -> (resulting string=w2479:string)  [unwired: 2 in, 1 out]
                          }
                          frame "Power ON" {
                            n1317 = Variant To Data(type=FALSE ("Connected"), Variant=w2494) -> (data=w2489:bool)  [unwired: 1 in, 1 out]
                            n1318 = Bundle By Name(cluster=w2492, "Power"=w2489) -> (w2491:T10)
                            n1319 = Format Into String(initial string=w2488, w2489) -> (resulting string=w2490:string)  [unwired: 2 in, 1 out]
                          }
                        }
                        n1320 = Replace Array Subset(array=w2467, new element=w2466, index=w2468) -> (w2464:T10[])
                      }
                    }
                    n1321 = call <vilib>:"Space Constant.vi"() -> ("String"=w2455:string)
                    n1322 = local read "loggersRef"() -> (w2442:refnum<file>)
                    n1323 = Concatenate Strings("Servo" ("string"), w2455, w2459, w2455, w2449) -> (w2460:string)
                    n1324 = call "Add actual date time to string.vi"("String in"=w2460) -> ("String out"=w2443:string)  [unwired: 4 in]
                    n1325 = call "Write in logger.vi"("String in"=w2443, "logger refnum"=w2442) -> ()  [unwired: 2 in, 2 out]
                    n1326 = call "simple Shift string array.vi"("Element in"=w2443, "Array in"=w2457) -> ("Array out"=w2458:string[])  [unwired: 8 in, 1 out]
                  }
                  frame "Update" {
                    n1327 = Variant To Data(type=T73 {"Property"="", "Value"=variant, "Name"=enum."AxisX"} ("Array"), Variant=w2519) -> (data=w2511:T73)  [unwired: 1 in, 1 out]
                    n1328 = Unbundle By Name(w2511) -> ("Property"=w2505:string, "Value"=w2510:variant, "Name"=w2507:T11)
                    n1329 = call "Extract axis properties.vi"("Name"=w2507, "All servo status"=w2498) -> ("Servo"=w2509:T10, "Index"=w2508:i32, "Found?"=w2500:bool)  [unwired: 6 in]
                    n1330 = Format Into String(w2507) -> (resulting string=w2506:string)  [unwired: 3 in, 1 out]
                    n1331 = Bundle By Name(cluster=w2509, "Last update"=w2495) -> (w2496:T10)
                    n1332 = call <vilib>:"Space Constant.vi"() -> ("String"=w2502:string)
                    n1333 = Concatenate Strings(w2505, w2502, w2506, ":" ("string"), w2502) -> (w2504:string)
                    n1334 = case shown="True" w2500 {
                      tunnel: w2510 -> [_ w2536]
                      tunnel: w2496 -> [_ w2535]
                      tunnel: w2498 -> [w2520 w2534]
                      tunnel: w2508 -> [_ w2532]
                      tunnel: w2507 -> [w2526 w2531]
                      tunnel: w2505 -> [w2522 w2530]
                      tunnel: w2504 -> [_ w2529]
                      tunnel: [w2524 w2528] -> w2501
                      tunnel: [w2520 w2527] -> w2497
                      frame False {
                        n1335 = call <vilib>:"Space Constant.vi"() -> ("String"=w2521:string)
                        n1336 = Concatenate Strings(w2522, w2521, "Unknown driver" ("initial string")) -> (w2523:string)
                        n1337 = Format Into String(initial string=w2523, w2526) -> (resulting string=w2524:string)  [unwired: 2 in, 1 out]
                      }
                      frame True {
                        n1338 = case shown="\"Actual position\"" w2530 {
                          tunnel: w2536 -> [_ w2546 w2557 w2564]
                          tunnel: w2531 -> [_ w2540 _ _]
                          tunnel: w2535 -> [w2538 w2544 w2555 w2562]
                          tunnel: [w2538 w2543 w2555 w2561] -> w2533
                          tunnel: w2529 -> [w2537 w2542 w2552 w2559]
                          tunnel: [w2537 w2541 w2554 w2560] -> w2528
                          frame "Nothing", Default {
                          }
                          frame "Actual position" {
                            n1339 = Variant To Data(type=0.0, Variant=w2546) -> (data=w2539:dbl)  [unwired: 1 in, 1 out]
                            n1340 = case shown="\"AxisZ_left\"" w2540 {
                              tunnel: w2539 -> [w2547 w2548 w2549 w2550 w2551]
                              frame "AxisX", Default {
                                n1341 = property on="X" class="DigNum (strict)"("Val(Sgnl)"=w2547) -> ()  [unwired: 2 in, 2 out]
                              }
                              frame "AxisY" {
                                n1342 = property on="Y" class="DigNum (strict)"("Value"=w2548) -> ()  [unwired: 2 in, 2 out]
                              }
                              frame "AxisZ_left" {
                                n1343 = property on="ZL" class="DigNum (strict)"("Value"=w2549) -> ()  [unwired: 2 in, 2 out]
                              }
                              frame "AxisZ_middle" {
                                n1344 = property on="ZM" class="DigNum (strict)"("Value"=w2550) -> ()  [unwired: 2 in, 2 out]
                              }
                              frame "AxisZ_right" {
                                n1345 = property on="ZR" class="DigNum (strict)"("Value"=w2551) -> ()  [unwired: 2 in, 2 out]
                              }
                            }
                            n1346 = Bundle By Name(cluster=w2544, "Position"=w2539) -> (w2543:T10)
                            n1347 = Format Into String(initial string=w2542, w2539) -> (resulting string=w2541:string)  [unwired: 2 in, 1 out]
                          }
                          frame "Target position" {
                            n1348 = Variant To Data(type=0.0, Variant=w2557) -> (data=w2553:dbl)  [unwired: 1 in, 1 out]
                            n1349 = Format Into String(initial string=w2552, w2553) -> (resulting string=w2554:string)  [unwired: 2 in, 1 out]
                          }
                          frame "Power ON" {
                            n1350 = Variant To Data(type=FALSE ("Connected"), Variant=w2564) -> (data=w2558:bool)  [unwired: 1 in, 1 out]
                            n1351 = Bundle By Name(cluster=w2562, "Power"=w2558) -> (w2561:T10)
                            n1352 = Format Into String(initial string=w2559, w2558) -> (resulting string=w2560:string)  [unwired: 2 in, 1 out]
                          }
                        }
                        n1353 = Replace Array Subset(array=w2534, new element=w2533, index=w2532) -> (w2527:T10[])
                      }
                    }
                    n1354 = call <vilib>:"Space Constant.vi"() -> ("String"=w2499:string)
                    n1355 = Concatenate Strings("Servo" ("string"), w2499, w2512, w2499, w2499, w2499, w2501, w2499) -> (w2513:string)
                    n1356 = call "Add actual date time to string.vi"("String in"=w2513) -> ("String out"=w2517:string)  [unwired: 4 in]
                    n1357 = call "simple Shift string array.vi"("Element in"=w2517, "Array in"=w2515) -> ("Array out"=w2516:string[])  [unwired: 8 in, 1 out]
                  }
                  frame "End" {
                    w2577 = nan
                    n1358 = local read "Instr status"() -> (w2603:T1)
                    n1359 = control-ref of="Servo controls"() -> (w2601:refnum<vi>)
                    n1360 = Bundle By Name(cluster=w2603, "Serv"=FALSE ("PSU")) -> (w2604:T1)
                    n1361 = local write "Instr status"(w2604) -> ()
                    n1362 = Array Size(array=w2566) -> (size(s)=w2596:i32)
                    n1363 = property class="Clust"(reference=w2601, "DisabledEnum"=T33."Disabled and Grayed Out" ("Disabled")) -> ()  [unwired: 1 in, 2 out]
                    n1364 = call "Extract axis properties.vi"("Name"=Axis_names."AxisX", "All servo status"=w2566) -> ("Servo"=w2594:T10, "Found?"=w2589:bool)  [unwired: 6 in, 1 out]
                    n1365 = call "Extract axis properties.vi"("Name"=Axis_names."AxisY", "All servo status"=w2566) -> ("Servo"=w2593:T10, "Found?"=w2587:bool)  [unwired: 6 in, 1 out]
                    n1366 = call "Extract axis properties.vi"("Name"=Axis_names."AxisZ_middle", "All servo status"=w2566) -> ("Servo"=w2592:T10, "Found?"=w2586:bool)  [unwired: 6 in, 1 out]
                    n1367 = call "Extract axis properties.vi"("Name"=Axis_names."AxisZ_left", "All servo status"=w2566) -> ("Servo"=w2591:T10, "Found?"=w2585:bool)  [unwired: 6 in, 1 out]
                    n1368 = call "Extract axis properties.vi"("Name"=Axis_names."AxisZ_right", "All servo status"=w2566) -> ("Servo"=w2590:T10, "Found?"=w2584:bool)  [unwired: 6 in, 1 out]
                    n1369 = Delete From Array(array=w2566, length=w2596) -> (array with subset deleted=w2595:T10[])  [unwired: 1 in, 1 out]
                    n1370 = Unbundle By Name(w2590) -> ("Position"=w2582:dbl)
                    n1371 = Unbundle By Name(w2593) -> ("Position"=w2580:dbl)
                    n1372 = Unbundle By Name(w2592) -> ("Position"=w2581:dbl)
                    n1373 = Unbundle By Name(w2591) -> ("Position"=w2583:dbl)
                    n1374 = Unbundle By Name(w2594) -> ("Position"=w2588:dbl)
                    n1375 = Select(t=w2588, s=w2589, f=w2577) -> (s? t:f=w2567:dbl)
                    n1376 = Select(t=w2580, s=w2587, f=w2577) -> (s? t:f=w2571:dbl)
                    n1377 = Select(t=w2581, s=w2586, f=w2577) -> (s? t:f=w2569:dbl)
                    n1378 = Select(t=w2583, s=w2585, f=w2577) -> (s? t:f=w2570:dbl)
                    n1379 = Select(t=w2582, s=w2584, f=w2577) -> (s? t:f=w2568:dbl)
                    n1380 = Format Into String(format string="\\nX: %f\\tY: %f\\tZM: %f\\tZL: %f\\tZR: %f", initial string="Servo ended " ("Element in"), w2567, w2571, w2569, w2570, w2568) -> (resulting string=w2565:string)  [unwired: 1 in, 1 out]
                    n1381 = local read "loggersRef"() -> (w2597:refnum<file>)
                    n1382 = call "simple Shift string array.vi"("Element in"=w2565, "Array in"=w2598) -> ("Array out"=w2599:string[])  [unwired: 8 in, 1 out]
                    n1383 = call "Write in logger.vi"("String in"=w2565, "logger refnum"=w2597) -> ()  [unwired: 2 in, 2 out]
                  }
                  frame "Disconnect" {
                    w2612 = nan
                    n1384 = local read "Instr status"() -> (w2643:T1)
                    n1385 = control-ref of="Servo controls"() -> (w2641:refnum<vi>)
                    n1386 = Bundle By Name(cluster=w2643, "Serv"=FALSE ("PSU")) -> (w2644:T1)
                    n1387 = Array Size(array=w2631) -> (size(s)=w2635:i32)
                    n1388 = local write "Instr status"(w2644) -> ()
                    n1389 = Delete From Array(array=w2631, length=w2635) -> (array with subset deleted=w2634:T10[])  [unwired: 1 in, 1 out]
                    n1390 = call "Extract axis properties.vi"("Name"=Axis_names."AxisX", "All servo status"=w2631) -> ("Servo"=w2625:T10, "Found?"=w2620:bool)  [unwired: 6 in, 1 out]
                    n1391 = call "Extract axis properties.vi"("Name"=Axis_names."AxisY", "All servo status"=w2631) -> ("Servo"=w2624:T10, "Found?"=w2618:bool)  [unwired: 6 in, 1 out]
                    n1392 = call "Extract axis properties.vi"("Name"=Axis_names."AxisZ_middle", "All servo status"=w2631) -> ("Servo"=w2623:T10, "Found?"=w2617:bool)  [unwired: 6 in, 1 out]
                    n1393 = call "Extract axis properties.vi"("Name"=Axis_names."AxisZ_left", "All servo status"=w2631) -> ("Servo"=w2622:T10, "Found?"=w2616:bool)  [unwired: 6 in, 1 out]
                    n1394 = call "Extract axis properties.vi"("Name"=Axis_names."AxisZ_right", "All servo status"=w2631) -> ("Servo"=w2621:T10, "Found?"=w2615:bool)  [unwired: 6 in, 1 out]
                    n1395 = property class="Clust"(reference=w2641, "DisabledEnum"=T33."Disabled and Grayed Out" ("Disabled")) -> ()  [unwired: 1 in, 2 out]
                    n1396 = Unbundle By Name(w2621) -> ("Position"=w2613:dbl)
                    n1397 = Unbundle By Name(w2624) -> ("Position"=w2610:dbl)
                    n1398 = Unbundle By Name(w2623) -> ("Position"=w2611:dbl)
                    n1399 = Unbundle By Name(w2622) -> ("Position"=w2614:dbl)
                    n1400 = Unbundle By Name(w2625) -> ("Position"=w2619:dbl)
                    n1401 = Select(t=w2619, s=w2620, f=w2612) -> (s? t:f=w2609:dbl)
                    n1402 = Select(t=w2610, s=w2618, f=w2612) -> (s? t:f=w2608:dbl)
                    n1403 = Select(t=w2611, s=w2617, f=w2612) -> (s? t:f=w2607:dbl)
                    n1404 = Select(t=w2614, s=w2616, f=w2612) -> (s? t:f=w2606:dbl)
                    n1405 = Select(t=w2613, s=w2615, f=w2612) -> (s? t:f=w2605:dbl)
                    n1406 = Format Into String(format string="\\nX: %f\\tY: %f\\tZM: %f\\tZL: %f\\tZR: %f", initial string="Servo disconnected " ("Element in"), w2609, w2608, w2607, w2606, w2605) -> (resulting string=w2633:string)  [unwired: 1 in, 1 out]
                    n1407 = local read "loggersRef"() -> (w2637:refnum<file>)
                    n1408 = call "simple Shift string array.vi"("Element in"=w2633, "Array in"=w2638) -> ("Array out"=w2639:string[])  [unwired: 8 in, 1 out]
                    n1409 = call "Write in logger.vi"("String in"=w2633, "logger refnum"=w2637) -> ()  [unwired: 2 in, 2 out]
                  }
                  frame "Error", Default {
                    n1410 = Variant To Data(type=errorcluster {"status"=FALSE, "code"=0, "source"=""} ("error constant"), Variant=w2652) -> (data=w2650:errorcluster)  [unwired: 1 in, 1 out]
                    n1411 = Unbundle By Name(w2650) -> ("source"=w2649:string)
                    n1412 = call <vilib>:"Space Constant.vi"() -> ("String"=w2655:string)
                    n1413 = Concatenate Strings("Servo: " ("string"), w2654, w2655, w2649) -> (w2653:string)
                    n1414 = local read "loggersRef"() -> (w2648:refnum<file>)
                    n1415 = call "Add actual date time to string.vi"("String in"=w2653) -> ("String out"=w2647:string)  [unwired: 4 in]
                    n1416 = call "simple Shift string array.vi"("Element in"=w2647, "Array in"=w2657) -> ("Array out"=w2656:string[])  [unwired: 8 in, 1 out]
                    n1417 = call "Write in logger.vi"("String in"=w2647, "logger refnum"=w2648) -> ()  [unwired: 2 in, 2 out]
                  }
                }
                n1418 = Bundle By Name(cluster=w2389, "Servo"=w2386) -> (w2388:T8)
              }
              frame "Rotator" {
                n1419 = Format Into String(w2666) -> (resulting string=w2664:string)  [unwired: 3 in, 1 out]
                n1420 = Unbundle By Name(w2663) -> ("Magnet.Field [T]"=w2658:dbl, "Rotator"=w2662:T89)
                n1421 = case shown="\"Update\"" w2670 {
                  selector: w2670 -> [_ _ _ w2758 _ w2835 _ _]
                  tunnel: w2669 -> [_ w2690 w2735 w2776 w2815 w2844 w2864 w2891]
                  tunnel: w2668 -> [w2672 w2689 w2733 w2769 w2810 w2842 w2868 w2894]
                  tunnel: [w2672 w2688 w2733 w2768 w2809 w2841 w2867 w2893] -> w2667
                  tunnel: w2664 -> [_ w2685 _ w2759 _ w2836 _ _]
                  tunnel: w2662 -> [w2671 w2680 w2729 w2763 w2813 w2840 w2859 w2887]
                  tunnel: [w2671 w2683 w2730 w2774 w2813 w2840 w2862 w2895] -> w2660
                  tunnel: w2659 -> [_ w2682 w2732 w2773 _ _ w2860 w2888]
                  tunnel: w2658 -> [_ _ w2723 _ _ _ _ _]
                  frame "Ignore", Default {
                  }
                  frame "Initialize" {
                    n1422 = Variant To Data(type=T74 {"Controller info"={"deviceNumber"=0, "DeviceType"=0, "ID"=0, "Serial"="", "Address"="", "connected"=FALSE}, "Handle"=0, "FW-Version"=0, "Features"=0, "Axes"=[], "Path to DLL"=path ""} ("Rotator"), Variant=w2690) -> (data=w2687:T74)  [unwired: 1 in, 1 out]
                    n1423 = Unbundle By Name(w2687) -> ("Controller info.DeviceType"=w2681:i32, "Controller info.connected"=w2686:bool, "Axes"=w2677:T75[])
                    n1424 = property on="Rot" class="Bool (strict)"("Value"=w2686) -> ()  [unwired: 2 in, 2 out]
                    n1425 = case shown="True" w2686 {
                      tunnel: w2689 -> [w2705 w2715]
                      tunnel: [w2705 w2714] -> w2688
                      tunnel: w2685 -> [_ w2710]
                      tunnel: w2681 -> [_ w2711]
                      tunnel: ["None" w2706] -> _
                      frame False {
                      }
                      frame True {
                        n1426 = case shown="2" w2711 {
                          tunnel: ["ANC350res" "ANC350num" "ANC350fps" "Unknown"] -> w2706
                          frame 0, Default {
                          }
                          frame 1 {
                          }
                          frame 2 {
                          }
                          frame 3 {
                          }
                        }
                        n1427 = call <vilib>:"Space Constant.vi"() -> ("String"=w2709:string)
                        n1428 = local read "loggersRef"() -> (w2712:refnum<file>)
                        n1429 = Concatenate Strings(w2710, w2709, "Rotator" ("string"), w2709, w2706) -> (w2713:string)
                        n1430 = call "Add actual date time to string.vi"("String in"=w2713) -> ("String out"=w2707:string)  [unwired: 4 in]
                        n1431 = call "simple Shift string array.vi"("Element in"=w2707, "Array in"=w2715) -> ("Array out"=w2714:string[])  [unwired: 8 in, 1 out]
                        n1432 = call "Write in logger.vi"("String in"=w2707, "logger refnum"=w2712) -> ()  [unwired: 2 in, 2 out]
                      }
                    }
                    n1433 = local read "Piezo controls"() -> (w2675:T15)
                    n1434 = Unbundle By Name(w2675) -> ("Axes properties"=w2676:T16[])
                    n1435 = Unbundle By Name(w2680) -> ("Axes"=w2679:T90)
                    n1436 = for {
                      tunnel: w2677 -> [w2701] mode=indexing
                      tunnel: w2676 -> [w2702]
                      tunnel: [w2703] -> w2674 mode=indexing
                      i -> [w2691]
                      n1437 = Unbundle By Name(w2701) -> ("Frequency [Hz]"=w2697:dbl, "Tolerance [m°]"=w2696:dbl, "DC offset [V]"=w2695:dbl, "Voltage [V]"=w2694:dbl, "Position [°]"=w2693:dbl, "Axis status.EndForward"=w2700:bool, "Axis status.EndBackarwd"=w2699:bool, "Axis status.Error"=w2698:bool)
                      n1438 = Index Array(array=w2702, index=w2691) -> (element=w2692:T16)
                      n1439 = Bundle By Name(cluster=w2692, "Frequency [Hz]"=w2697, "MaxErr [µm|m°]"=w2696, "DC voltage [V]"=w2695, "Amplitude [V]"=w2694, "Position [mm|°]"=w2693, "EoF"=w2700, "EoB"=w2699, "Error"=w2698) -> (w2703:T16)
                    }
                    n1440 = call "Process rotator axes info.vi"("Incoming axes info"=w2677, "Current axes info"=w2679) -> ("Axes info"=w2678:T90)  [unwired: 9 in]
                    n1441 = Bundle By Name(cluster=w2675, "Axes properties"=w2674) -> (w2673:T15)
                    n1442 = Bundle By Name(cluster=w2680, "Name"=w2681, "Last update"=w2682, "Axes"=w2678) -> (w2683:T89)
                    n1443 = local write "Piezo controls"(w2673) -> ()
                  }
                  frame "Update" {
                    n1444 = Variant To Data(type=T75[] [] ("Axis status"), Variant=w2735) -> (data=w2727:T75[])  [unwired: 1 in, 1 out]
                    n1445 = Unbundle By Name(w2729) -> ("Axes"=w2728:T90)
                    n1446 = local read "Piezo controls"() -> (w2726:T15)
                    n1447 = Less Or Equal?(x=w2723, y=8.0) -> (x <= y?=w2721:bool)
                    n1448 = Unbundle By Name(w2726) -> ("Axes properties"=w2725:T16[])
                    n1449 = for {
                      tunnel: w2728 -> [w2740]
                      tunnel: w2727 -> [w2756] mode=indexing
                      tunnel: w2725 -> [w2750]
                      tunnel: [w2749] -> w2724 mode=indexing
                      tunnel: [w2739] -> w2720 mode=indexing
                      i -> [w2736]
                      n1450 = Unbundle By Name(w2756) -> ("Position [°]"=w2748:dbl, "Axis status.Moving"=w2753:bool, "Name"=w2754:string, "ActuatorType"=w2755:u16, "Axis status.Target"=w2752:bool, "Axis status.Connected"=w2751:bool, "Frequency [Hz]"=w2743:dbl, "Voltage [V]"=w2744:dbl, "Axis status.EndForward"=w2745:bool, "Axis status.EndBackarwd"=w2746:bool, "Axis status.Error"=w2747:bool, "Tolerance [m°]"=w2742:dbl, "DC offset [V]"=w2741:dbl)
                      n1451 = Index Array(array=w2740, index=w2736) -> (element=w2738:T91)
                      n1452 = Bundle By Name(cluster=w2738, "Pos [°]"=w2748, "Moving"=w2753, "Name"=w2754, "Actuator"=w2755, "Target"=w2752, "Connected"=w2751) -> (w2739:T91)
                      n1453 = Index Array(array=w2750, index=w2736) -> (element=w2737:T16)
                      n1454 = Bundle By Name(cluster=w2737, "Frequency [Hz]"=w2743, "Amplitude [V]"=w2744, "Position [mm|°]"=w2748, "EoF"=w2745, "EoB"=w2746, "Error"=w2747, "MaxErr [µm|m°]"=w2742, "DC voltage [V]"=w2741) -> (w2749:T16)
                    }
                    n1455 = Bundle By Name(cluster=w2726, "Axes properties"=w2724, "Safe to \nmove?"=w2721) -> (w2731:T15)
                    n1456 = Bundle By Name(cluster=w2729, "Last update"=w2732, "Axes"=w2720) -> (w2730:T89)
                    n1457 = local write "Piezo controls"(w2731) -> ()
                  }
                  frame "Stop movement" {
                    n1458 = local read "Piezo controls"() -> (w2767:T15)
                    n1459 = Variant To Data(type=T75[] [] ("Axis status"), Variant=w2776) -> (data=w2766:T75[])  [unwired: 1 in, 1 out]
                    n1460 = Unbundle By Name(w2767) -> ("Axes properties"=w2765:T16[])
                    n1461 = Unbundle By Name(w2763) -> ("Axes"=w2762:T90)
                    n1462 = for {
                      tunnel: w2766 -> [w2800] mode=indexing
                      tunnel: w2765 -> [w2794] mode=indexing
                      tunnel: [w2793] -> w2761 mode=indexing
                      tunnel: [w2785] -> w2764 mode=indexing
                      tunnel: w2762 -> [w2784] mode=indexing
                      tunnel: ": %s at %.1f° on axis %d" ("format string") -> [w2783]
                      tunnel: w2759 -> [w2782]
                      tunnel: w2758 -> [w2781]
                      tunnel: [w2780] -> w2757
                      i -> [w2779]
                      n1463 = Unbundle By Name(w2800) -> ("Position [°]"=w2778:dbl, "Axis status.Moving"=w2797:bool, "Name"=w2798:string, "ActuatorType"=w2799:u16, "Axis status.Target"=w2796:bool, "Axis status.Connected"=w2795:bool, "Frequency [Hz]"=w2788:dbl, "Voltage [V]"=w2789:dbl, "Axis status.EndForward"=w2790:bool, "Axis status.EndBackarwd"=w2791:bool, "Axis status.Error"=w2792:bool, "Tolerance [m°]"=w2787:dbl, "DC offset [V]"=w2786:dbl)
                      n1464 = Increment(x=w2779) -> (x+1=w2777:i32)
                      n1465 = Bundle By Name(cluster=w2784, "Pos [°]"=w2778, "Moving"=w2797, "Name"=w2798, "Actuator"=w2799, "Target"=w2796, "Connected"=w2795) -> (w2785:T91)
                      n1466 = Bundle By Name(cluster=w2794, "Frequency [Hz]"=w2788, "Amplitude [V]"=w2789, "Position [mm|°]"=w2778, "EoF"=w2790, "EoB"=w2791, "Error"=w2792, "MaxErr [µm|m°]"=w2787, "DC voltage [V]"=w2786) -> (w2793:T16)
                      n1467 = Format Into String(format string=w2783, initial string=w2782, w2781, w2778, w2777) -> (resulting string=w2780:string)  [unwired: 1 in, 1 out]
                    }
                    n1468 = local read "loggersRef"() -> (w2771:refnum<file>)
                    n1469 = call "Add actual date time to string.vi"("String in"=w2757) -> ("String out"=w2770:string)  [unwired: 4 in]
                    n1470 = Bundle By Name(cluster=w2767, "Axes properties"=w2761) -> (w2772:T15)
                    n1471 = call "Write in logger.vi"("String in"=w2770, "logger refnum"=w2771) -> ()  [unwired: 2 in, 2 out]
                    n1472 = Bundle By Name(cluster=w2763, "Last update"=w2773, "Axes"=w2764) -> (w2774:T89)
                    n1473 = call "simple Shift string array.vi"("Element in"=w2770, "Array in"=w2769) -> ("Array out"=w2768:string[])  [unwired: 8 in, 1 out]
                    n1474 = local write "Piezo controls"(w2772) -> ()
                  }
                  frame "Set parameters" {
                    n1475 = local read "Piezo controls"() -> (w2805:T15)
                    n1476 = Variant To Data(type=T16[] [] ("Motion parameters"), Variant=w2815) -> (data=w2807:T16[])  [unwired: 1 in, 1 out]
                    n1477 = Unbundle By Name(w2805) -> ("Axes properties"=w2806:T16[])
                    n1478 = for {
                      tunnel: w2807 -> [w2830] mode=indexing
                      tunnel: w2806 -> [w2831] mode=indexing
                      tunnel: [w2829] -> w2804 mode=indexing
                      tunnel: "%d \\n%s %.1f, %s %.1f, %s %.1f, %s %.1f" ("format string") -> [w2828]
                      tunnel: "Rotator: new parameters set for axis " ("String in") -> [w2827]
                      tunnel: [w2822] -> w2801 mode=concatenating
                      i -> [w2821]
                      n1479 = Unbundle(w2830) -> ("Frequency [Hz]"=w2819:dbl, "MaxErr [µm|m°]"=w2816:dbl, "DC voltage [V]"=w2818:dbl, "Amplitude [V]"=w2817:dbl)  [unwired: 5 out]
                      n1480 = Increment(x=w2821) -> (x+1=w2820:i32)
                      n1481 = Bundle By Name(cluster=w2831, "Frequency [Hz]"=w2819, "MaxErr [µm|m°]"=w2816, "DC voltage [V]"=w2818, "Amplitude [V]"=w2817) -> (w2829:T16)
                      n1482 = Format Into String(format string=w2828, initial string=w2827, w2820, "Freq [Hz]" ("input 1"), w2819, "Range [m°]" ("input 1"), w2816, "DC voltage [V]" ("input 1"), w2818, "Amplitude [Hz]" ("input 1"), w2817) -> (resulting string=w2822:string)  [unwired: 1 in, 1 out]
                    }
                    n1483 = local read "loggersRef"() -> (w2812:refnum<file>)
                    n1484 = Bundle By Name(cluster=w2805, "Axes properties"=w2804) -> (w2808:T15)
                    n1485 = call "Add actual date time to string.vi"("String in"=w2801) -> ("String out"=w2811:string)  [unwired: 4 in]
                    n1486 = call "Write in logger.vi"("String in"=w2811, "logger refnum"=w2812) -> ()  [unwired: 2 in, 2 out]
                    n1487 = local write "Piezo controls"(w2808) -> ()
                    n1488 = call "simple Shift string array.vi"("Element in"=w2811, "Array in"=w2810) -> ("Array out"=w2809:string[])  [unwired: 8 in, 1 out]
                  }
                  frame "Set position" {
                    n1489 = Variant To Data(type=T42[] [] ("Array"), Variant=w2844) -> (data=w2833:T42[])  [unwired: 1 in, 1 out]
                    n1490 = local read "Piezo controls"() -> (w2838:T15)
                    n1491 = Unbundle By Name(w2838) -> ("Axes properties"=w2837:T16[])
                    n1492 = for {
                      tunnel: w2837 -> [w2849] mode=indexing
                      tunnel: w2836 -> [w2853]
                      tunnel: w2835 -> [w2852]
                      tunnel: [w2851] -> w2834 mode=concatenating
                      tunnel: w2833 -> [w2850] mode=indexing
                      tunnel: [w2848] -> w2832 mode=indexing
                      i -> [w2846]
                      n1493 = Unbundle By Name(w2850) -> ("Position [°]"=w2847:dbl)
                      n1494 = Increment(x=w2846) -> (x+1=w2845:i32)
                      n1495 = Bundle By Name(cluster=w2849, "Position [mm|°]"=w2847) -> (w2848:T16)
                      n1496 = Format Into String(format string=": %s on axis %d: %.1f° ", initial string=w2853, w2852, w2845, w2847) -> (resulting string=w2851:string)  [unwired: 1 in, 1 out]
                    }
                    n1497 = Bundle By Name(cluster=w2838, "Axes properties"=w2832) -> (w2839:T15)
                    n1498 = local write "Piezo controls"(w2839) -> ()
                    n1499 = call "simple Shift string array.vi"("Element in"=w2834, "Array in"=w2842) -> ("Array out"=w2841:string[])  [unwired: 8 in, 1 out]
                  }
                  frame "End" {
                    n1500 = Variant To Data(type=T74 {"Controller info"={"deviceNumber"=0, "DeviceType"=0, "ID"=0, "Serial"="", "Address"="", "connected"=FALSE}, "Handle"=0, "FW-Version"=0, "Features"=0, "Axes"=[], "Path to DLL"=path ""} ("Rotator"), Variant=w2864) -> (data=w2863:T74)  [unwired: 1 in, 1 out]
                    n1501 = Unbundle By Name(w2863) -> ("Controller info"=w2861:T92, "Axes"=w2858:T75[])
                    n1502 = Unbundle By Name(w2859) -> ("Axes"=w2857:T90)
                    n1503 = for {
                      tunnel: w2858 -> [w2880] mode=indexing
                      tunnel: w2857 -> [w2882] mode=indexing
                      tunnel: [w2881] -> w2855 mode=indexing
                      n1504 = Unbundle By Name(w2880) -> ("Position [°]"=w2874:dbl, "Axis status.Moving"=w2875:bool, "Name"=w2876:string, "ActuatorType"=w2877:u16, "Axis status.Target"=w2878:bool, "Axis status.Connected"=w2879:bool)
                      n1505 = Bundle(cluster=w2882, "Pos [°]"=w2874, "Moving"=w2875, "Name"=w2876, "Actuator"=w2877, "Target"=w2878, "Connected"=w2879) -> (w2881:T91)
                    }
                    n1506 = Unbundle By Name(w2861) -> ("DeviceType"=w2856:i32)
                    n1507 = Bundle By Name(cluster=w2859, "Name"=w2856, "Last update"=w2860, "Axes"=w2855) -> (w2862:T89)
                    n1508 = local read "Instr status"() -> (w2872:T1)
                    n1509 = local read "loggersRef"() -> (w2870:refnum<file>)
                    n1510 = call "Add actual date time to string.vi"("String in"="Rotator module ended") -> ("String out"=w2866:string)  [unwired: 4 in]
                    n1511 = Bundle By Name(cluster=w2872, "Rot"=FALSE ("PSU")) -> (w2873:T1)
                    n1512 = call "Write in logger.vi"("String in"=w2866, "logger refnum"=w2870) -> ()  [unwired: 2 in, 2 out]
                    n1513 = local write "Instr status"(w2873) -> ()
                    n1514 = call "simple Shift string array.vi"("Element in"=w2866, "Array in"=w2868) -> ("Array out"=w2867:string[])  [unwired: 8 in, 1 out]
                  }
                  frame "Disconnect" {
                    n1515 = Variant To Data(type=T74 {"Controller info"={"deviceNumber"=0, "DeviceType"=0, "ID"=0, "Serial"="", "Address"="", "connected"=FALSE}, "Handle"=0, "FW-Version"=0, "Features"=0, "Axes"=[], "Path to DLL"=path ""} ("Rotator"), Variant=w2891) -> (data=w2889:T74)  [unwired: 1 in, 1 out]
                    n1516 = Unbundle By Name(w2889) -> ("Axes"=w2884:T75[], "Controller info"=w2883:T92)
                    n1517 = Unbundle By Name(w2887) -> ("Axes"=w2885:T90)
                    n1518 = for {
                      tunnel: w2884 -> [w2907] mode=indexing
                      tunnel: w2885 -> [w2909] mode=indexing
                      tunnel: [w2908] -> w2886 mode=indexing
                      n1519 = Unbundle By Name(w2907) -> ("Position [°]"=w2901:dbl, "Axis status.Moving"=w2902:bool, "Name"=w2903:string, "ActuatorType"=w2904:u16, "Axis status.Target"=w2905:bool, "Axis status.Connected"=w2906:bool)
                      n1520 = Bundle(cluster=w2909, "Pos [°]"=w2901, "Moving"=w2902, "Name"=w2903, "Actuator"=w2904, "Target"=w2905, "Connected"=w2906) -> (w2908:T91)
                    }
                    n1521 = Unbundle By Name(w2883) -> ()  [unwired: 1 out]
                    n1522 = Bundle By Name(cluster=w2887, "Last update"=w2888, "Axes"=w2886) -> (w2895:T89)
                    n1523 = local read "Instr status"() -> (w2899:T1)
                    n1524 = local read "loggersRef"() -> (w2897:refnum<file>)
                    n1525 = call "Add actual date time to string.vi"("String in"="Rotator module disconnected") -> ("String out"=w2892:string)  [unwired: 4 in]
                    n1526 = Bundle By Name(cluster=w2899, "Rot"=FALSE ("PSU")) -> (w2900:T1)
                    n1527 = call "Write in logger.vi"("String in"=w2892, "logger refnum"=w2897) -> ()  [unwired: 2 in, 2 out]
                    n1528 = local write "Instr status"(w2900) -> ()
                    n1529 = call "simple Shift string array.vi"("Element in"=w2892, "Array in"=w2894) -> ("Array out"=w2893:string[])  [unwired: 8 in, 1 out]
                  }
                }
                n1530 = Bundle By Name(cluster=w2663, "Rotator"=w2660) -> (w2661:T8)
              }
              frame "Emty", Default {
                n1531 = Format Into String(w2915) -> (resulting string=w2914:string)  [unwired: 3 in, 1 out]
                n1532 = call <vilib>:"Space Constant.vi"() -> ("String"=w2916:string)
                n1533 = Concatenate Strings(w2914, w2916, w2913) -> (w2912:string)
                n1534 = call "simple Shift string array.vi"("Element in"=w2912, "Array in"=w2918) -> ("Array out"=w2917:string[])  [unwired: 8 in, 1 out]
              }
            }
          }
          frame True {
          }
        }
        "Instr info" <- w1413
        n1535 = case shown="False" w1420 {
          selector: w1420 -> [w1439 w1440]
          tunnel: [w1437 TopStates."Check message" ("State")] -> w1418
          tunnel: w1411 -> [w1433 _]
          frame False {
            n1536 = local write "Busy"(w1439) -> ()
            n1537 = Equal?(x=w1433, y=experiment_state."Setup" ("Value")) -> (x = y?=w1435:bool)
            n1538 = Select(t=TopStates."Wait for Event" ("State"), s=w1435, f=TopStates."Check measurement") -> (s? t:f=w1437:T29)
          }
          frame True {
            "Busy" <- w1440
          }
        }
      }
      frame "Check measurement" {
        n1539 = Unbundle By Name(w2922) -> ("Experiment state"=w2924:T25)  [unwired: 1 out]
        n1540 = case shown="\"Stabilization\"" w2924 {
          tunnel: w2930 -> [_ w2958 w2980 _ _ _]
          tunnel: w2926 -> [w2932 w2947 w2988 w3059 w3068 w3144]
          tunnel: w2929 -> [w2934 w2964 w2993 w3063 w3074 w3163]
          tunnel: [w2934 w2962 w2992 w3063 w3074 w3162] -> w2928
          tunnel: [w2933 w2961 w2990 w3062 w3070 w3160] -> w2927
          tunnel: w2922 -> [w2933 w2959 w2991 w3062 w3071 w3161]
          tunnel: [w2932 w2947 w2987 w3059 w3068 w3157] -> w2925
          tunnel: w2923 -> [_ w2939 w2986 _ w3066 _]
          tunnel: w2922 -> [_ _ _ _ w3065 _]
          frame "Setup", Default {
            # "here can be implemented check of input parameters before measurement"
          }
          frame "Preparation" {
            n1541 = local read "THz control"() -> (w2938:T21)
            n1542 = call "Add point to array for XY graph.vi"("Reset?(F)"=TRUE ("Reset?")) -> ()  [unwired: 6 in, 1 out]
            n1543 = Unbundle By Name(w2947) -> ("Mod_A [G]"=w2940:dbl)
            n1544 = call "Prepare measurement.vi"("Instr info"=w2939, "VID control"=w2938, "Script cluster"=w2947, "Referencies in"=w2958) -> ("error out"=w2952:errorcluster)  [unwired: 7 in]
            n1545 = local write "VTI tmp reached"(FALSE ("VTI tmp reached")) -> ()
            n1546 = local read "Acquisition controls"() -> (w2942:T18)
            n1547 = call "Add actual date time to string.vi"("String in"="Preparing for measurement") -> ("String out"=w2965:string)  [unwired: 4 in]
            n1548 = call "simple Shift string array.vi"("Element in"=w2965, "Array in"=w2964) -> ("Array out"=w2962:string[])  [unwired: 8 in, 1 out]
            n1549 = Unbundle By Name(w2942) -> ("Sample holder"=w2943:T20)
            n1550 = Bundle By Name(cluster=w2942, "Desired [G]"=w2940, "Auto-modulation"=TRUE) -> (w2941:T18)
            n1551 = property on="Script Array" class="Arr (strict)"() -> ("Selection Start []"=w2946:u32[])  [unwired: 2 in, 2 out]
            n1552 = local read "Main data folder"() -> (w2944:path)
            n1553 = local write "Acquisition controls"(w2941) -> ()
            n1554 = Index Array(array=w2946) -> (element=w2945:u32)  [unwired: 1 in]
            n1555 = Select(t=experiment_state."Setup", s=w2952, f=experiment_state."Stabilization" ("Value")) -> (s? t:f=w2953:T25)
            n1556 = call "Create measurement file.vi"("Global comment"="Global comment", "Subfolder"=w2944, "Operator"="Operator", "Row"=w2947, "Sample name"="Sample name", "Sample holder"=w2943, "Line index"=w2945, "Create folder with date"="Create folder with date") -> ("Data file ref out"=→"meas results":refnum<file>)  [unwired: 5 in, 2 out]
            n1557 = Bundle By Name(cluster=w2959, "Experiment state"=w2953) -> (w2961:T24)
            "VTI tmp reached" <- FALSE ("VTI tmp reached")
            "Tmp reched time" <- u32 0 ("Tmp reched time")
          }
          frame "Stabilization" {
            n1558 = local read "Piezo controls"() -> (w2973:T15)
            n1559 = Unbundle By Name(w2986) -> ("Rotator.Axes"=w2979:T90, "VTI.VTI [K]"=w2985:dbl, "Magnet.Field [T]"=w2970:dbl)
            n1560 = Unbundle By Name(w2980) -> ("Angle_C"=w2966:refnum<queue>)
            n1561 = Unbundle By Name(w2973) -> ("Axes properties"=w2972:T16[], "Safe to \nmove?"=w2968:bool)
            n1562 = Unbundle By Name(w2988) -> ("Positioners [mm|°]"=w2978:dbl[], "Start"=w2982:dbl, "Tmp [K]"=w2975:dbl, "Wait [min]"=w2984:dbl)
            n1563 = for {
              tunnel: w2979 -> [w3022] mode=indexing
              tunnel: w2978 -> [w3010] mode=indexing
              tunnel: w2972 -> [w3020] mode=indexing
              tunnel: [w3013] -> w2971 mode=indexing
              tunnel: w2968 -> [w3008]
              tunnel: [w3006] -> w2967 mode=indexing
              n1564 = Unbundle By Name(w3020) -> ("MaxErr [µm|m°]"=w3019:dbl)
              n1565 = Unbundle By Name(w3022) -> ("Target"=w3014:bool, "Pos [°]"=w3021:dbl)
              n1566 = Compound Arithmetic op=MULTIPLY(w3019, 2.0 ("value"), 0.001 ("y")) -> (w3017:dbl)
              n1567 = call "Is equal in tolerance.vi"("Absolut tolerance"=w3017, "Reference value"=w3010, "Input value"=w3021) -> ("Is in range"=w3015:bool)  [unwired: 3 in, 1 out]
              n1568 = Less Than 0?(x=w3010) -> (x < 0?=w3007:bool)
              n1569 = And(x=w3014, y=w3015) -> (x .and. y?=w3005:bool)
              n1570 = Or(x=w3007, y=w3005) -> (x .or. y?=w3006:bool)
              n1571 = Select(t=0.0, s=w3005, f=w3010) -> (s? t:f=w3011:dbl)
              n1572 = Bundle By Name(cluster=T42 {"Relative?"=FALSE, "Position [°]"=0.0, "Safe to move?"=TRUE} ("Set position"), "Position [°]"=w3011, "Relative?"=w3005, "Safe to move?"=w3008) -> (w3013:T42)
            }
            n1573 = local read "VTI tmp reached"() -> (w2999:bool)
            n1574 = Less Or Equal To 0?(x=w2975) -> (x <= 0?=w2974:bool)
            n1575 = call "Is equal in tolerance.vi"("Absolut tolerance"=0.5, "Reference value"=w2975, "Input value"=w2985) -> ("Is in range"=w2996:bool)  [unwired: 3 in, 1 out]
            n1576 = Not(x=w2999) -> (.not. x?=w2997:bool)
            n1577 = Or(x=w2974, y=w2996) -> (x .or. y?=w2976:bool)
            n1578 = call "Is equal in tolerance.vi"("Absolut tolerance"=0.001, "Reference value"=w2982, "Input value"=w2970) -> ("Is in range"=w2981:bool)  [unwired: 3 in, 1 out]
            n1579 = And(x=w2976, y=w2997) -> (x .and. y?=w2998:bool)
            n1580 = case shown="False" w2998 {
              tunnel: w2976 -> [w3041 _]
              tunnel: w2984 -> [w3040 w3053]
              tunnel: [w3039 FALSE] -> w2995
              tunnel: [w3038 w3053] -> w2983
              frame False {
                n1581 = case shown="True" w3041 {
                  selector: w3041 -> [w3043 _]
                  tunnel: w3040 -> [w3042 w3048]
                  tunnel: [w3043 w3046] -> w3039
                  tunnel: [w3042 w3044] -> w3038
                  frame False {
                    n1582 = local write "VTI tmp reached"(w3043) -> ()
                  }
                  frame True {
                    n1583 = local read "Tmp reched time"() -> (w3052:dbl)
                    n1584 = Get Date/Time In Seconds() -> (seconds since 1Jan1904=w3045:timestamp)
                    n1585 = To Double Precision Float(number=w3045) -> (double precision float=w3050:dbl)
                    n1586 = Multiply(x=w3048, y=60.0) -> (x*y=w3047:dbl)
                    n1587 = Subtract(x=w3050, y=w3052) -> (x-y=w3049:dbl)
                    n1588 = Subtract(x=w3047, y=w3049) -> (x-y=w3044:dbl)
                    n1589 = Less Or Equal To 0?(x=w3044) -> (x <= 0?=w3046:bool)
                  }
                }
              }
              frame True {
                n1590 = Get Date/Time In Seconds() -> (seconds since 1Jan1904=w3055:timestamp)
                n1591 = To Double Precision Float(number=w3055) -> (double precision float=w3054:dbl)
                n1592 = local write "VTI tmp reached"(TRUE ("VTI tmp reached")) -> ()
                n1593 = local write "Tmp reched time"(w3054) -> ()
              }
            }
            n1594 = And Array Elements(Boolean array=w2967) -> (logical AND=w2969:bool)
            n1595 = case shown="False" w2969 {
              tunnel: w2971 -> [w3002 _]
              tunnel: w2966 -> [w3001 _]
              frame False {
                n1596 = Bundle By Name(cluster=T40 {"Command"=enum."Initialize", "Data"=variant} ("Array"), "Data"=w3002) -> (w3004:T40)
                n1597 = call "Put in mailbox.vi"("Message"=w3004, "Queue in"=w3001) -> ()  [unwired: 7 in, 3 out]
              }
              frame True {
              }
            }
            n1598 = Compound Arithmetic op=AND(w2969, w2981, w2995) -> (w2994:bool)
            n1599 = case shown="True" w2994 {
              tunnel: w2988 -> [w3023 w3027]
              tunnel: w2980 -> [_ w3032]
              tunnel: w2993 -> [w3025 w3035]
              tunnel: [w3025 w3034] -> w2992
              tunnel: [experiment_state."Stabilization" ("Value") w3030] -> w2989
              tunnel: [w3023 w3027] -> w2987
              frame False {
              }
              frame True {
                n1600 = Unbundle By Name(w3027) -> ("Auto-mod"=w3026:bool)
                n1601 = call "Start measurement.vi"("Actual measurement"=w3027, "Referencies in"=w3032) -> ("error out"=w3031:errorcluster)  [unwired: 9 in]
                n1602 = Select(t=experiment_state."Save" ("Value"), s=w3031, f=experiment_state."Begin" ("Value")) -> (s? t:f=w3030:T25)
                n1603 = property on="Auto-modulation" class="Bool (strict)"("Value"=w3026) -> ()  [unwired: 2 in, 2 out]
                n1604 = call "Add actual date time to string.vi"("String in"="Starting measurement") -> ("String out"=w3036:string)  [unwired: 4 in]
                n1605 = call "simple Shift string array.vi"("Element in"=w3036, "Array in"=w3035) -> ("Array out"=w3034:string[])  [unwired: 8 in, 1 out]
                "Running experiment" <- TRUE ("Running experiment")
              }
            }
            n1606 = Bundle By Name(cluster=w2991, "Remains"=w2983, "Experiment state"=w2989) -> (w2990:T24)
          }
          frame "Begin" {
            n1607 = Unbundle By Name(w3059) -> ("Auto-mod"=w3058:bool)
            n1608 = local read "Acquisition controls"() -> (w3061:T18)
            n1609 = Bundle By Name(cluster=w3061, "Auto-modulation"=w3058) -> (w3060:T18)
            n1610 = local write "Acquisition controls"(w3060) -> ()
          }
          frame "Acquisition" {
            n1611 = local read "New data"() -> (w3067:bool)
            n1612 = case shown="True" w3067 {
              selector: w3067 -> [_ w3116]
              tunnel: [FALSE w3128] -> w3075
              tunnel: w3068 -> [_ w3126]
              tunnel: w3066 -> [_ w3121]
              tunnel: w3065 -> [w3077 w3120]
              tunnel: [w3076 w3117] -> w3064
              frame False {
                n1613 = Unbundle By Name(w3077) -> ("Remains"=w3076:dbl)
              }
              frame True {
                n1614 = Not(x=w3116) -> (.not. x?=w3115:bool)
                n1615 = local read "data time"() -> (w3125:timestamp)
                n1616 = Unbundle By Name(w3120) -> ("Started"=w3119:timestamp)
                n1617 = local write "New data"(w3115) -> ()
                n1618 = Unbundle By Name(w3126) -> ("Start"=w3127:dbl, "End"=w3122:dbl)
                n1619 = local read "Data"() -> (w3123:dbl[])
                n1620 = To Double Precision Float(number=w3119) -> (double precision float=w3118:dbl)
                n1621 = To Double Precision Float(number=w3125) -> (double precision float=w3124:dbl)
                n1622 = Unbundle By Name(w3121) -> ("VTI.VTI [K]"=w3080:dbl, "VTI.Sample [K]"=w3094:dbl, "Magnet.Field [T]"=w3087:dbl, "Magnet.Ramp state"=w3096:T9, "Magnet.Ramp [mT/s]"=w3093:dbl)
                n1623 = Index Array(array=w3123) -> (element #1=w3086:dbl, element #2=w3085:dbl)  [unwired: 2 in]
                n1624 = Less?(x=w3127, y=w3122) -> (x < y?=w3099:bool)
                n1625 = Select(t=0.001 ("x"), s=w3099, f=-0.001) -> (s? t:f=w3101:dbl)
                n1626 = Subtract(x=w3124, y=w3118) -> (x-y=w3112:dbl)
                n1627 = Multiply(x=w3101, y=w3093) -> (x*y=w3104:dbl)
                n1628 = Multiply(x=w3112, y=w3104) -> (x*y=w3105:dbl)
                n1629 = Equal?(x=w3096, y=RampingOutput."At Target" ("Magnet.Ramp state")) -> (x = y?=w3097:bool)
                n1630 = Square(x=w3086) -> (x^2=w3083:dbl)
                n1631 = Square(x=w3085) -> (x^2=w3082:dbl)
                n1632 = Add(x=w3105, y=w3127) -> (x+y=w3090:dbl)
                n1633 = Subtract(x=w3090, y=w3122) -> (x-y=w3091:dbl)
                n1634 = local read "Acquisition controls"() -> (w3103:T18)
                n1635 = Add(x=w3083, y=w3082) -> (x+y=w3084:dbl)
                n1636 = Unbundle By Name(w3103) -> ("Modulation [A]"=w3102:dbl)
                n1637 = Absolute Value(x=w3091) -> (abs(x)=w3092:dbl)
                n1638 = Square Root(x=w3084) -> ()  [unwired: 1 out]
                n1639 = call "Is equal in tolerance.vi"("Absolut tolerance"=0.01, "Reference value"=w3122, "Input value"=w3087) -> ("Is in range"=w3114:bool)  [unwired: 1 in]
                n1640 = Divide(x=w3092, y=w3093) -> (x/y=w3089:dbl)
                n1641 = local read "Tab Control"() -> (w3111:T6)
                n1642 = And(x=w3097, y=w3114) -> (x .and. y?=w3128:bool)
                n1643 = call "Add point to array for XY graph.vi"("X-axis"=w3090, "Input A"=w3086, "Input B"=w3085) -> ("Array"=w3107:cluster{"Array":dbl[], "Array":dbl[]}[])  [unwired: 4 in]
                n1644 = local read "SMU controls"() -> (w3081:T14)
                n1645 = Unbundle By Name(w3081) -> ("B[T]"=w3079:dbl)
                n1646 = case shown="\"CW measurement\"" w3111 {
                  tunnel: w3107 -> [_ w3129]
                  frame "Page Status", Default {
                  }
                  frame "CW measurement" {
                    "Spectrum" <- w3129
                  }
                }
                n1647 = local read "meas results"() -> (w3106:refnum<file>)
                n1648 = Build Array(w3090, w3079, w3086, w3085, w3094, w3080, w3102, w3087) -> (w3109:dbl[])
                n1649 = Multiply(x=w3089, y=1000.0) -> (x*y=w3117:dbl)
                n1650 = Array To Spreadsheet String(array=w3109, 3:"%e" ("format string")) -> (spreadsheet string=w3108:string)  [unwired: 1 in]
                n1651 = Write to Text File(file (use dialog)=w3106, text=w3108) -> ()  [unwired: 2 in, 3 out]
              }
            }
            n1652 = Select(t=experiment_state."Save" ("Value"), s=w3075, f=experiment_state."Acquisition" ("Value")) -> (s? t:f=w3069:T25)
            n1653 = Bundle By Name(cluster=w3071, "Experiment state"=w3069, "Remains"=w3064) -> (w3070:T24)
          }
          frame "Save" {
            n1654 = local read "THz control"() -> (w3135:T21)
            n1655 = property on="Script Array" class="Arr (strict)"() -> ("Selection Start []"=w3142:u32[])  [unwired: 2 in, 2 out]
            n1656 = local read "Script Array"() -> (w3158:T26[])
            n1657 = local read "Infobar"() -> (w3146:T24)
            n1658 = local read "Instr status"() -> (w3152:T1)
            n1659 = Index Array(array=w3142) -> (element=w3143:u32)  [unwired: 1 in]
            n1660 = Unbundle By Name(w3135) -> ("AMC"=w3133:u16, "Multip"=w3134:u16)
            n1661 = Increment(x=w3143) -> (x+1=w3155:u32)
            n1662 = Array Size(array=w3158) -> (size(s)=w3156:i32)
            n1663 = local read "Run script btn"() -> (w3150:bool)
            n1664 = Multiply(x=w3133, y=w3134) -> (x*y=w3132:u16)
            n1665 = Array Subset(array=w3158, index=w3155) -> (w3153:T26[])  [unwired: 1 in]
            n1666 = for {
              tunnel: [w3201] -> w3151
              tunnel: w3152 -> [w3203]
              tunnel: [w3202] -> w3148
              tunnel: w3153 -> [w3201] mode=indexing
              tunnel: [w3200] -> w3154
              tunnel: w3132 -> [w3199]
              i -> [w3200]
              stop <- w3202 stop-if-true
              n1667 = call "verify executabiity of line.vi"("Freq multiplication factor"=w3199, "Instr status"=w3203, "Script cluster"=w3201) -> ("is executable"=w3202:bool)  [unwired: 7 in, 1 out]
            }
            n1668 = Greater?(x=w3156, y=w3143) -> (0:w3149:bool)
            n1669 = Compound Arithmetic op=AND(w3150, w3149, w3148) -> (w3147:bool)
            n1670 = Add(x=w3154, y=w3155) -> (x+y=w3145:u32)
            n1671 = local write "Run script btn"(w3147) -> ()
            n1672 = case shown="False" w3147 {
              tunnel: [experiment_state."Setup" ("Value") experiment_state."Preparation" ("Value")] -> w3159
              tunnel: w3144 -> [w3208 _]
              tunnel: w3158 -> [_ _]
              tunnel: [w3208 w3211] -> w3157
              tunnel: w3143 -> [w3205 _]
              tunnel: w3151 -> [_ w3211]
              tunnel: w3146 -> [_ _]
              tunnel: w3145 -> [_ w3210]
              tunnel: [w3205 w3210] -> w3136
              frame False {
                n1673 = local read "Controls referencies"() -> (w3207:T2)
                n1674 = Unbundle By Name(w3207) -> ("To disable"=w3204:refnum<vi>[])
                n1675 = call "Dis- or en- able controls.vi"("Disabled"=T33."Enabled", "Control referencies"=w3204) -> ()  [unwired: 9 in, 1 out]
              }
              frame True {
              }
            }
            n1676 = call "Add point to array for XY graph.vi"("Write?(T)"=FALSE ("Write(T)")) -> ("Array"=w3130:cluster{"Array":dbl[], "Array":dbl[]}[])  [unwired: 6 in]
            n1677 = local write "Spectrum"(w3130) -> ()
            n1678 = local read "meas results"() -> (w3166:refnum<file>)
            n1679 = Close File(refnum=w3166) -> (path=w3139:path)  [unwired: 1 in, 1 out]
            n1680 = case shown="True" "Save also backup" {
              tunnel: w3139 -> [_ w3192]
              tunnel: w3130 -> [_ w3167]
              frame False {
              }
              frame True {
                w3176 = "\t"
                n1681 = Strip Path(path=w3192) -> (stripped path=w3188:path, name=w3191:string)
                n1682 = Concatenate Strings("Backup_", w3191) -> (w3189:string)
                n1683 = Build Path(base path=w3188, name or relative path=w3189) -> (appended path=w3187:path)
                n1684 = Index Array(array=w3167, index #1=0 ("index"), index #2=1 ("index")) -> (element #1=w3183:cluster{"Array":dbl[], "Array":dbl[]}, element #2=w3186:cluster{"Array":dbl[], "Array":dbl[]})
                n1685 = call <vilib>:"Create File with Incrementing Suffix.vi"("file path"=w3187) -> ("error out"=w3168:errorcluster, "refnum out"=w3171:refnum<file>)  [unwired: 8 in, 1 out]
                n1686 = Concatenate Strings("B[T]" ("string"), w3176, "X" ("string"), w3176, "Y", "\r\n") -> (w3173:string)
                n1687 = Unbundle(w3183) -> ("Array"=w3182:dbl[], "Array"=w3181:dbl[])
                n1688 = Unbundle(w3186) -> ("Array"=w3180:dbl[])  [unwired: 1 out]
                n1689 = for {
                  tunnel: w3182 -> [w3194] mode=indexing
                  tunnel: w3181 -> [w3196] mode=indexing
                  tunnel: w3180 -> [w3195] mode=indexing
                  tunnel: [w3197] -> w3174 mode=indexing
                  n1690 = Build Array(w3194, w3196, w3195) -> (w3193:dbl[])
                  n1691 = Array To Spreadsheet String(array=w3193, 3:"%g" ("format string")) -> (spreadsheet string=w3197:string)  [unwired: 1 in]
                }
                n1692 = Concatenate Strings(w3173, w3174) -> (w3172:string)
                n1693 = Write to Text File(file (use dialog)=w3171, text=w3172, error in=w3168) -> (refnum out=w3169:refnum<file>, error out=w3170:errorcluster)  [unwired: 1 in, 1 out]
                n1694 = Close File(refnum=w3169, error in=w3170) -> ()  [unwired: 2 out]
              }
            }
            n1695 = Build Array(w3136) -> (w3137:u32[])
            n1696 = Bundle By Name(cluster=w3161, "Experiment state"=w3159) -> (w3160:T24)
            n1697 = Path To String(path=w3139) -> (string=w3138:string)
            n1698 = property on="Script Array" class="Arr (strict)"("Selection Start []"=w3137) -> ()  [unwired: 2 in, 2 out]
            n1699 = Concatenate Strings("Measurrement finished " ("String in"), w3138) -> (w3140:string)
            n1700 = call "Add actual date time to string.vi"("String in"=w3140) -> ("String out"=w3165:string)  [unwired: 4 in]
            n1701 = call "simple Shift string array.vi"("Element in"=w3165, "Array in"=w3163) -> ("Array out"=w3162:string[])  [unwired: 8 in, 1 out]
          }
        }
      }
      frame "Stop" {
        n1702 = call "simple Shift string array.vi"("Element in"="Program stopped", "Array in"=w3218) -> ("Array out"=w3217:string[])  [unwired: 8 in, 1 out]
      }
      frame "Restart" {
        n1703 = Build Array("Program restarted") -> (w3223:string[])
      }
    }
    n1704 = Tick Count (ms)() -> (millisecond timer value=w20:u32)
    n1705 = Subtract(x=w20, y=w19) -> (x-y=→"round execution\ntime [ms]":u32)
  }
  n1706 = case shown="True" "Operation mode" {
    tunnel: w10 -> [w3235 w3243]
    frame True {
      n1707 = Unbundle By Name(w3235) -> ("Mod_M"=w3228:refnum<queue>, "Field_C"=w3230:refnum<queue>, "MW_C"=w3232:refnum<queue>, "Angle_C"=w3233:refnum<queue>, "Table_C"=w3234:refnum<queue>, "Data_Aq"=w3229:refnum<queue>, "Tmp_C"=w3231:refnum<queue>, "TOP"=w3226:refnum<queue>)
      n1708 = call "TemperatureController main.vi"("Supervising module"=w3226, "Controller module"=w3231) -> ()  [unwired: 10 in]
      n1709 = call "MFLI module main.vi"("Master mailbox"=w3226, "Module mailbox"=w3229) -> ()  [unwired: 10 in]
      n1710 = call "Servo main.vi"("Queue to UI"=w3226, "Module queue servo"=w3234) -> ()  [unwired: 10 in]
      n1711 = call "PiezoController main.vi"("Top"=w3226, "Rotator"=w3233) -> ()  [unwired: 9 in, 1 out]
      n1712 = call "Module for APVSG.vi"("Main controller mailbox"=w3226, "THz module mailbox"=w3232) -> ()  [unwired: 8 in, 2 out]
      n1713 = call "MagnetTop.vi"("Queue to UI"=w3226, "Module queue"=w3230) -> ()  [unwired: 10 in]
      n1714 = call "SMU magnetic field meter.vi"("update time (100ms)"=u32 100, "Mailbox address Top"=w3226, "Module mailbox"=w3228) -> ()  [unwired: 7 in, 2 out]
    }
    frame False {
      n1715 = Unbundle By Name(w3243) -> ("Instr_M"=w3238:refnum<queue>, "Tmp_M"=w3240:refnum<queue>, "MW_C"=w3241:refnum<queue>, "Table_C"=w3242:refnum<queue>, "Tmp_C"=w3237:refnum<queue>, "Field_C"=w3239:refnum<queue>, "TOP"=w3236:refnum<queue>)
      n1716 = call "Fake VTI module.vi"("Top address in"=w3236, "VTI Module ref"=w3239) -> ()  [unwired: 10 in]
      n1717 = call "fake lock-in module.vi"("Master mailbox"=w3236, "Module mailbox"=w3237) -> ()  [unwired: 10 in]
      n1718 = call "fake Servo modue.vi"("Queue to UI"=w3236, "Module queue servo"=w3242) -> ()  [unwired: 10 in]
      n1719 = call "fake SampleRotator module.vi"("Top"=w3236, "Rotator"=w3241) -> ()  [unwired: 8 in, 2 out]
      n1720 = call "fake THz module.vi"("Main controller mailbox"=w3236, "THz module mailbox"=w3240) -> ()  [unwired: 10 in]
      n1721 = call "fake main magnet module.vi"("Queue to UI"=w3236, "Module queue"=w3238) -> ()  [unwired: 10 in]
    }
  }
  n1722 = flat-sequence {
    tunnel: w5 -> [_]
    frame #0 {
      n1723 = Stop(stop? (T)=TRUE) -> ()
    }
  }
